vi "main_scan_4.vi"() -> ()   [LabVIEW 2009]
uses:
  <vilib>/userDefined/High Color/IMAQdx.ctl
  <vilib>/vision/Image Controls.llb/IMAQ Image.ctl
  global_stage_initialised.vi
  <vilib>/vision/driver/IMAQdx.llb/IMAQdx Buffer Number Mode.ctl
  <vilib>/Utility/file.llb/Write To Spreadsheet File (DBL).vi
  <vilib>/vision/driver/NI_Vision_Acquisition_Software.lvlib
  C:/Program Files (x86)/National Instruments/LabVIEW 2009/resource/objmgr/imaqdx.rc
panel:
  in  "Video Mode":u32(ring)=2 items=["Mono 8 1.88 fsp", "Mono 8 3.75 fsp", "Mono 8 7.50 fsp", "Mono 8 15.00 fsp", "Mono 8 30.00 fsp", "Mono 8 60.00 fsp", "Mono 8 120.00 fsp", "Mono 16 1.88 fsp", "Mono 16 3.75 fsp", "Mono 16 7.50 fsp", "Mono 16 15.00 fsp", "Mono 16 30.00 fsp", "Mono 16 60.00 fsp", "Format 7 Mode 0 640x480"]
  out "Vektor Summierte Helligkeit [a.u.]":dbl[](array[numeric])
  out "Vektor L/2-Position [°]":dbl[](array[numeric])
  out "Daten speichern":bool
  out "Leist/Pol # Schleifen":i64
  out "Leistungs-/Polarisationscan läuft":bool
  in  "Max. Spannungsdifferenz":dbl=150.0
  out "Geschätzte Messzeit":string="00:00"
  out "Start time [ms]":timestamp
  out "2D-Intensitätsverteilung (MCP)":dbl[][](graph)
  in  "# Photosignale":i32
  in  "Achs-ID":i32
  in  "Spannungskanal":refnum<k21>
  out "x-U-Scan läuft":bool
  out "Spannungsscan läuft":bool
  out "LAPD Spannung (V)":dbl format="%#.3g"
  out "Summierte Helligkeit (a.u.)":i64
  out "# Messschritte":i32
  out "Aktueller Messschritt":i32
  in  "LAPD-Daten speichern":bool
  in  "Summierte Helligkeit speichern":bool
  in  "Einzelbilder speichern":bool
  in  "Gemittelte Bilder speichern":bool
  in  "# Bilder/Messschritt":i32=1
  in  "SN von Rotationsbühne":i32=83831982
  in  "Wellenplatte [°]":refnum<k7>(container)
  out "Wellenplatte":bool
  in  "Waveplate ON/OFF":bool
  in  "Registerkarte":T1(tab)=enum."Leistungs-/Polarisationsscan"
  out "Aktuelle xyz-Position [mm]":dbl[](array[numeric]) format="%.5g"
  in  "Rasterweite [µm]":dbl[](array[numeric])
  in  "# Rasterschritte":i32[](array[numeric])=[1, 1, 1] min=1 step=1
  in  "Rasterung ON/OFF":bool
  out "Start xyz-Position [mm]":dbl[](array[numeric]) format="%.5g"
  in  "Rasterart":T2(ring)=enum."2D-Scan(xy)"
  out "Rasterschritt [µm]":dbl[](array[numeric])
  out "2D-Intensitätsverteilung (LAPD)":dbl[][](graph)
  out "Spannungsstart [V]":dbl[](array[numeric])
  out "TIP/SUP":string[](array[string])=["Tip", "Suppressor"]
  out "Spannungsschritt [V]":dbl[](array[numeric]) format="%.1g"
  out "Aktuelle Spannung [V]":dbl[](array[numeric]) format="%.1f"
  in  "# Spannungsschritte":i32[](array[numeric])
  in  "Spannungsweite [V]":dbl[](array[numeric])
  in  "Spannungsscan ON/OFF":bool
  out "Schräglage berücksichtigen":string="Schräglage berücksichtigen"
  in  "Ausgleichslage Start festlegen":bool
  out "x-U-Scan (Ausgleichslage) xy-Start [mm]":dbl[](array[numeric]) format="%_5g"
  in  "Raum-Koordinate 2 (Lagenausgleich)":enum16{"x-Achse", "y-Achse", "z-Achse"}(ring)=enum."y-Achse"
  out "x-U-Scan y-Startposition [mm]":dbl format="%.4g"
  out "x-U-Scan aktuelle y-Position [mm]":dbl format="%.4g"
  in  "x-U-Scan (Ausgleichslage) Steigung":dbl format="%_3g"
  out "x-U-Scan Spannungsstart [V]":dbl
  out "x-U-Scan Spannungsschritt [V]":dbl
  out "x-U-Scan aktuelle Spannung [V]":dbl
  in  "# x-U-Scan Spannungsschritte":i32
  in  "x-U-Scan Spannungsweite [V]":dbl
  in  "Raum-Koordinate 1":enum16{"x-Achse", "y-Achse", "z-Achse"}(ring)
  in  "Spannungs-Koordinate":enum16{"Tip-Spannung", "Suppressor-Spannung"}(ring)=2
  in  "x-U-Scan ON/OFF":bool
  in  "x-U-Scan x-Rasterweite [µm]":dbl
  in  "# x-U-Scan x-Rasterschritte":i32
  out "x-U-Scan x-Startposition [mm]":dbl format="%.4g"
  out "x-U-Scan aktuelle x-Position [mm]":dbl format="%.4g"
  out "x-U-Scan x-Rasterschritt [µm]":dbl
  out "x-U-Scan (Ausgleichslage) xy-End [mm]":dbl[](array[numeric]) format="%_5g"
  in  "Ausgleichslage Ende festlegen":bool
  in  "Sättigungszeit [s]":dbl
  in  "Wartezeit [s]":dbl
  in  "Max. Leistung (vK) [mW]":dbl
  out "Aktuelle Leistung (iK) [mW]":dbl
  out "Aktuelle L/2-Position [°]":dbl format="%_3g"
  out "L/2-Schritt [°]":dbl
  in  "Hin und Zurück":bool=TRUE
  in  "# L/2-Schritte":i32
  in  "L/2-Weite [°]":dbl
  in  "L/2-Start [°]":dbl
  in  "Leistuns- oder Polarisationsscan":u16(ring) items=["Polarisationsscan", "Leistungsscan"]
  in  "Leistungs-/Polarisationsscan ON/OFF":bool
  out "1D-Intensitätsverteilung (MCP)":T3(graph)
  out "Vorherige L/2 Position [°]":dbl format="%_3g"
  in  "Hintergrund-Helligkeit":i64
  in  "Helligkeit nullen":bool
  out "Helligkeitsverlauf":dbl(graph)
  in  "Sequenz Ordner":string="Referenzbilder"
  in  "Sequenzaufnahme ON":bool
  in  "MCP-Spannung [V]":dbl=1300.0
  in  "P-Schirm-Spannung [V]":dbl=4300.0
  in  "Proben-ID":string="140528_06"
  out "Messlogbuch":path
  out "Gemitteltes Bild":u64[][](array[numeric])
  in  "Polarisation [°]":dbl=90.0
  out "Current y step":i32
  out "Current z step":i32
  out "Current x step":i32
  out "Scanschleifenzähler":i32
  out "Kameraschleifenzähler":i32
  out "Steuerschleifenzähler":i32
  out "Bühne":bool
  in  "HV ON/OFF":bool
  out "HV-Steuerung":bool
  in  "Suppressor-Spannung [V]":dbl min=0.0 max=1000.0 step=1.0 format="%.1p"
  in  "Tip-Spannung [V]":dbl min=0.0 max=800.0 step=1.0 format="%.1p"
  in  "Leistung (iK) [mW]":dbl format="%.1f"
  in  "LAPD-Kanal (Meilhaus)":u32 max=31
  out "Save folder":string
  out "Buffer Number":u64
  out "ROI table":string[](array[string])=["Breite [px]", "Höhe [px]", "X-Offset [px]", "Y-Offset [px]"]
  in  "Vollbild":bool
  out "Frame Rate (FPS)":dbl format="%#_3g"
  in  "Buffer Interval":u32=1
  out "Ereignis: FrameDone?":refnum<event-registration>
  out "Image Display":T4(plugin-control)
  in  "ROI":i32[](array[numeric])=[640, 480, 0, 0]
  in  "Shutter time (ms)":u16(ring)=3 items=["1000", "500", "200", "100", "50", "20", "10", "1"]
  out "Buffer Overrun":bool
  out "Image Memory":T4
  out "Kamera":bool
  in  "Kamera ON/OFF":bool
  in  "Detektionskamera":T5="cam0"
  out "Day folder":string
  in  "Root folder":string="E:\\GIPES\\Messungen\\"
  out "z-Achse":i32=3
  out "y-Achse":i32=2
  out "x-Achse":i32=1
  out "Event: Rasterung gestartet?":refnum<user-event>
  out "Fehler (Ausgang)":errorcluster
  in  "Programm beenden":bool
  out "Rasterung läuft":bool
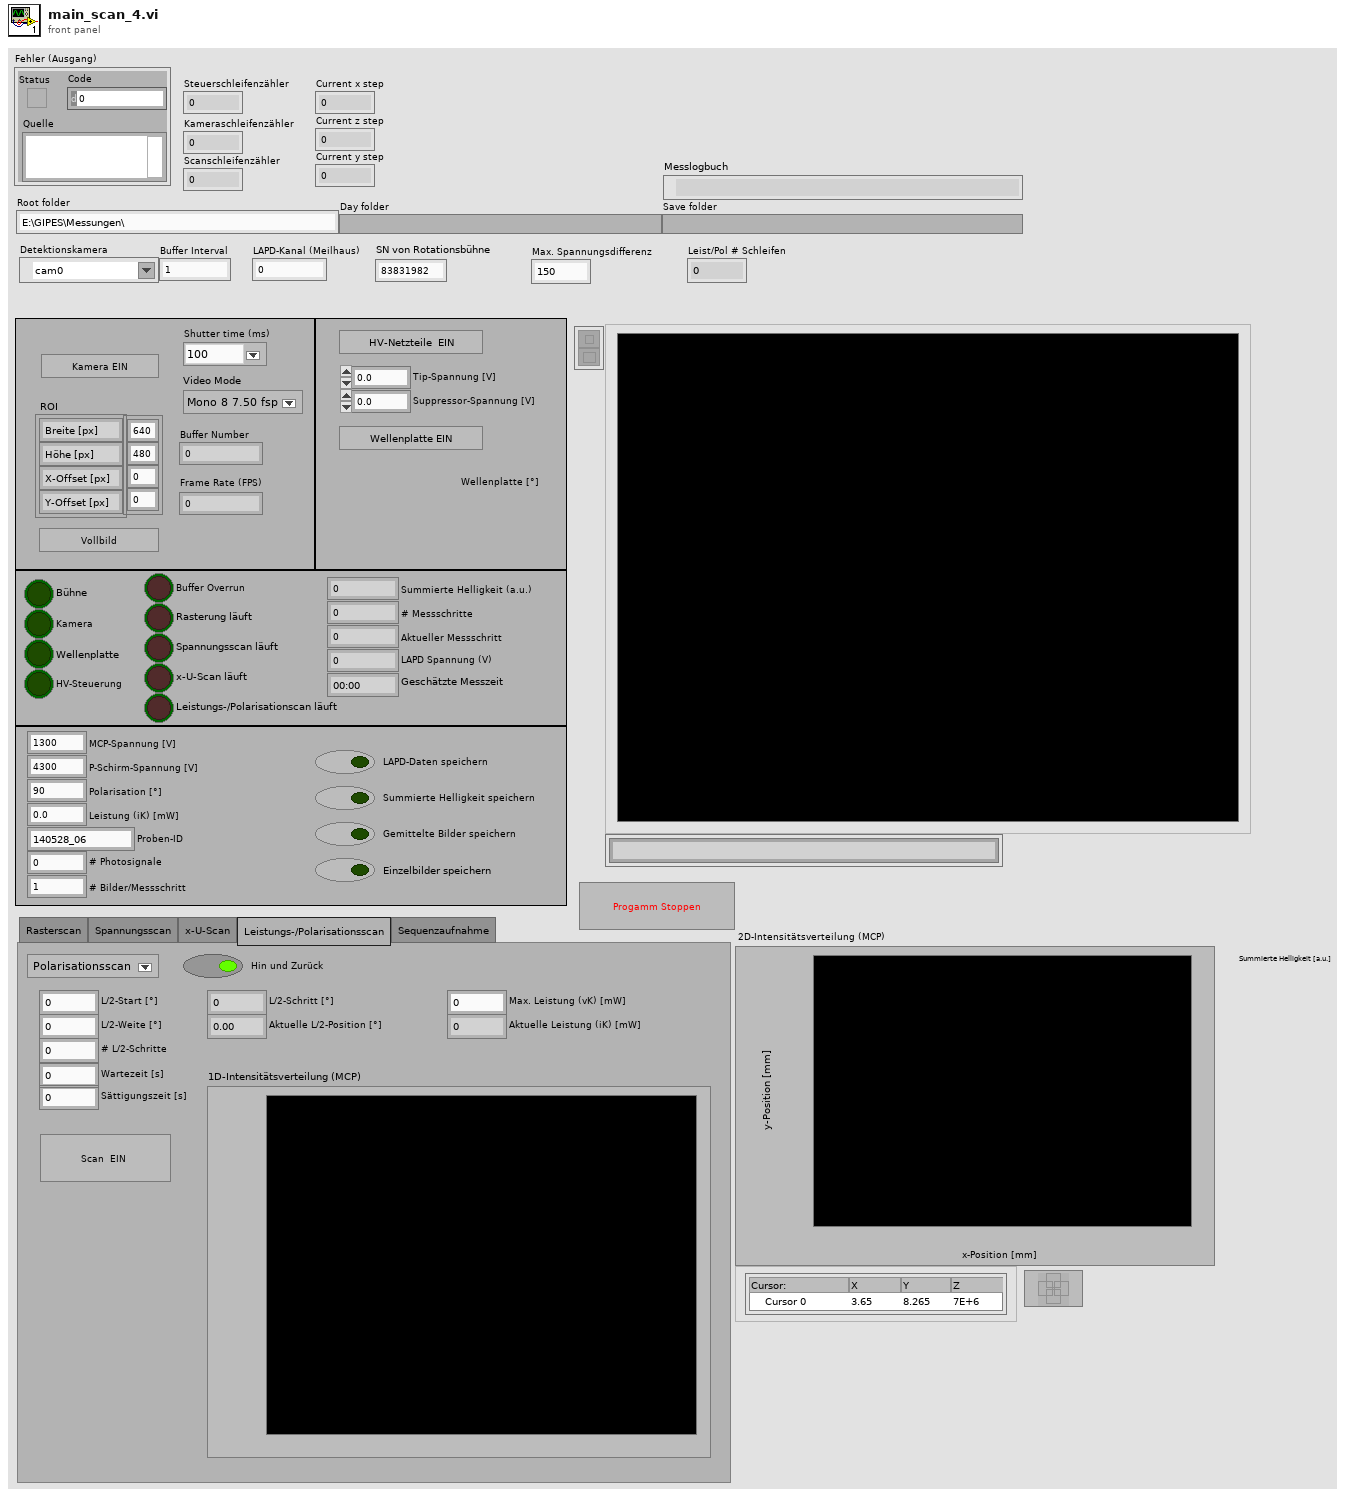
[diagram p1: front panel]
types:
  T1 = enum32{"Rasterscan", "Spannungsscan", "x-U-Scan", "Leistungs-/Polarisationsscan", "Sequenzaufnahme"}
  T2 = enum16{"Linescan(x)", "Linescan(z)", "2D-Scan(xy)", "2D-Scan(yz)", "2D-Scan(xz)"}
  T3 = cluster{"Vektor L/2-Position [°]":dbl[], "Vektor Summierte Helligkeit [a.u.]":dbl[]}
  T4 = typedef "IMAQ Image.ctl" = refnum<image>
  T5 = typedef "IMAQdx.ctl" = refnum<k21>
  T6 = enum32{"Bad", "Idle", "Run top level", "Running"}
  T7 = cluster{"Summierte Helligkeit (a.u.)":u64, "Aktuelle L/2-Position [°]":dbl}
  T8 = typedef "NI_Vision_Acquisition_Software.lvlib/IMAQdx Buffer Number Mode.ctl" = enum32{"Next", "Last", "Buffer Number"}
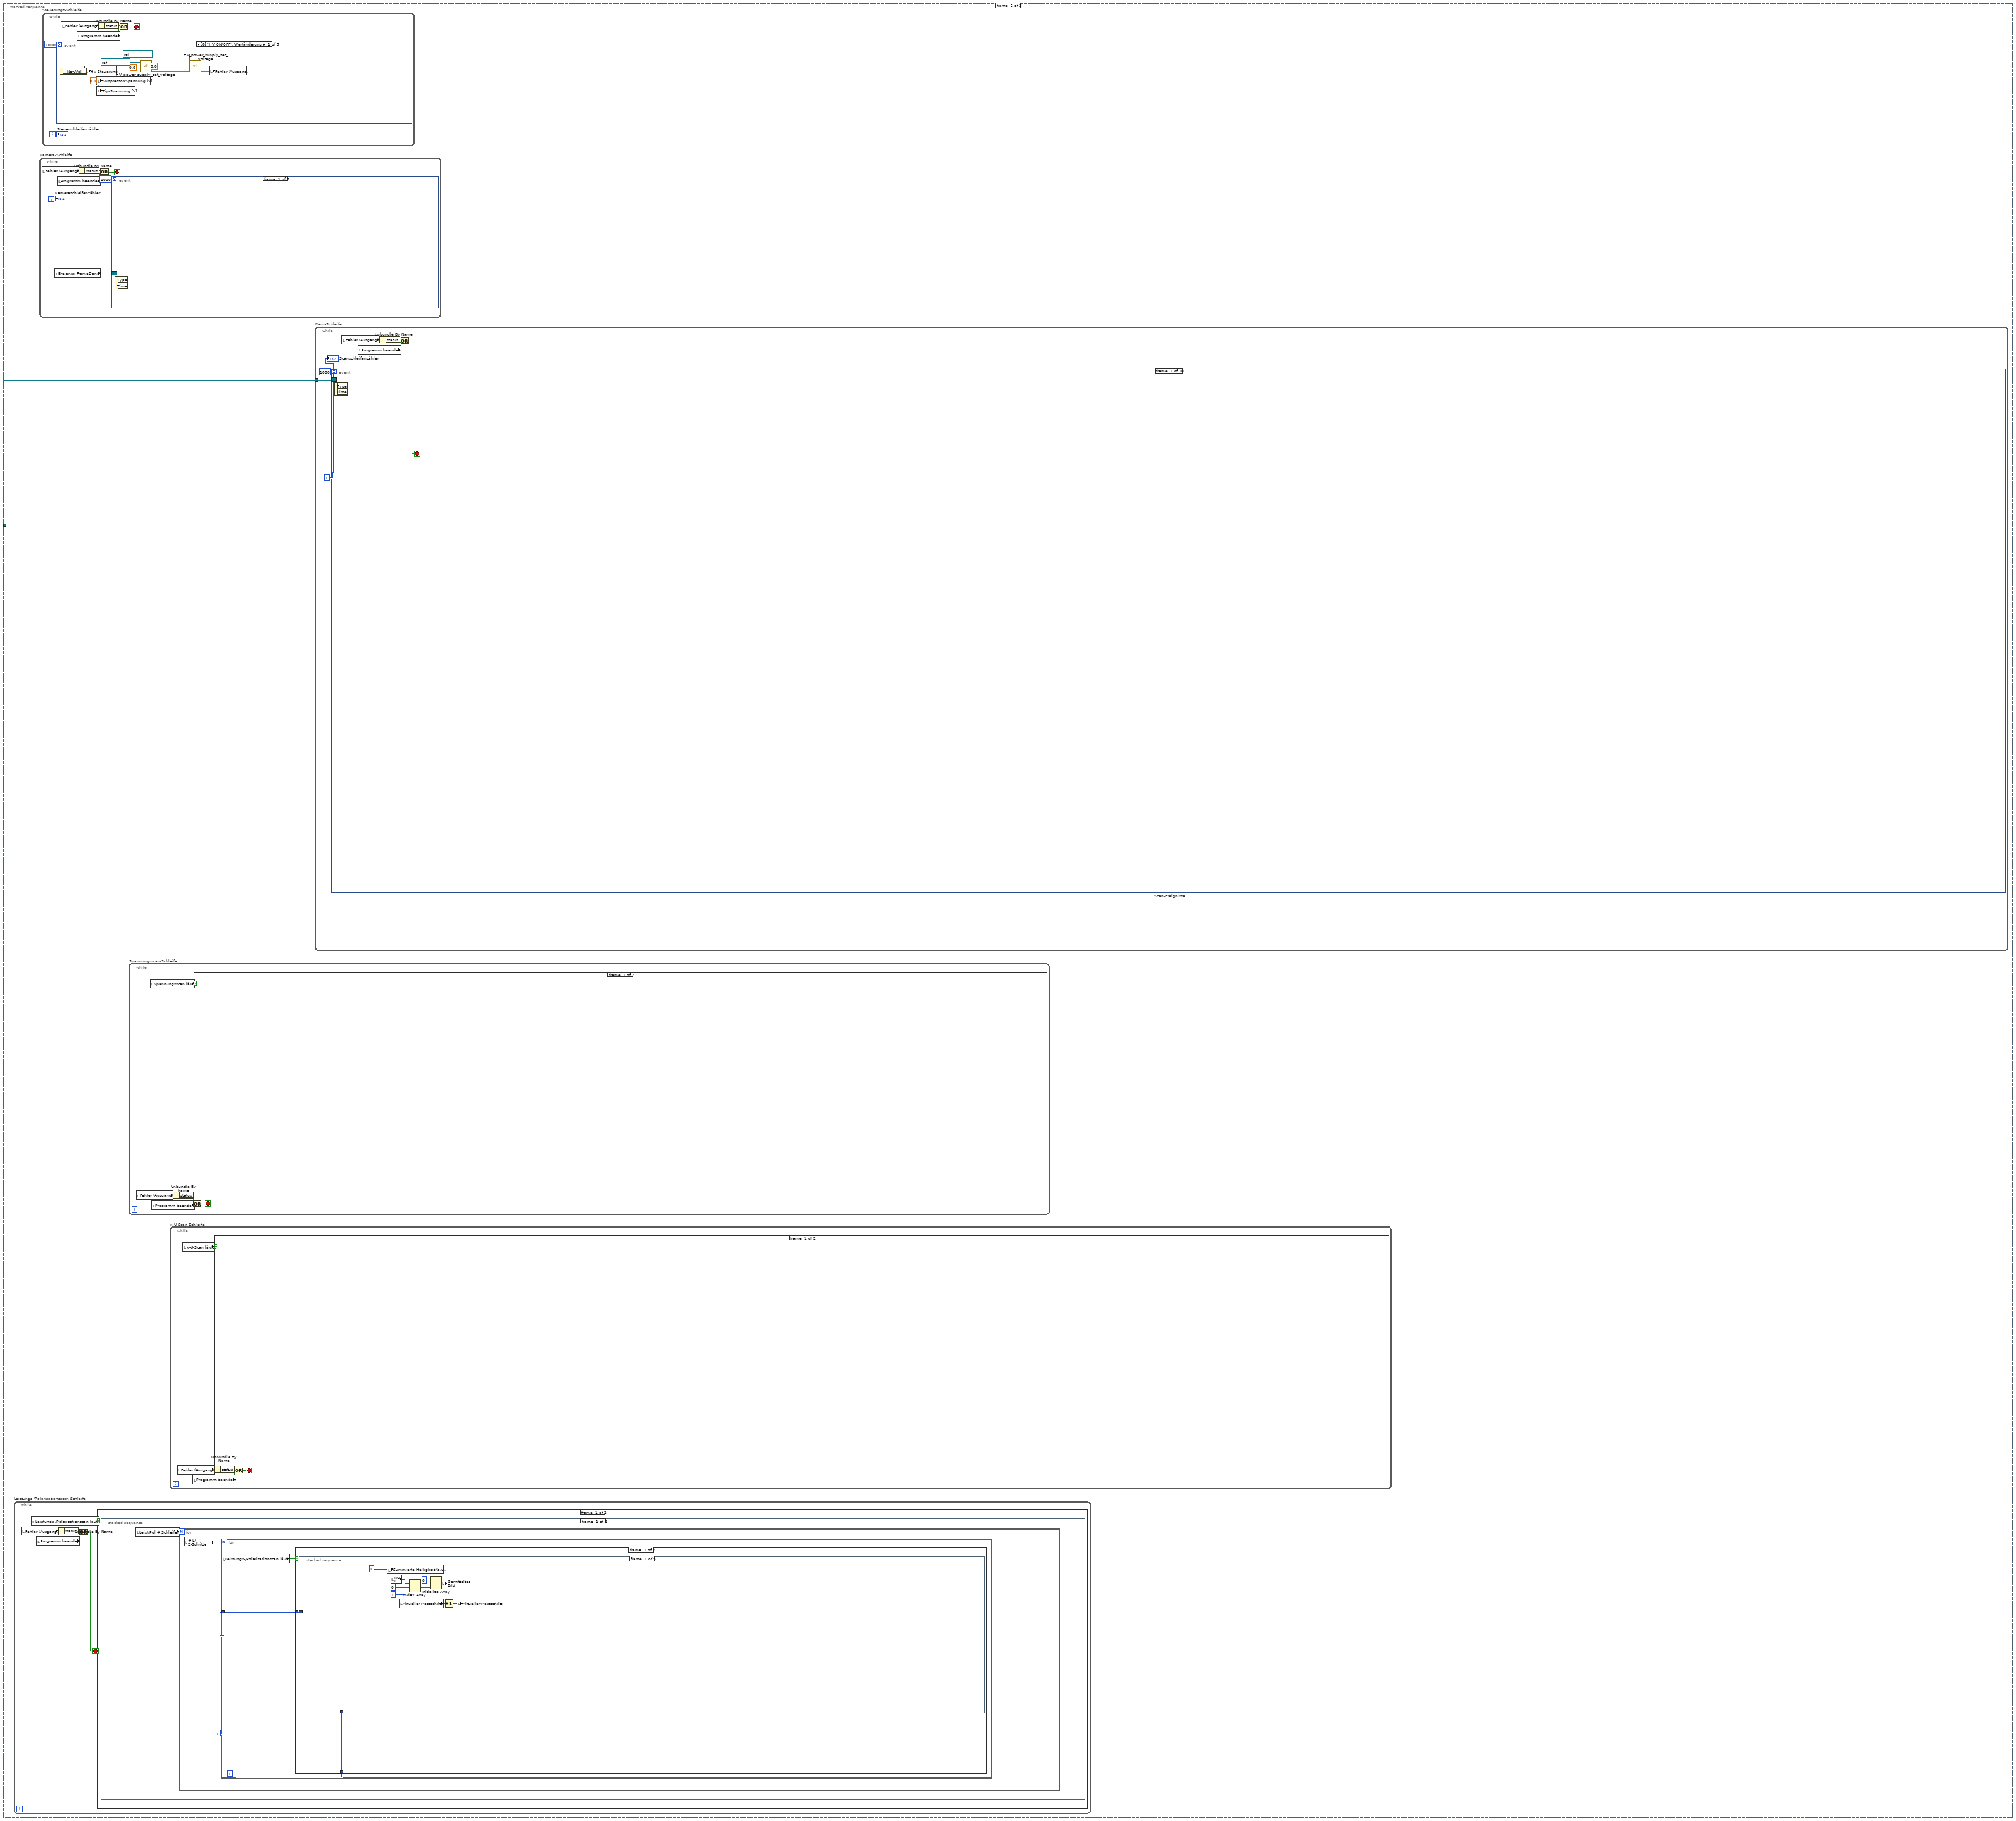
[diagram p3: hidden frame]
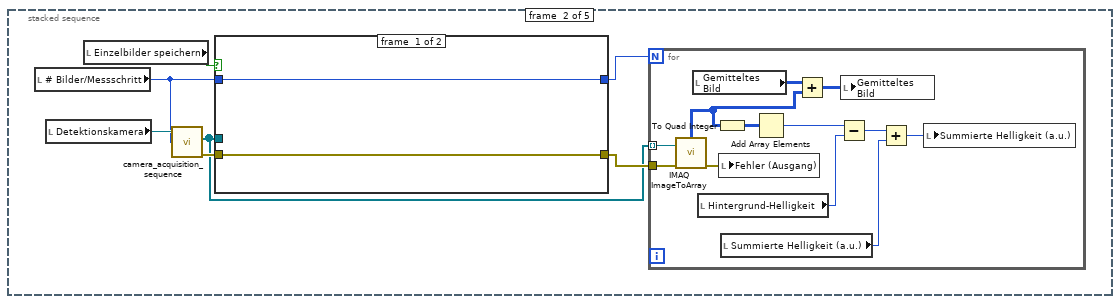
[diagram p4: hidden frame]
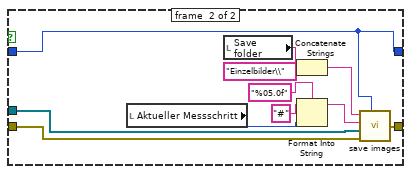
[diagram p5: hidden frame]
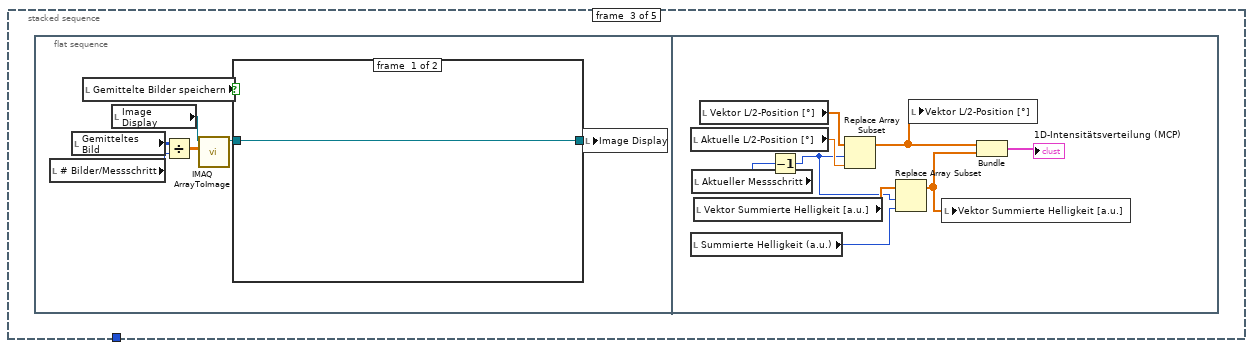
[diagram p6: hidden frame]
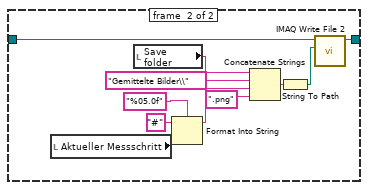
[diagram p7: hidden frame]
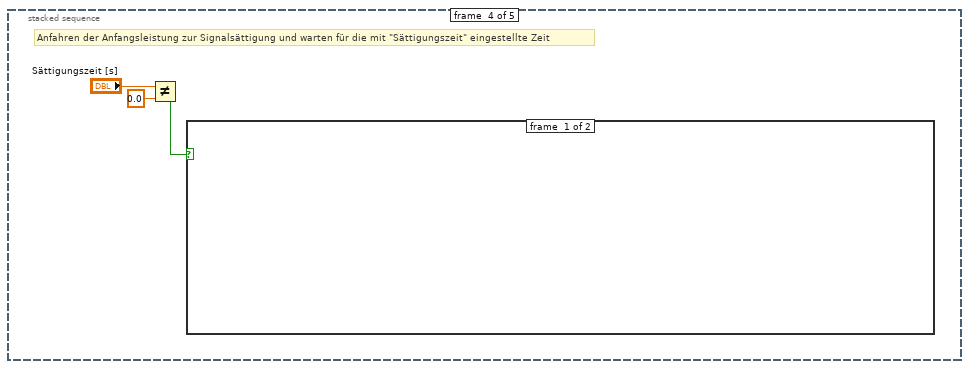
[diagram p8: hidden frame]
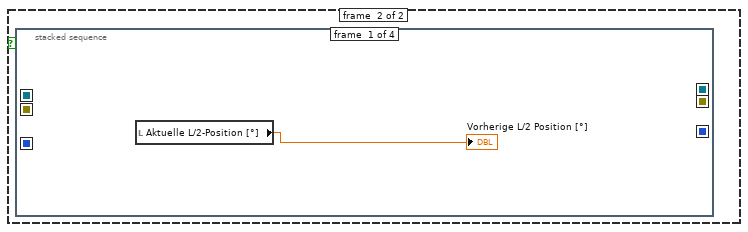
[diagram p9: hidden frame]
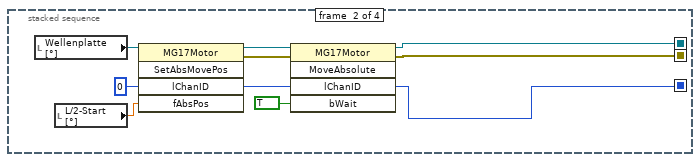
[diagram p10: hidden frame]
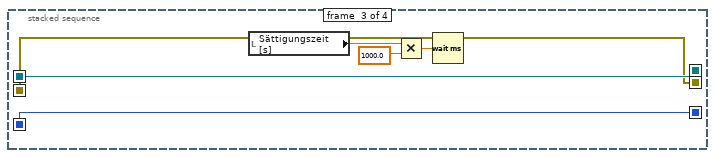
[diagram p11: hidden frame]
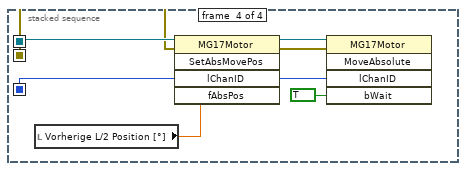
[diagram p12: hidden frame]
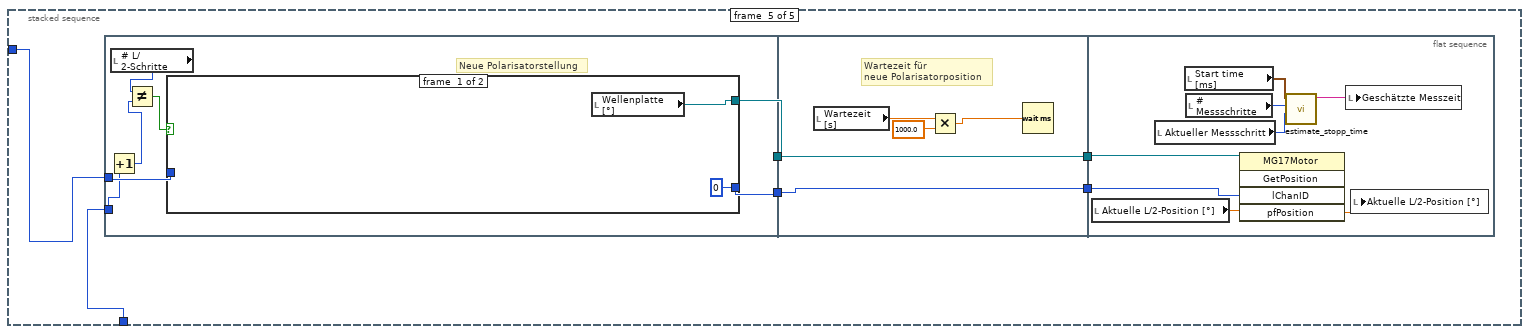
[diagram p13: hidden frame]
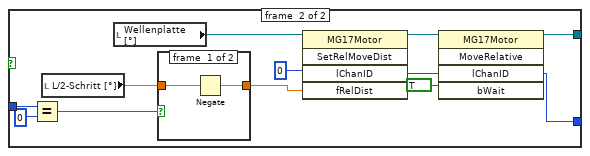
[diagram p14: hidden frame]
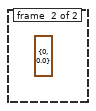
[diagram p16: hidden frame]
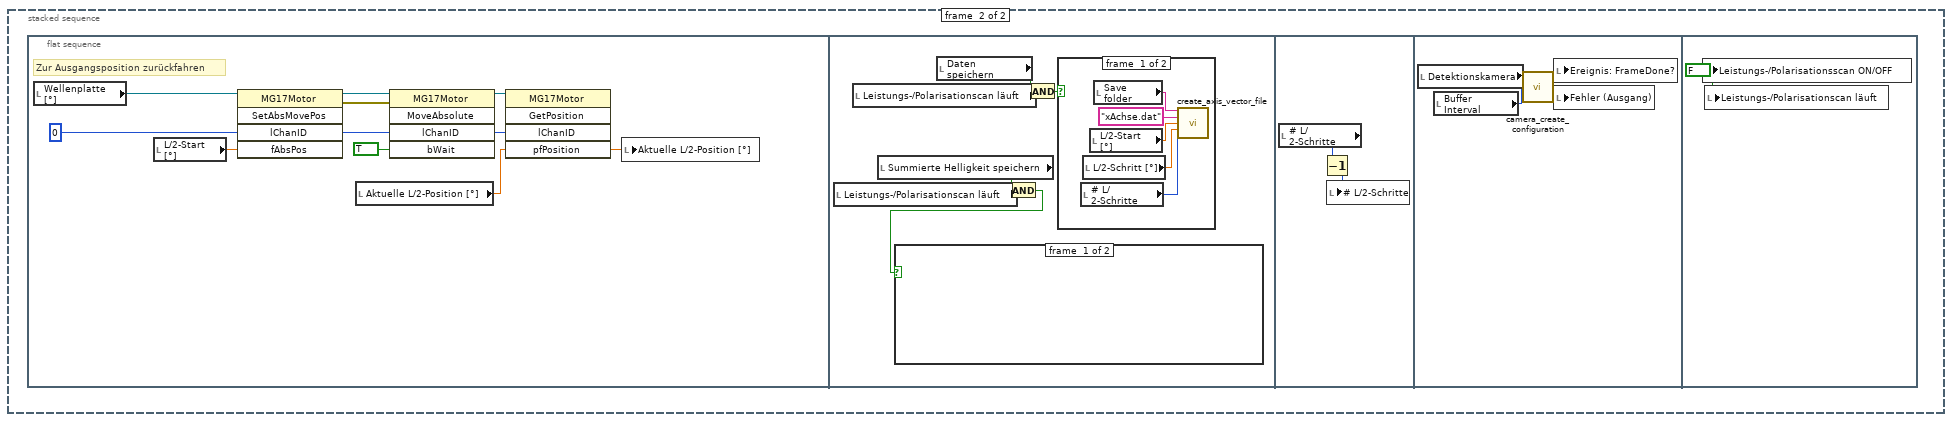
[diagram p17: hidden frame]
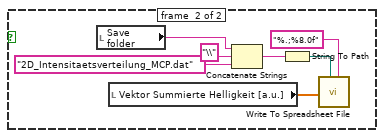
[diagram p18: hidden frame]
diagram:
  n1 = local read "Event: Rasterung gestartet?"() -> (w2:refnum<user-event>)
  n2 = register-events(w2) -> (reference out=w1:refnum<event-registration>)  [unwired: 2 in, 1 out]
  n3 = flat-sequence {
    frame #0 {
      (unwired) 0.0 ("Helligkeitsverlauf")
      w6 = 0.0 ("Aktuelle x-Position [mm]")
      w12 = 1 ("# x-U-Scan Spannungsschritte")
      w13 = 0.0 ("Aktuelle x-Position [mm]")
      w11 = 0.0 ("Suppressor-Spannung [V]")
      w3 = i64 0 ("Numerisches Element")
      w25 = u16 3 items=["1000", "500", "200", "100", "50", "20", "10"] ("Shutter time (ms)")
      w4 = FALSE ("Scanstart")
      n4 = Initialize Array(1 ("Element"), 2 ("Dimension")) -> (w14:i32[])
      n5 = Initialize Array(1 ("Dimension"), 3 ("Dimension")) -> (w37:i32[])
      n6 = Initialize Array(0.0 ("Element"), 2 ("Dimension")) -> (w10:dbl[])
      "Aktuelle Spannung [V]" <- w10
      "Spannungsstart [V]" <- w10
      "x-U-Scan (Ausgleichslage) xy-Start [mm]" <- w10
      "x-U-Scan (Ausgleichslage) xy-End [mm]" <- w10
      n7 = Initialize Array(0.0 ("Element"), 3 ("Dimension")) -> (w20:dbl[])
      "Aktuelle xyz-Position [mm]" <- w20
      "Start xyz-Position [mm]" <- w20
      "Rasterschritt [µm]" <- w20
      n8 = local write "Tip-Spannung [V]"(0.0 ("Tip-Spannung [V]")) -> ()
      n9 = local write "# Photosignale"(10.0 ("Anzahl Mittelungen")) -> ()
      n10 = local write "x-U-Scan x-Rasterweite [µm]"(w11) -> ()
      n11 = local write "# x-U-Scan x-Rasterschritte"(w12) -> ()
      n12 = local write "x-U-Scan Spannungsweite [V]"(w11) -> ()
      n13 = local write "# x-U-Scan Spannungsschritte"(w12) -> ()
      n14 = local write "Suppressor-Spannung [V]"(w11) -> ()
      n15 = local read "Aktueller Messschritt"() -> (w30:i32)
      n16 = local write "Shutter time (ms)"(w25) -> ()
      n17 = local write "# Spannungsschritte"(w14) -> ()
      n18 = local write "Spannungsweite [V]"(w10) -> ()
      n19 = local write "Rasterweite [µm]"(w20) -> ()
      n20 = local write "# Rasterschritte"(w37) -> ()
      n21 = local write "ROI"(i32[] [640, 480, 0, 0] ("Region of Interest (px)")) -> ()
      n22 = local write "x-U-Scan (Ausgleichslage) Steigung"(0.0 ("x-U-Scan (Ausgleichslage) Steigung")) -> ()
      n23 = local write "Spannungsscan ON/OFF"(w4) -> ()
      n24 = local write "Programm beenden"(w4) -> ()
      n25 = local write "Spannungsscan ON/OFF"(w4) -> ()
      n26 = local write "Sequenzaufnahme ON"(w4) -> ()
      n27 = local write "HV ON/OFF"(w4) -> ()
      n28 = local write "x-U-Scan ON/OFF"(w4) -> ()
      n29 = local write "Kamera ON/OFF"(w4) -> ()
      n30 = local write "Rasterung ON/OFF"(w4) -> ()
      n31 = local write "Waveplate ON/OFF"(w4) -> ()
      n32 = local write "Buffer Overrun"(w4) -> ()
      n33 = local write "x-U-Scan läuft"(w4) -> ()
      n34 = local write "Rasterung läuft"(w4) -> ()
      n35 = Create User Event(user event datatype=w30) -> (user event=→"Event: Rasterung gestartet?":refnum<user-event>)  [unwired: 1 in, 1 out]
      n36 = local write "Leistungs-/Polarisationsscan ON/OFF"(w4) -> ()
      n37 = local write "Hintergrund-Helligkeit"(w3) -> ()
      "Rasterung läuft" <- FALSE ("Scan aktiv")
      "# Messschritte" <- 0 ("# Messschritte")
      "Aktueller Messschritt" <- 0 ("Aktueller Messschritt")
      "x-Achse" <- 1 ("x-Achse")
      "y-Achse" <- 2 ("y-Achse")
      "z-Achse" <- 3 ("z-Achse")
      "Summierte Helligkeit (a.u.)" <- w3
      "LAPD Spannung (V)" <- 0.0 ("Transmittierte Intensität (a.u.)")
      "Bühne" <- w4
      "Wellenplatte" <- w4
      "Kamera" <- FALSE ("Camera eingeschaltet")
      "HV-Steuerung" <- w4
      "Spannungsscan läuft" <- w4
      "x-U-Scan aktuelle x-Position [mm]" <- w13
      "x-U-Scan x-Rasterschritt [µm]" <- w13
      "x-U-Scan aktuelle Spannung [V]" <- w13
      "x-U-Scan Spannungsschritt [V]" <- w13
      "x-U-Scan x-Startposition [mm]" <- w13
      "x-U-Scan Spannungsstart [V]" <- w11
      "x-U-Scan aktuelle y-Position [mm]" <- 0.0 ("x-U-Scan aktuelle y-Position [mm]")
      "x-U-Scan y-Startposition [mm]" <- 0.0 ("x-U-Scan y-Startposition [mm]")
      "L/2-Schritt [°]" <- w6
      "Aktuelle L/2-Position [°]" <- w6
      "Aktuelle Leistung (iK) [mW]" <- w6
      "Leistungs-/Polarisationscan läuft" <- w4
      "Leist/Pol # Schleifen" <- i64 1 ("Leist/Pol # Schleifen")
      "Daten speichern" <- w4
    }
  }
  n38 = stacked-sequence {
    tunnel: w1 -> [_ w63 _]
    frame #0 {
      n39 = flat-sequence {
        frame #0 {
          # "Überprüfung ob die VI stage_control.vi ausgeführt wid, wenn nicht wird sie gestartet und gewartet bis die Bühne initialisiert ist"
          n40 = Open VI Reference(vi path=path "stage_control.vi" ("VI-Pfad")) -> (vi reference=w41:refnum<vi>)  [unwired: 5 in, 1 out]
          n41 = property class="VI"(reference=w41) -> (reference out=w40:refnum<vi>, error out=w39:errorcluster, "Exec.State"=w44:T6)  [unwired: 1 in]
          n42 = Equal?(x=w44, y=T6."Run top level") -> (x = y?=w42:bool)
          n43 = case shown="False" w42 {
            tunnel: w40 -> [w51 _]
            tunnel: w39 -> [w50 _]
            frame #0 {
              n44 = invoke class="VI" method="VI ausführen"(reference=w51, error in=w50, "Wait until done"=FALSE ("Warten bis beendet"), "Auto Dispose Ref"=FALSE ("Referenz automatisch schließen")) -> (reference out=w47:refnum<vi>)  [unwired: 1 in, 4 out]
              n45 = invoke class="VI" method="FP.Öffnen"(reference=w47) -> (reference out=w46:refnum<vi>)  [unwired: 4 in, 4 out]
              n46 = while {
                tunnel: w46 -> [w58]
                stop <- w53 stop-if-true
                n47 = property class="VI"(reference=w58) -> (error out=w57:errorcluster, "Exec.State"=w56:T6)  [unwired: 1 in, 1 out]
                n48 = global read "global_stage_initialised.vi" "Bühne initialisiert"() -> (w52:bool)
                n49 = local write "Fehler (Ausgang)"(w57) -> ()
                n50 = Equal?(x=w56, y=T6."Run top level") -> (x = y?=w54:bool)
                n51 = And(x=w52, y=w54) -> (x .and. y?=w53:bool)
              }
            }
            frame #1 {
            }
          }
        }
        frame #1 {
          n52 = local read "Root folder"() -> (w62:string)
          n53 = local write "Bühne"(TRUE ("Bühne bereit")) -> ()
          n54 = call "create_day_folder.vi"("Root folder"=w62) -> ("Day Folder"=w60:string)  [unwired: 9 in, 1 out]
          n55 = local write "Day folder"(w60) -> ()
          n56 = call "create_measure_log_file.vi"("Tagesordner"=w60) -> ("Messlogbuch"=w59:path)  [unwired: 9 in]
          n57 = local write "Messlogbuch"(w59) -> ()
        }
      }
    }
    frame #1 {
      n58 = while "Leistungs-/Polarisationsscan-Schleife" {
        stop <- w65 stop-if-true
        n59 = local read "Fehler (Ausgang)"() -> (w68:errorcluster)
        n60 = local read "Leistungs-/Polarisationscan läuft"() -> (w64:bool)
        n61 = local read "Programm beenden"() -> (w66:bool)
        n62 = Unbundle By Name(w68) -> ("status"=w67:bool)
        n63 = Or(x=w67, y=w66) -> (x .or. y?=w65:bool)
        n64 = case shown="True" w64 {
          frame #0 {
            n65 = stacked-sequence {
              frame #0 {
                n66 = local read "Leist/Pol # Schleifen"() -> (w69:i64)
                n67 = for {
                  N: w69 -> [_]
                  i -> [w70]
                  n68 = local read "# L/2-Schritte"() -> (w71:i32)
                  n69 = for "Schleife für L/2-Position" {
                    N: w71 -> [_]
                    tunnel: w70 -> [w73]
                    i -> [w72]
                    n70 = local read "Leistungs-/Polarisationscan läuft"() -> (w74:bool)
                    n71 = case shown="True" w74 {
                      tunnel: w73 -> [w76 _]
                      tunnel: w72 -> [w75 _]
                      frame #0 {
                        n72 = stacked-sequence {
                          tunnel: w76 -> [_ _ _ _ w180]
                          tunnel: w75 -> [_ _ _ _ w175]
                          frame #0 {
                            n73 = local write "Summierte Helligkeit (a.u.)"(u64 0 ("Summierte Helligkeit (a.u.)")) -> ()
                            n74 = local read "ROI"() -> (w82:i32[])
                            n75 = local read "Aktueller Messschritt"() -> (w79:i32)
                            n76 = Index Array(array=w82, index #1=0 ("Index"), index #2=1 ("Index")) -> (element #1=w86:i32, element #2=w85:i32)
                            n77 = Initialize Array(u64 0 ("Element"), w85, w86) -> (w80:u64[][])
                            n78 = local write "Gemitteltes Bild"(w80) -> ()
                            n79 = Increment(x=w79) -> (x+1=w78:i32)
                            n80 = local write "Aktueller Messschritt"(w78) -> ()
                          }
                          frame #1 {
                            n81 = local read "# Bilder/Messschritt"() -> (w90:i32)
                            n82 = local read "Detektionskamera"() -> (w93:T5)
                            n83 = local read "Einzelbilder speichern"() -> (w88:bool)
                            n84 = call "camera_acquisition_sequence.vi"("Session In"=w93, "Desired image number"=w90) -> ("Image Array"=w87:T4[], "error out"=w92:errorcluster)  [unwired: 2 in, 1 out]
                            n85 = case shown="True" w88 {
                              tunnel: w92 -> [w95 w103]
                              tunnel: [w95 w102] -> w91
                              tunnel: w90 -> [w94 w101]
                              tunnel: [w94 w101] -> w89
                              tunnel: w87 -> [_ w100]
                              frame #0 {
                              }
                              frame #1 {
                                n86 = local read "Aktueller Messschritt"() -> (w106:i32)
                                n87 = local read "Save folder"() -> (w98:string)
                                n88 = Concatenate Strings(w98, "Einzelbilder\\" ("String")) -> (w96:string)
                                n89 = Format Into String(format string="%05.0f" ("Format-String"), initial string="#" ("Eingangs-String"), w106) -> (resulting string=w99:string)  [unwired: 1 in, 1 out]
                                n90 = call "save images.vi"("Save Folder"=w96, "File name prefix"=w99, "Array"=w100, "error out 2"=w103, "Bilder/Messschritt"=w101) -> ("error out"=w102:errorcluster)
                              }
                            }
                            n91 = for {
                              N: w89 -> [_]
                              tunnel: w91 -> [w116]
                              tunnel: w87 -> [w114] mode=indexing
                              n92 = call "IMAQ ImageToArray"("error in (no error)"=w116, "Image"=w114) -> ("error out"=w115:errorcluster, "Image Pixels (U8)"=w113:u8[][])  [unwired: 2 in, 3 out]
                              n93 = local read "Gemitteltes Bild"() -> (w111:u64[][])
                              n94 = local read "Hintergrund-Helligkeit"() -> (w107:i64)
                              n95 = To Quad Integer(1:w113) -> (0:w117:i64[][])
                              n96 = local write "Fehler (Ausgang)"(w115) -> ()
                              n97 = local read "Summierte Helligkeit (a.u.)"() -> (w110:i64)
                              n98 = Add Array Elements(numeric array=w117) -> (sum=w109:i64)
                              n99 = Add(x=w111, y=w113) -> (x+y=w112:u64[][])
                              n100 = Subtract(x=w109, y=w107) -> (x-y=w108:i64)
                              n101 = local write "Gemitteltes Bild"(w112) -> ()
                              n102 = Add(x=w108, y=w110) -> (x+y=w118:i64)
                              n103 = local write "Summierte Helligkeit (a.u.)"(w118) -> ()
                            }
                          }
                          frame #2 {
                            n104 = flat-sequence {
                              frame #0 {
                                n105 = local read "# Bilder/Messschritt"() -> (w121:i32)
                                n106 = local read "Gemitteltes Bild"() -> (w119:u64[][])
                                n107 = local read "Gemittelte Bilder speichern"() -> (w125:bool)
                                n108 = local read "Image Display"() -> (w123:T4)
                                n109 = Divide(x=w119, y=w121) -> (x/y=w120:dbl[][])
                                n110 = call "IMAQ ArrayToImage"("Image Pixels (U8)"=w120, "Image"=w123) -> ("Image Out"=w122:T4)  [unwired: 8 in, 1 out]
                                n111 = case shown="True" w125 {
                                tunnel: w122 -> [w126 w137]
                                tunnel: [w126 w128] -> w124
                                frame #0 {
                                }
                                frame #1 {
                                n112 = local read "Aktueller Messschritt"() -> (w132:i32)
                                n113 = local read "Save folder"() -> (w134:string)
                                n114 = Format Into String(format string="%05.0f" ("Format-String"), initial string="#" ("Eingangs-String"), w132) -> (resulting string=w131:string)  [unwired: 1 in, 1 out]
                                n115 = Concatenate Strings(w134, "Gemittelte Bilder\\" ("String"), w131, ".png" ("String")) -> (w130:string)
                                n116 = String To Path(string=w130) -> (path=w129:path)
                                n117 = call-poly "IMAQ Write File 2"("File Path"=w129, "Image"=w137) -> ("Image Out (duplicate)"=w128:T4)  [unwired: 8 in, 1 out]
                                }
                                }
                                n118 = local write "Image Display"(w124) -> ()
                              }
                              frame #1 {
                                n119 = local read "Aktuelle L/2-Position [°]"() -> (w143:dbl)
                                n120 = local read "Summierte Helligkeit (a.u.)"() -> (w142:i64)
                                n121 = local read "Aktueller Messschritt"() -> (w141:i32)
                                n122 = local read "Vektor Summierte Helligkeit [a.u.]"() -> (w145:dbl[])
                                n123 = local read "Vektor L/2-Position [°]"() -> (w144:dbl[])
                                n124 = Decrement(x=w141) -> (x-1=w140:i32)
                                n125 = Replace Array Subset(array=w144, new element=w143, index=w140) -> (w139:dbl[])
                                n126 = Replace Array Subset(array=w145, new element=w142, index=w140) -> (w138:dbl[])
                                n127 = local write "Vektor L/2-Position [°]"(w139) -> ()
                                n128 = local write "Vektor Summierte Helligkeit [a.u.]"(w138) -> ()
                                n129 = Bundle("Vektor L/2-Position [°]"=w139, "Vektor Summierte Helligkeit [a.u.]"=w138) -> (→"1D-Intensitätsverteilung (MCP)":T3)  [unwired: 1 in]
                              }
                            }
                          }
                          frame #3 {
                            # "Anfahren der Anfangsleistung zur Signalsättigung und warten für die mit \"Sättigungszeit\" eingestellte Zeit"
                            n130 = Not Equal?(x="Sättigungszeit [s]", y=0.0) -> (x != y?=w149:bool)
                            n131 = case shown="True" w149 {
                              frame #0 {
                              }
                              frame #1 {
                                n132 = stacked-sequence {
                                seq-local: [_ w153 _ _] -> [_ _ w163 _]
                                seq-local: [_ w152 _ _] -> [_ _ w162 _]
                                seq-local: [_ w151 _ _] -> [_ _ w161 _]
                                seq-local: [_ _ w163 _] -> [_ _ _ w170]
                                seq-local: [_ _ w162 _] -> [_ _ _ w169]
                                seq-local: [_ _ w161 _] -> [_ _ _ w168]
                                frame #0 {
                                n133 = local read "Aktuelle L/2-Position [°]"() -> (→"Vorherige L/2 Position [°]":dbl)
                                }
                                frame #1 {
                                n134 = local read "Wellenplatte [°]"() -> (w154:refnum<k7>)
                                n135 = local read "L/2-Start [°]"() -> (w160:dbl)
                                n136 = invoke class="MG17Motor" method="SetAbsMovePos"(reference=w154, "lChanID"=0, "fAbsPos"=w160) -> (reference out=w156:refnum<k7>, error out=w159:errorcluster, "lChanID"=w158:i32)  [unwired: 2 in, 2 out]
                                n137 = invoke class="MG17Motor" method="MoveAbsolute"(reference=w156, error in=w159, "lChanID"=w158, "bWait"=TRUE) -> (reference out=w152:refnum<k7>, error out=w151:errorcluster, "lChanID"=w153:i32)  [unwired: 1 in, 2 out]
                                }
                                frame #2 {
                                n138 = local read "Sättigungszeit [s]"() -> (w166:dbl)
                                n139 = Multiply(x=w166, y=1000.0) -> (x*y=w164:dbl)
                                n140 = Wait (ms)(milliseconds to wait=w164) -> ()  [unwired: 1 out]
                                }
                                frame #3 {
                                n141 = local read "Vorherige L/2 Position [°]"() -> (w167:dbl)
                                n142 = invoke class="MG17Motor" method="SetAbsMovePos"(reference=w169, error in=w168, "lChanID"=w170, "fAbsPos"=w167) -> (reference out=w172:refnum<k7>, error out=w174:errorcluster, "lChanID"=w173:i32)  [unwired: 1 in, 2 out]
                                n143 = invoke class="MG17Motor" method="MoveAbsolute"(reference=w172, error in=w174, "lChanID"=w173, "bWait"=TRUE) -> ()  [unwired: 1 in, 5 out]
                                }
                                }
                              }
                            }
                          }
                          frame #4 {
                            n144 = flat-sequence {
                              tunnel: w180 -> [w187]
                              tunnel: [w186] -> w179
                              tunnel: [w185] -> w178
                              tunnel: w175 -> [w184]
                              tunnel: w179 -> [w208]
                              tunnel: w178 -> [w209]
                              tunnel: [w209] -> w177
                              tunnel: [w208] -> w176
                              tunnel: w177 -> [w213]
                              tunnel: w176 -> [w212]
                              frame #0 {
                                # "Neue Polarisatorstellung"
                                n145 = Increment(x=w184) -> (x+1=w183:i32)
                                n146 = local read "# L/2-Schritte"() -> (w182:i32)
                                n147 = Not Equal?(x=w182, y=w183) -> (x != y?=w181:bool)
                                n148 = case shown="True" w181 {
                                tunnel: w187 -> [_ w194]
                                tunnel: [0 ("lChanID") w191] -> w186
                                tunnel: [w189 w190] -> w185
                                frame #0 {
                                n149 = local read "Wellenplatte [°]"() -> (w189:refnum<k7>)
                                }
                                frame #1 {
                                n150 = Equal?(x=w194, y=0) -> (x = y?=w192:bool)
                                n151 = local read "L/2-Schritt [°]"() -> (w196:dbl)
                                n152 = local read "Wellenplatte [°]"() -> (w197:refnum<k7>)
                                n153 = case shown="False" w192 {
                                tunnel: w196 -> [w203 w204]
                                tunnel: [w202 w204] -> w195
                                frame #0 {
                                n154 = Negate(x=w203) -> (-x=w202:dbl)
                                }
                                frame #1 {
                                }
                                }
                                n155 = invoke class="MG17Motor" method="SetRelMoveDist"(reference=w197, "lChanID"=0, "fRelDist"=w195) -> (reference out=w199:refnum<k7>, "lChanID"=w200:i32)  [unwired: 2 in, 3 out]
                                n156 = invoke class="MG17Motor" method="MoveRelative"(reference=w199, "lChanID"=w200, "bWait"=TRUE) -> (reference out=w190:refnum<k7>, "lChanID"=w191:i32)  [unwired: 2 in, 3 out]
                                }
                                }
                              }
                              frame #1 {
                                # "Wartezeit für\nneue Polarisatorposition"
                                n157 = local read "Wartezeit [s]"() -> (w206:dbl)
                                n158 = Multiply(x=w206, y=1000.0) -> (x*y=w205:dbl)
                                n159 = Wait (ms)(milliseconds to wait=w205) -> ()  [unwired: 1 out]
                              }
                              frame #2 {
                                n160 = local read "Aktuelle L/2-Position [°]"() -> (w210:dbl)
                                n161 = local read "Aktueller Messschritt"() -> (w215:i32)
                                n162 = local read "Start time [ms]"() -> (w217:timestamp)
                                n163 = local read "# Messschritte"() -> (w216:i32)
                                n164 = invoke class="MG17Motor" method="GetPosition"(reference=w213, "lChanID"=w212, "pfPosition"=w210) -> ("pfPosition"=w211:sgl)  [unwired: 2 in, 4 out]
                                n165 = call "estimate_stopp_time.vi"("Aktueller Messschritt"=w215, "# Messschritte"=w216, "Startzeit"=w217) -> ("Stopp Zeit"=w214:string)  [unwired: 8 in]
                                n166 = local write "Geschätzte Messzeit"(w214) -> ()
                                n167 = local write "Aktuelle L/2-Position [°]"(w211) -> ()
                              }
                            }
                          }
                        }
                      }
                      frame #1 {
                        (unwired) T7 {"Summierte Helligkeit (a.u.)"=0, "Aktuelle L/2-Position [°]"=0.0}
                      }
                    }
                  }
                }
              }
              frame #1 {
                n168 = flat-sequence {
                  frame #0 {
                    # "Zur Ausgangsposition zurückfahren"
                    n169 = local read "Wellenplatte [°]"() -> (w228:refnum<k7>)
                    n170 = local read "L/2-Start [°]"() -> (w222:dbl)
                    n171 = invoke class="MG17Motor" method="SetAbsMovePos"(reference=w228, "lChanID"=0, "fAbsPos"=w222) -> (reference out=w226:refnum<k7>, error out=w223:errorcluster, "lChanID"=w224:i32)  [unwired: 2 in, 2 out]
                    n172 = local read "Aktuelle L/2-Position [°]"() -> (w220:dbl)
                    n173 = invoke class="MG17Motor" method="MoveAbsolute"(reference=w226, error in=w223, "lChanID"=w224, "bWait"=TRUE) -> (reference out=w219:refnum<k7>, "lChanID"=w218:i32)  [unwired: 1 in, 3 out]
                    n174 = invoke class="MG17Motor" method="GetPosition"(reference=w219, "lChanID"=w218, "pfPosition"=w220) -> ("pfPosition"=w221:sgl)  [unwired: 2 in, 4 out]
                    n175 = local write "Aktuelle L/2-Position [°]"(w221) -> ()
                  }
                  frame #1 {
                    n176 = local read "Leistungs-/Polarisationscan läuft"() -> (w231:bool)
                    n177 = local read "Leistungs-/Polarisationscan läuft"() -> (w233:bool)
                    n178 = local read "Summierte Helligkeit speichern"() -> (w230:bool)
                    n179 = local read "Daten speichern"() -> (w234:bool)
                    n180 = And(x=w230, y=w231) -> (x .and. y?=w229:bool)
                    n181 = case shown="True" w229 {
                      frame #0 {
                      }
                      frame #1 {
                        n182 = local read "Save folder"() -> (w235:string)
                        n183 = local read "Vektor Summierte Helligkeit [a.u.]"() -> (w236:dbl[])
                        n184 = Concatenate Strings(w235, "\\" ("String"), "2D_Intensitaetsverteilung_MCP.dat" ("String")) -> (w240:string)
                        n185 = String To Path(string=w240) -> (path=w239:path)
                        n186 = call-poly <vilib>:"Write To Spreadsheet File.vi"("format (%.3f)"="%.;%8.0f", "1D data"=w236, "file path (dialog if empty)"=w239) -> ()  [unwired: 5 in, 1 out]
                      }
                    }
                    n187 = And(x=w234, y=w233) -> (x .and. y?=w232:bool)
                    n188 = case shown="True" w232 {
                      frame #0 {
                        n189 = local read "# L/2-Schritte"() -> (w244:i32)
                        n190 = local read "L/2-Schritt [°]"() -> (w243:dbl)
                        n191 = local read "L/2-Start [°]"() -> (w242:dbl)
                        n192 = local read "Save folder"() -> (w245:string)
                        n193 = call "create_axis_vector_file.vi"("Save folder"=w245, "Dateiname"="xAchse.dat", "Start"=w242, "Schrittlänge"=w243, "# Schritte"=w244) -> ()  [unwired: 11 in]
                      }
                      frame #1 {
                      }
                    }
                  }
                  frame #2 {
                    n194 = local read "# L/2-Schritte"() -> (w248:i32)
                    n195 = Decrement(x=w248) -> (x-1=w247:i32)
                    n196 = local write "# L/2-Schritte"(w247) -> ()
                  }
                  frame #3 {
                    n197 = local read "Detektionskamera"() -> (w250:T5)
                    n198 = local read "Buffer Interval"() -> (w251:u32)
                    n199 = call "camera_create_configuration.vi"("BufferInterval"=w251, "Session Out 2"=w250) -> ("Fehler (Ausgang)"=w252:errorcluster, "Ereignisregistrierung (Referenz)"=w249:refnum<event-registration>)  [unwired: 1 in, 1 out]
                    n200 = local write "Ereignis: FrameDone?"(w249) -> ()
                    n201 = local write "Fehler (Ausgang)"(w252) -> ()
                  }
                  frame #4 {
                    w253 = FALSE ("Spannungsscan läuft")
                    n202 = local write "Leistungs-/Polarisationsscan ON/OFF"(w253) -> ()
                    n203 = local write "Leistungs-/Polarisationscan läuft"(w253) -> ()
                  }
                }
              }
            }
          }
          frame #1 {
          }
        }
      }
      n204 = while "Kamera-Schleife" {
        i -> [w1624]
        stop <- w1625 stop-if-true
        n205 = local read "Fehler (Ausgang)"() -> (w1626:errorcluster)
        n206 = local read "Ereignis: FrameDone?"() -> (w1629:refnum<event-registration>)
        n207 = local read "Programm beenden"() -> (w1628:bool)
        n208 = Unbundle By Name(w1626) -> ("status"=w1627:bool)
        n209 = Or(x=w1627, y=w1628) -> (x .or. y?=w1625:bool)
        n210 = event "Kamera-Ereignisse" shown="[3] \"Helligkeit nullen\": Wertänderung" {
          selector: w1629 -> [_ _ _ _ _ _ _ _]
          dyn-events: _ -> [_ _ _ _ _ _ _ _]
          timeout: 1000 -> [_ _ _ _ _ _ _ _]
          event #0 {
            n211 = event-data() -> ()  [unwired: 1 in, 2 out]
          }
          event #1 {
            n212 = event-data() -> ()  [unwired: 1 in, 4 out]
            n213 = local read "Detektionskamera"() -> (w1632:T5)
            n214 = local read "Kamera ON/OFF"() -> (w1633:bool)
            n215 = case shown="True" w1633 {
              tunnel: w1632 -> [w1634 w1640]
              tunnel: [w1637 w1641] -> w1631
              frame #0 {
                n216 = local read "Image Memory"() -> (w1635:T4)
                n217 = call "camera_release configuration_stop.vi"("Image Memory"=w1635, "Detektionskamera"=w1634) -> ("error out"=w1637:errorcluster, "status"=w1636:bool)
                n218 = local write "Kamera"(w1636) -> ()
              }
              frame #1 {
                n219 = local read "Buffer Interval"() -> (w1639:u32)
                n220 = local read "Video Mode"() -> (w1638:u32)
                n221 = call "camera_acquisition_continously.vi"("Detektionskamera"=w1640, "BufferInterval"=w1639, "Video Mode"=w1638) -> ("Kamera eingeschaltet?"=w1645:bool, "Detektionskamera"=w1644:T5, "Image Memory"=w1643:T4, "Ereignis: FrameDone?"=w1642:refnum<event-registration>, "error out"=w1641:errorcluster)  [unwired: 1 in]
                n222 = local write "Image Memory"(w1643) -> ()
                n223 = local write "Detektionskamera"(w1644) -> ()
                n224 = local write "Ereignis: FrameDone?"(w1642) -> ()
                n225 = local write "Kamera"(w1645) -> ()
              }
            }
            n226 = local write "Fehler (Ausgang)"(w1631) -> ()
          }
          event #2 {
            w1660 = IMAQdx_Buffer_Number_Mode."Buffer Number"  # Buffer Number Mode
            n227 = event-data() -> ("ActualBufferNumber"=w1654:u32)  [unwired: 1 in]
            n228 = local read "Detektionskamera"() -> (w1659:T5)
            n229 = local read "Image Memory"() -> (w1658:T4)
            n230 = call <vilib>:"IMAQdx Get Image.vi"("Buffer Number Mode (Next)"=w1660, "Buffer Number In"=w1654, "Image In"=w1658, "Session In"=w1659) -> ("error out"=w1652:errorcluster, "Buffer Number Out"=w1655:u32, "Image Out"=w1651:T4, "Session Out"=w1656:T5)  [unwired: 1 in, 3 out]
            n231 = local write "Image Memory"(w1651) -> ()
            n232 = local write "Detektionskamera"(w1656) -> ()
            n233 = local write "Image Display"(w1651) -> ()
            n234 = local write "Buffer Number"(w1655) -> ()
            n235 = local write "Fehler (Ausgang)"(w1652) -> ()
            n236 = Not Equal?(x=w1655, y=w1654) -> (x != y?=w1653:bool)
            n237 = call "IMAQ ImageToArray"("Image"=w1651) -> ("Image Pixels (U8)"=w1648:u8[][])  [unwired: 3 in, 4 out]
            n238 = call "CalculateFPS.vi"("buffer number"=w1655) -> ("processed FPS"=w1657:dbl)  [unwired: 2 out]
            n239 = To Quad Integer(1:w1648) -> (0:w1647:i64[][])
            n240 = local write "Buffer Overrun"(w1653) -> ()
            n241 = local write "Frame Rate (FPS)"(w1657) -> ()
            n242 = Add Array Elements(numeric array=w1647) -> (sum=w1650:i64)
            n243 = local read "Hintergrund-Helligkeit"() -> (w1646:i64)
            n244 = Subtract(x=w1650, y=w1646) -> (x-y=w1649:i64)
            n245 = local write "Summierte Helligkeit (a.u.)"(w1649) -> ()
            n246 = local write "Helligkeitsverlauf"(w1649) -> ()
          }
          event #3 {
            n247 = event-data() -> ()  [unwired: 1 in, 2 out]
            n248 = case shown="True" "Helligkeit nullen" {
              frame #0 {
              }
              frame #1 {
                n249 = local read "Summierte Helligkeit (a.u.)"() -> (w1662:i64)
                n250 = local write "Hintergrund-Helligkeit"(w1662) -> ()
              }
            }
          }
          event #4 {
            n251 = event-data() -> ()  [unwired: 1 in, 2 out]
            n252 = local read "Kamera"() -> (w1663:bool)
            n253 = case shown="True" w1663 {
              frame #0 {
              }
              frame #1 {
                n254 = control-ref of="Shutter time (ms)"() -> (w1670:refnum<vi>)
                n255 = property class="Ring (strikt)"(reference=w1670) -> ("RingText.Text"=w1669:string)  [unwired: 1 in, 2 out]
                n256 = local read "Detektionskamera"() -> (w1668:T5)
                n257 = Decimal String To Number(string=w1669) -> (number=w1665:i32)  [unwired: 2 in, 1 out]
                n258 = property class="IMAQdx"(reference=w1668, "ActiveAttribute"="CameraAttributes::Shutter::Value", "ValueDBL"=w1665) -> (reference out=w1667:T5, error out=w1664:errorcluster)  [unwired: 1 in]
                n259 = local write "Detektionskamera"(w1667) -> ()
                n260 = local write "Fehler (Ausgang)"(w1664) -> ()
              }
            }
          }
          event #5 {
            n261 = event-data() -> ()  [unwired: 1 in, 1 out]
            n262 = local read "Kamera ON/OFF"() -> (w1671:bool)
            n263 = case shown="True" w1671 {
              frame #0 {
              }
              frame #1 {
                n264 = flat-sequence {
                  frame #0 {
                    n265 = local read "Detektionskamera"() -> (w1672:T5)
                    n266 = local read "Image Memory"() -> (w1673:T4)
                    n267 = call "camera_release configuration_stop.vi"("Image Memory"=w1673, "Detektionskamera"=w1672) -> ("status"=w1674:bool)  [unwired: 1 out]
                    n268 = local write "Kamera"(w1674) -> ()
                  }
                  frame #1 {
                    n269 = local read "Detektionskamera"() -> (w1675:T5)
                    n270 = control-ref of="Shutter time (ms)"() -> (w1678:refnum<vi>)
                    n271 = property class="Ring (strikt)"(reference=w1678) -> ("RingText.Text"=w1677:string)  [unwired: 1 in, 2 out]
                    n272 = local read "Buffer Interval"() -> (w1681:u32)
                    n273 = local read "Video Mode"() -> (w1680:u32)
                    n274 = Decimal String To Number(string=w1677) -> (number=w1676:i32)  [unwired: 2 in, 1 out]
                    n275 = call "camera_acquisition_continously.vi"("Detektionskamera"=w1675, "BufferInterval"=w1681, "Video Mode"=w1680, "Shutter time (ms)"=w1676) -> ("Kamera eingeschaltet?"=w1685:bool, "Detektionskamera"=w1684:T5, "Image Memory"=w1683:T4, "Ereignis: FrameDone?"=w1682:refnum<event-registration>, "error out"=w1679:errorcluster)
                    n276 = local write "Image Memory"(w1683) -> ()
                    n277 = local write "Detektionskamera"(w1684) -> ()
                    n278 = local write "Ereignis: FrameDone?"(w1682) -> ()
                    n279 = local write "Fehler (Ausgang)"(w1679) -> ()
                    n280 = local write "Kamera"(w1685) -> ()
                  }
                }
              }
            }
          }
          event #6 {
            n281 = event-data() -> ()  [unwired: 1 in, 1 out]
            n282 = local read "Kamera"() -> (w1686:bool)
            n283 = case shown="True" w1686 {
              frame #0 {
              }
              frame #1 {
                n284 = local read "Ereignis: FrameDone?"() -> (w1688:refnum<event-registration>)
                n285 = local read "Detektionskamera"() -> (w1692:T5)
                n286 = local read "Buffer Interval"() -> (w1691:u32)
                n287 = local read "ROI"() -> (w1693:i32[])
                n288 = call "camera_change_ROI.vi"("BufferInterval"=w1691, "Region of Interest"=w1693, "Ereignisregistrierung (Referenz) 2"=w1688, "Session In"=w1692) -> ("Fehler (Ausgang)"=w1687:errorcluster, "Ereignisregistrierung (Referenz)"=w1690:refnum<event-registration>, "Session Out"=w1689:T5)  [unwired: 5 in]
                n289 = local write "Detektionskamera"(w1689) -> ()
                n290 = local write "Ereignis: FrameDone?"(w1690) -> ()
                n291 = local write "Fehler (Ausgang)"(w1687) -> ()
              }
            }
          }
          event #7 {
            n292 = event-data() -> ("NewVal"=w1695:bool)  [unwired: 1 in, 1 out]
            n293 = local read "Kamera"() -> (w1696:bool)
            n294 = And(x=w1696, y=w1695) -> (x .and. y?=w1694:bool)
            n295 = case shown="True" w1694 {
              frame #0 {
              }
              frame #1 {
                w1697 = i32[] [640, 480, 0, 0] ("Region of Interest (px)")
                n296 = local read "Ereignis: FrameDone?"() -> (w1699:refnum<event-registration>)
                n297 = local read "Detektionskamera"() -> (w1703:T5)
                n298 = local read "Buffer Interval"() -> (w1702:u32)
                n299 = call "camera_change_ROI.vi"("BufferInterval"=w1702, "Region of Interest"=w1697, "Ereignisregistrierung (Referenz) 2"=w1699, "Session In"=w1703) -> ("Fehler (Ausgang)"=w1698:errorcluster, "Ereignisregistrierung (Referenz)"=w1701:refnum<event-registration>, "Session Out"=w1700:T5)  [unwired: 5 in]
                n300 = local write "ROI"(w1697) -> ()
                n301 = local write "Detektionskamera"(w1700) -> ()
                n302 = local write "Ereignis: FrameDone?"(w1701) -> ()
                n303 = local write "Fehler (Ausgang)"(w1698) -> ()
              }
            }
          }
        }
        "Kameraschleifenzähler" <- w1624
      }
      n304 = while "Steuerungs-Schleife" {
        i -> [w614]
        stop <- w613 stop-if-true
        n305 = event shown="[0] \"HV ON/OFF\": Wertänderung" {
          selector: _ -> [_ _ _ _ _]
          dyn-events: _ -> [_ _ _ _ _]
          timeout: 1000 -> [_ _ _ _ _]
          event #0 {
            w619 = 0.0 ("Suppressor-Spannung [V]")
            n306 = event-data() -> ("NewVal"=w620:bool)  [unwired: 1 in]
            n307 = local write "HV-Steuerung"(w620) -> ()
            n308 = local write "Suppressor-Spannung [V]"(w619) -> ()
            n309 = local write "Tip-Spannung [V]"(w619) -> ()
            n310 = call "HV_power_supply_set_voltage.vi"("Desired output voltage in V (HV power supply)"=0.0, "Channel of HV power supply"=refnum<k21> "Dev0/Ao0") -> ("error out"=w622:errorcluster)  [unwired: 8 in]
            n311 = call "HV_power_supply_set_voltage.vi"("error in"=w622, "Desired output voltage in V (HV power supply)"=0.0, "Channel of HV power supply"=refnum<k21> "Dev0/Ao1") -> ("error out"=w621:errorcluster)  [unwired: 7 in]
            n312 = local write "Fehler (Ausgang)"(w621) -> ()
          }
          event #1 {
            n313 = event-data() -> ("NewVal"=w627:bool)  [unwired: 1 in]
            n314 = case shown="True" w627 {
              frame #0 {
                n315 = local read "Wellenplatte [°]"() -> (w630:refnum<k7>)
                n316 = invoke class="MG17Motor" method="StopCtrl"(reference=w630) -> (error out=w629:errorcluster)  [unwired: 2 in, 2 out]
                n317 = Unbundle By Name(w629) -> ("status"=w628:bool)
                n318 = local write "Wellenplatte"(w628) -> ()
              }
              frame #1 {
                n319 = property class="MG17Motor"(reference="Wellenplatte [°]", "HWSerialNum"="SN von Rotationsbühne") -> (reference out=w637:refnum<k7>, error out=w636:errorcluster)  [unwired: 1 in]
                n320 = invoke class="MG17Motor" method="StartCtrl"(reference=w637, error in=w636) -> (error out=w635:errorcluster)  [unwired: 1 in, 2 out]
                n321 = local write "Fehler (Ausgang)"(w635) -> ()
                n322 = Unbundle By Name(w635) -> ("status"=w634:bool)
                n323 = Not(x=w634) -> (.not. x?=w633:bool)
                n324 = local write "Wellenplatte"(w633) -> ()
              }
            }
          }
          event #2 {
            n325 = event-data() -> ("OldVal"=w638:dbl, "NewVal"=w644:dbl)  [unwired: 1 in]
            n326 = local read "Suppressor-Spannung [V]"() -> (w643:dbl)
            n327 = local read "Max. Spannungsdifferenz"() -> (w641:dbl)
            n328 = local read "HV-Steuerung"() -> (w639:bool)
            n329 = Subtract(x=w644, y=w643) -> (x-y=w642:dbl)
            n330 = Less Or Equal?(x=w642, y=w641) -> (x <= y?=w640:bool)
            n331 = case shown="True" w639 {
              tunnel: w640 -> [_ w646]
              tunnel: w638 -> [_ w645]
              frame #0 {
              }
              frame #1 {
                n332 = case shown="True" w646 {
                  tunnel: w645 -> [w647 _]
                  frame #0 {
                    n333 = local write "Tip-Spannung [V]"(w647) -> ()
                  }
                  frame #1 {
                    n334 = local read "Tip-Spannung [V]"() -> (w648:dbl)
                    n335 = call "HV_power_supply_set_voltage.vi"("Desired output voltage in V (HV power supply)"=w648, "Channel of HV power supply"=refnum<k21> "Dev0/Ao1") -> ("error out"=w649:errorcluster)  [unwired: 8 in]
                    n336 = local write "Fehler (Ausgang)"(w649) -> ()
                  }
                }
              }
            }
          }
          event #3 {
            n337 = event-data() -> ("OldVal"=w651:dbl, "NewVal"=w653:dbl)  [unwired: 1 in]
            n338 = local read "Tip-Spannung [V]"() -> (w652:dbl)
            n339 = local read "Max. Spannungsdifferenz"() -> (w654:dbl)
            n340 = Subtract(x=w652, y=w653) -> (x-y=w656:dbl)
            n341 = local read "HV-Steuerung"() -> (w657:bool)
            n342 = Less Or Equal?(x=w656, y=w654) -> (x <= y?=w655:bool)
            n343 = case shown="True" w657 {
              tunnel: w655 -> [_ w659]
              tunnel: w651 -> [_ w658]
              frame #0 {
              }
              frame #1 {
                n344 = case shown="True" w659 {
                  tunnel: w658 -> [w660 _]
                  frame #0 {
                    n345 = local write "Suppressor-Spannung [V]"(w660) -> ()
                  }
                  frame #1 {
                    n346 = local read "Suppressor-Spannung [V]"() -> (w661:dbl)
                    n347 = call "HV_power_supply_set_voltage.vi"("Desired output voltage in V (HV power supply)"=w661, "Channel of HV power supply"=refnum<k21> "Dev0/Ao0") -> ("error out"=w662:errorcluster)  [unwired: 8 in]
                    n348 = local write "Fehler (Ausgang)"(w662) -> ()
                  }
                }
              }
            }
          }
          event #4 {
            n349 = event-data() -> ()  [unwired: 1 in, 2 out]
          }
        }
        n350 = local read "Fehler (Ausgang)"() -> (w618:errorcluster)
        n351 = local read "Programm beenden"() -> (w617:bool)
        n352 = Unbundle By Name(w618) -> ("status"=w616:bool)
        n353 = Or(x=w616, y=w617) -> (x .or. y?=w613:bool)
        "Steuerschleifenzähler" <- w614
      }
      n354 = while "Spannungsscan-Schleife" {
        stop <- w435 stop-if-true
        n355 = local read "Fehler (Ausgang)"() -> (w436:errorcluster)
        n356 = local read "Spannungsscan läuft"() -> (w434:bool)
        n357 = local read "Programm beenden"() -> (w438:bool)
        n358 = Unbundle By Name(w436) -> ("status"=w437:bool)
        n359 = Or(x=w437, y=w438) -> (x .or. y?=w435:bool)
        n360 = case shown="True" w434 {
          frame #0 {
          }
          frame #1 {
            n361 = stacked-sequence {
              frame #0 {
                n362 = local read "# Spannungsschritte"() -> (w443:i32[])
                n363 = Index Array(array=w443, index #1=0 ("Index"), index #2=1 ("Index")) -> (element #1=w440:i32, element #2=w439:i32)
                n364 = for "Schleife für Tip-Spannung" {
                  N: w440 -> [_]
                  tunnel: w439 -> [w444]
                  i -> [w445]
                  n365 = local read "Spannungsscan läuft"() -> (w446:bool)
                  n366 = case shown="True" w446 {
                    tunnel: w445 -> [_ w448]
                    tunnel: w444 -> [_ w447]
                    frame #0 {
                    }
                    frame #1 {
                      n367 = stacked-sequence {
                        tunnel: w448 -> [w450 _]
                        tunnel: w447 -> [w449 _]
                        frame #0 {
                          n368 = for "Schleife für Suppressor-Spannung" {
                            N: w449 -> [_]
                            tunnel: w450 -> [w452]
                            i -> [w451]
                            n369 = local read "Spannungsscan läuft"() -> (w453:bool)
                            n370 = case shown="True" w453 {
                              tunnel: w452 -> [_ w455]
                              tunnel: w451 -> [_ w454]
                              frame #0 {
                              }
                              frame #1 {
                                n371 = stacked-sequence {
                                tunnel: w455 -> [_ _ w499 _]
                                tunnel: w454 -> [_ _ w498 _]
                                frame #0 {
                                n372 = local write "Summierte Helligkeit (a.u.)"(u64 0 ("Summierte Helligkeit (a.u.)")) -> ()
                                n373 = local read "ROI"() -> (w461:i32[])
                                n374 = local read "Aktueller Messschritt"() -> (w458:i32)
                                n375 = Index Array(array=w461, index #1=0 ("Index"), index #2=1 ("Index")) -> (element #1=w465:i32, element #2=w464:i32)
                                n376 = Initialize Array(u64 0 ("Element"), w464, w465) -> (w459:u64[][])
                                n377 = local write "Gemitteltes Bild"(w459) -> ()
                                n378 = Increment(x=w458) -> (x+1=w457:i32)
                                n379 = local write "Aktueller Messschritt"(w457) -> ()
                                }
                                frame #1 {
                                n380 = local read "# Bilder/Messschritt"() -> (w469:i32)
                                n381 = local read "Detektionskamera"() -> (w472:T5)
                                n382 = local read "Einzelbilder speichern"() -> (w467:bool)
                                n383 = call "camera_acquisition_sequence.vi"("Session In"=w472, "Desired image number"=w469) -> ("Image Array"=w466:T4[], "error out"=w471:errorcluster)  [unwired: 2 in, 1 out]
                                n384 = case shown="True" w467 {
                                tunnel: w471 -> [w474 w482]
                                tunnel: [w474 w481] -> w470
                                tunnel: w469 -> [w473 w480]
                                tunnel: [w473 w480] -> w468
                                tunnel: w466 -> [_ w479]
                                frame #0 {
                                }
                                frame #1 {
                                n385 = local read "Aktueller Messschritt"() -> (w485:i32)
                                n386 = local read "Save folder"() -> (w477:string)
                                n387 = Concatenate Strings(w477, "Einzelbilder\\" ("String")) -> (w475:string)
                                n388 = Format Into String(format string="%05.0f" ("Format-String"), initial string="#" ("Eingangs-String"), w485) -> (resulting string=w478:string)  [unwired: 1 in, 1 out]
                                n389 = call "save images.vi"("Save Folder"=w475, "File name prefix"=w478, "Array"=w479, "error out 2"=w482, "Bilder/Messschritt"=w480) -> ("error out"=w481:errorcluster)
                                }
                                }
                                n390 = for {
                                N: w468 -> [_]
                                tunnel: w470 -> [w494]
                                tunnel: w466 -> [w492] mode=indexing
                                n391 = call "IMAQ ImageToArray"("error in (no error)"=w494, "Image"=w492) -> ("error out"=w493:errorcluster, "Image Pixels (U8)"=w491:u8[][])  [unwired: 2 in, 3 out]
                                n392 = local read "Gemitteltes Bild"() -> (w489:u64[][])
                                n393 = local write "Fehler (Ausgang)"(w493) -> ()
                                n394 = To Quad Integer(1:w491) -> (0:w495:i64[][])
                                n395 = Add Array Elements(numeric array=w495) -> (sum=w488:i64)
                                n396 = local read "Summierte Helligkeit (a.u.)"() -> (w496:i64)
                                n397 = Add(x=w489, y=w491) -> (x+y=w490:u64[][])
                                n398 = local write "Gemitteltes Bild"(w490) -> ()
                                n399 = local read "Hintergrund-Helligkeit"() -> (w486:i64)
                                n400 = Subtract(x=w488, y=w486) -> (x-y=w487:i64)
                                n401 = Add(x=w487, y=w496) -> (x+y=w497:i64)
                                n402 = local write "Summierte Helligkeit (a.u.)"(w497) -> ()
                                }
                                }
                                frame #2 {
                                n403 = local read "# Bilder/Messschritt"() -> (w505:i32)
                                n404 = local read "2D-Intensitätsverteilung (MCP)"() -> (w502:dbl[][])
                                n405 = local read "Gemitteltes Bild"() -> (w503:u64[][])
                                n406 = local read "Summierte Helligkeit (a.u.)"() -> (w500:i64)
                                n407 = local read "Gemittelte Bilder speichern"() -> (w509:bool)
                                n408 = local read "Image Display"() -> (w507:T4)
                                n409 = Divide(x=w503, y=w505) -> (x/y=w504:dbl[][])
                                n410 = Replace Array Subset(array=w502, new element=w500, index (row)=w499, index (col)=w498) -> (w501:dbl[][])
                                n411 = call "IMAQ ArrayToImage"("Image Pixels (U8)"=w504, "Image"=w507) -> ("Image Out"=w506:T4)  [unwired: 8 in, 1 out]
                                n412 = local write "2D-Intensitätsverteilung (MCP)"(w501) -> ()
                                n413 = case shown="True" w509 {
                                tunnel: w506 -> [w510 w521]
                                tunnel: [w510 w512] -> w508
                                frame #0 {
                                }
                                frame #1 {
                                n414 = local read "Aktueller Messschritt"() -> (w516:i32)
                                n415 = local read "Save folder"() -> (w518:string)
                                n416 = Format Into String(format string="%05.0f" ("Format-String"), initial string="#" ("Eingangs-String"), w516) -> (resulting string=w515:string)  [unwired: 1 in, 1 out]
                                n417 = Concatenate Strings(w518, "Gemittelte Bilder\\" ("String"), w515, ".png" ("String")) -> (w514:string)
                                n418 = String To Path(string=w514) -> (path=w513:path)
                                n419 = call-poly "IMAQ Write File 2"("File Path"=w513, "Image"=w521) -> ("Image Out (duplicate)"=w512:T4)  [unwired: 8 in, 1 out]
                                }
                                }
                                n420 = local write "Image Display"(w508) -> ()
                                }
                                frame #3 {
                                n421 = flat-sequence {
                                frame #0 {
                                n422 = local read "Aktuelle Spannung [V]"() -> (w524:dbl[])
                                n423 = local read "Spannungsschritt [V]"() -> (w528:dbl[])
                                n424 = Index Array(array=w524, index=1 ("Index")) -> (element=w526:dbl)
                                n425 = Index Array(array=w528, index=1 ("Index")) -> (element=w527:dbl)
                                n426 = Add(x=w526, y=w527) -> (x+y=w522:dbl)
                                n427 = local write "Suppressor-Spannung [V]"(w522) -> ()
                                n428 = call "HV_power_supply_set_voltage.vi"("Desired output voltage in V (HV power supply)"=w522, "Channel of HV power supply"=refnum<k21> "Dev0/Ao0") -> ("error out"=w531:errorcluster)  [unwired: 8 in]
                                n429 = local write "Fehler (Ausgang)"(w531) -> ()
                                n430 = Replace Array Subset(array=w524, new element=w522, index=1 ("Index")) -> (w523:dbl[])
                                n431 = local write "Aktuelle Spannung [V]"(w523) -> ()
                                }
                                frame #1 {
                                # "Wartezeit für\nneue Spannung"
                                n432 = Wait (ms)(milliseconds to wait=u32 200 ("Zu wartende ms")) -> ()  [unwired: 1 out]
                                }
                                frame #2 {
                                n433 = local read "Aktueller Messschritt"() -> (w535:i32)
                                n434 = local read "Start time [ms]"() -> (w537:timestamp)
                                n435 = local read "# Messschritte"() -> (w536:i32)
                                n436 = call "estimate_stopp_time.vi"("Aktueller Messschritt"=w535, "# Messschritte"=w536, "Startzeit"=w537) -> ("Stopp Zeit"=w534:string)  [unwired: 8 in]
                                n437 = local write "Geschätzte Messzeit"(w534) -> ()
                                }
                                }
                                }
                                }
                              }
                            }
                          }
                        }
                        frame #1 {
                          n438 = flat-sequence {
                            frame #0 {
                              n439 = local read "Spannungsstart [V]"() -> (w543:dbl[])
                              n440 = local read "Aktuelle Spannung [V]"() -> (w545:dbl[])
                              n441 = Index Array(array=w543, index=1 ("Index")) -> (element=w538:dbl)
                              n442 = local write "Suppressor-Spannung [V]"(w538) -> ()
                              n443 = call "HV_power_supply_set_voltage.vi"("Desired output voltage in V (HV power supply)"=w538, "Channel of HV power supply"=refnum<k21> "Dev0/Ao0") -> ("error out"=w539:errorcluster)  [unwired: 8 in]
                              n444 = local write "Fehler (Ausgang)"(w539) -> ()
                              n445 = Replace Array Subset(array=w545, new element=w538, index=1 ("Index")) -> (w541:dbl[])
                              n446 = local write "Aktuelle Spannung [V]"(w541) -> ()
                            }
                            frame #1 {
                              n447 = local read "Aktuelle Spannung [V]"() -> (w548:dbl[])
                              n448 = local read "Spannungsschritt [V]"() -> (w552:dbl[])
                              n449 = Index Array(array=w548, index=0 ("Index")) -> (element=w550:dbl)
                              n450 = Index Array(array=w552, index=0 ("Index")) -> (element=w551:dbl)
                              n451 = Add(x=w550, y=w551) -> (x+y=w546:dbl)
                              n452 = local write "Tip-Spannung [V]"(w546) -> ()
                              n453 = call "HV_power_supply_set_voltage.vi"("Desired output voltage in V (HV power supply)"=w546, "Channel of HV power supply"=refnum<k21> "Dev0/Ao1") -> ("error out"=w555:errorcluster)  [unwired: 8 in]
                              n454 = local write "Fehler (Ausgang)"(w555) -> ()
                              n455 = Replace Array Subset(array=w548, new element=w546, index=0 ("Index")) -> (w547:dbl[])
                              n456 = local write "Aktuelle Spannung [V]"(w547) -> ()
                            }
                            frame #2 {
                              # "Wartezeit für\nStartspannung"
                              n457 = Wait (ms)(milliseconds to wait=u32 6000 ("Zu wartende ms")) -> ()  [unwired: 1 out]
                            }
                          }
                        }
                      }
                    }
                  }
                }
              }
              frame #1 {
                n458 = local read "Spannungsscan läuft"() -> (w558:bool)
                n459 = case shown="False" w558 {
                  frame #0 {
                    n460 = flat-sequence {
                      frame #0 {
                        # "Zur Ausgangsposition zurückfahren"
                        n461 = local read "Spannungsstart [V]"() -> (w564:dbl[])
                        n462 = local read "Spannungsstart [V]"() -> (w559:dbl[])
                        n463 = local read "Detektionskamera"() -> (w571:T5)
                        n464 = local read "Buffer Interval"() -> (w570:u32)
                        n465 = local write "Aktuelle Spannung [V]"(w559) -> ()
                        n466 = call "camera_create_configuration.vi"("BufferInterval"=w570, "Session Out 2"=w571) -> ("Fehler (Ausgang)"=w565:errorcluster, "Ereignisregistrierung (Referenz)"=w572:refnum<event-registration>)  [unwired: 1 in, 1 out]
                        n467 = Index Array(array=w564, index #1=0 ("Index"), index #2=1 ("Index")) -> (element #1=w560:dbl, element #2=w561:dbl)
                        n468 = local write "Tip-Spannung [V]"(w560) -> ()
                        n469 = local write "Suppressor-Spannung [V]"(w561) -> ()
                        n470 = local write "Ereignis: FrameDone?"(w572) -> ()
                        n471 = call "HV_power_supply_set_voltage.vi"("error in"=w565, "Desired output voltage in V (HV power supply)"=w561, "Channel of HV power supply"=refnum<k21> "Dev0/Ao0") -> ("error out"=w567:errorcluster)  [unwired: 7 in]
                        n472 = call "HV_power_supply_set_voltage.vi"("error in"=w567, "Desired output voltage in V (HV power supply)"=w560, "Channel of HV power supply"=refnum<k21> "Dev0/Ao1") -> ("error out"=w566:errorcluster)  [unwired: 7 in]
                        n473 = local write "Fehler (Ausgang)"(w566) -> ()
                      }
                    }
                  }
                  frame #1 {
                    n474 = flat-sequence {
                      frame #0 {
                        n475 = local read "2D-Intensitätsverteilung (MCP)"() -> (w573:dbl[][])
                        n476 = control-ref of="2D-Intensitätsverteilung (MCP)"() -> (w576:refnum<vi>)
                        n477 = Array Max & Min(array=w573) -> (max value=w574:dbl, min value=w575:dbl)  [unwired: 2 out]
                        n478 = property class="IntGraph (strikt)"(reference=w576, "ZScale.Maximum"=w574, "ZScale.Minimum"=w575) -> ()  [unwired: 1 in, 2 out]
                      }
                      frame #1 {
                        # "Zur Ausgangsposition zurückfahren"
                        n479 = local read "Spannungsstart [V]"() -> (w577:dbl[])
                        n480 = local read "Spannungsstart [V]"() -> (w582:dbl[])
                        n481 = local read "Detektionskamera"() -> (w589:T5)
                        n482 = local read "Buffer Interval"() -> (w588:u32)
                        n483 = local write "Aktuelle Spannung [V]"(w577) -> ()
                        n484 = call "camera_create_configuration.vi"("BufferInterval"=w588, "Session Out 2"=w589) -> ("Fehler (Ausgang)"=w583:errorcluster, "Ereignisregistrierung (Referenz)"=w590:refnum<event-registration>)  [unwired: 1 in, 1 out]
                        n485 = Index Array(array=w582, index #1=0 ("Index"), index #2=1 ("Index")) -> (element #1=w578:dbl, element #2=w579:dbl)
                        n486 = local write "Tip-Spannung [V]"(w578) -> ()
                        n487 = local write "Suppressor-Spannung [V]"(w579) -> ()
                        n488 = local write "Ereignis: FrameDone?"(w590) -> ()
                        n489 = call "HV_power_supply_set_voltage.vi"("error in"=w583, "Desired output voltage in V (HV power supply)"=w579, "Channel of HV power supply"=refnum<k21> "Dev0/Ao0") -> ("error out"=w585:errorcluster)  [unwired: 7 in]
                        n490 = call "HV_power_supply_set_voltage.vi"("error in"=w585, "Desired output voltage in V (HV power supply)"=w578, "Channel of HV power supply"=refnum<k21> "Dev0/Ao1") -> ("error out"=w584:errorcluster)  [unwired: 7 in]
                        n491 = local write "Fehler (Ausgang)"(w584) -> ()
                      }
                      frame #2 {
                        n492 = local read "Daten speichern"() -> (w591:bool)
                        n493 = case shown="True" w591 {
                          frame #0 {
                          }
                          frame #1 {
                            w592 = 1 ("Index")
                            w604 = 0 ("Index")
                            n494 = local read "Spannungsschritt [V]"() -> (w602:dbl[])
                            n495 = local read "# Spannungsschritte"() -> (w603:i32[])
                            n496 = local read "Spannungsstart [V]"() -> (w601:dbl[])
                            n497 = local read "Save folder"() -> (w593:string)
                            n498 = Index Array(array=w601, index #1=w604, index #2=w592) -> (element #1=w600:dbl, element #2=w596:dbl)
                            n499 = Index Array(array=w602, index #1=w604, index #2=w592) -> (element #1=w599:dbl, element #2=w595:dbl)
                            n500 = Index Array(array=w603, index #1=w604, index #2=w592) -> (element #1=w598:i32, element #2=w594:i32)
                            n501 = local read "2D-Intensitätsverteilung (MCP)"() -> (w610:dbl[][])
                            n502 = call "create_axis_vector_file.vi"("Save folder"=w593, "Dateiname"="xAchse.dat" ("Save folder"), "Start"=w600, "Schrittlänge"=w599, "# Schritte"=w598) -> ()  [unwired: 11 in]
                            n503 = call "create_axis_vector_file.vi"("Save folder"=w593, "Dateiname"="yAchse.dat", "Start"=w596, "Schrittlänge"=w595, "# Schritte"=w594) -> ()  [unwired: 11 in]
                            n504 = Concatenate Strings(w593, "\\" ("String"), "2D_Intensitaetsverteilung_MCP.dat" ("String")) -> (w607:string)
                            n505 = String To Path(string=w607) -> (path=w608:path)
                            n506 = call-poly <vilib>:"Write To Spreadsheet File.vi"("format (%.3f)"="%.;%8.0f", "2D data"=w610, "file path (dialog if empty)"=w608) -> ()  [unwired: 5 in, 1 out]
                          }
                        }
                      }
                      frame #3 {
                        w612 = FALSE ("Spannungsscan läuft")
                        n507 = local write "Spannungsscan ON/OFF"(w612) -> ()
                        n508 = local write "Spannungsscan läuft"(w612) -> ()
                      }
                    }
                  }
                }
              }
            }
          }
        }
      }
      n509 = while "x-U-Scan Schleife" {
        stop <- w255 stop-if-true
        n510 = local read "Fehler (Ausgang)"() -> (w256:errorcluster)
        n511 = local read "x-U-Scan läuft"() -> (w254:bool)
        n512 = local read "Programm beenden"() -> (w258:bool)
        n513 = case shown="True" w254 {
          frame #0 {
          }
          frame #1 {
            n514 = stacked-sequence {
              frame #0 {
                n515 = local read "# x-U-Scan x-Rasterschritte"() -> (w259:i32)
                n516 = for "Schleife für Raumkoordinate" {
                  N: w259 -> [_]
                  i -> [w260]
                  n517 = local read "x-U-Scan läuft"() -> (w261:bool)
                  n518 = case shown="True" w261 {
                    tunnel: w260 -> [_ w262]
                    frame #0 {
                    }
                    frame #1 {
                      n519 = stacked-sequence {
                        tunnel: w262 -> [w264 _]
                        frame #0 {
                          n520 = local read "# x-U-Scan Spannungsschritte"() -> (w263:i32)
                          n521 = for "Schleife für Spannungskoordinate" {
                            N: w263 -> [_]
                            tunnel: w264 -> [w266]
                            i -> [w265]
                            n522 = local read "x-U-Scan läuft"() -> (w267:bool)
                            n523 = case shown="True" w267 {
                              tunnel: w266 -> [_ w269]
                              tunnel: w265 -> [_ w268]
                              frame #0 {
                              }
                              frame #1 {
                                n524 = stacked-sequence {
                                tunnel: w269 -> [_ _ w313 _]
                                tunnel: w268 -> [_ _ w312 _]
                                frame #0 {
                                n525 = local write "Summierte Helligkeit (a.u.)"(u64 0 ("Summierte Helligkeit (a.u.)")) -> ()
                                n526 = local read "ROI"() -> (w275:i32[])
                                n527 = local read "Aktueller Messschritt"() -> (w272:i32)
                                n528 = Index Array(array=w275, index #1=0 ("Index"), index #2=1 ("Index")) -> (element #1=w279:i32, element #2=w278:i32)
                                n529 = Initialize Array(u64 0 ("Element"), w278, w279) -> (w273:u64[][])
                                n530 = local write "Gemitteltes Bild"(w273) -> ()
                                n531 = Increment(x=w272) -> (x+1=w271:i32)
                                n532 = local write "Aktueller Messschritt"(w271) -> ()
                                }
                                frame #1 {
                                n533 = local read "# Bilder/Messschritt"() -> (w283:i32)
                                n534 = local read "Detektionskamera"() -> (w286:T5)
                                n535 = local read "Einzelbilder speichern"() -> (w281:bool)
                                n536 = call "camera_acquisition_sequence.vi"("Session In"=w286, "Desired image number"=w283) -> ("Image Array"=w280:T4[], "error out"=w285:errorcluster)  [unwired: 2 in, 1 out]
                                n537 = case shown="True" w281 {
                                tunnel: w285 -> [w288 w296]
                                tunnel: [w288 w295] -> w284
                                tunnel: w283 -> [w287 w294]
                                tunnel: [w287 w294] -> w282
                                tunnel: w280 -> [_ w293]
                                frame #0 {
                                }
                                frame #1 {
                                n538 = local read "Aktueller Messschritt"() -> (w299:i32)
                                n539 = local read "Save folder"() -> (w291:string)
                                n540 = Concatenate Strings(w291, "Einzelbilder\\" ("String")) -> (w289:string)
                                n541 = Format Into String(format string="%05.0f" ("Format-String"), initial string="#" ("Eingangs-String"), w299) -> (resulting string=w292:string)  [unwired: 1 in, 1 out]
                                n542 = call "save images.vi"("Save Folder"=w289, "File name prefix"=w292, "Array"=w293, "error out 2"=w296, "Bilder/Messschritt"=w294) -> ("error out"=w295:errorcluster)
                                }
                                }
                                n543 = for {
                                N: w282 -> [_]
                                tunnel: w284 -> [w308]
                                tunnel: w280 -> [w306] mode=indexing
                                n544 = call "IMAQ ImageToArray"("error in (no error)"=w308, "Image"=w306) -> ("error out"=w307:errorcluster, "Image Pixels (U8)"=w305:u8[][])  [unwired: 2 in, 3 out]
                                n545 = local read "Gemitteltes Bild"() -> (w303:u64[][])
                                n546 = local read "Summierte Helligkeit (a.u.)"() -> (w310:i64)
                                n547 = local write "Fehler (Ausgang)"(w307) -> ()
                                n548 = To Quad Integer(1:w305) -> (0:w309:i64[][])
                                n549 = Add Array Elements(numeric array=w309) -> (sum=w302:i64)
                                n550 = Add(x=w303, y=w305) -> (x+y=w304:u64[][])
                                n551 = local write "Gemitteltes Bild"(w304) -> ()
                                n552 = local read "Hintergrund-Helligkeit"() -> (w300:i64)
                                n553 = Subtract(x=w302, y=w300) -> (x-y=w301:i64)
                                n554 = Add(x=w301, y=w310) -> (x+y=w311:i64)
                                n555 = local write "Summierte Helligkeit (a.u.)"(w311) -> ()
                                }
                                }
                                frame #2 {
                                n556 = local read "# Bilder/Messschritt"() -> (w319:i32)
                                n557 = local read "2D-Intensitätsverteilung (MCP)"() -> (w316:dbl[][])
                                n558 = local read "Gemitteltes Bild"() -> (w317:u64[][])
                                n559 = local read "Summierte Helligkeit (a.u.)"() -> (w314:i64)
                                n560 = local read "Gemittelte Bilder speichern"() -> (w323:bool)
                                n561 = local read "Image Display"() -> (w321:T4)
                                n562 = Divide(x=w317, y=w319) -> (x/y=w318:dbl[][])
                                n563 = call "IMAQ ArrayToImage"("Image Pixels (U8)"=w318, "Image"=w321) -> ("Image Out"=w320:T4)  [unwired: 8 in, 1 out]
                                n564 = Replace Array Subset(array=w316, new element=w314, index (row)=w313, index (col)=w312) -> (w315:dbl[][])
                                n565 = local write "2D-Intensitätsverteilung (MCP)"(w315) -> ()
                                n566 = case shown="True" w323 {
                                tunnel: w320 -> [w324 w335]
                                tunnel: [w324 w326] -> w322
                                frame #0 {
                                }
                                frame #1 {
                                n567 = local read "Aktueller Messschritt"() -> (w330:i32)
                                n568 = local read "Save folder"() -> (w332:string)
                                n569 = Format Into String(format string="%05.0f" ("Format-String"), initial string="#" ("Eingangs-String"), w330) -> (resulting string=w329:string)  [unwired: 1 in, 1 out]
                                n570 = Concatenate Strings(w332, "Gemittelte Bilder\\" ("String"), w329, ".png" ("String")) -> (w328:string)
                                n571 = String To Path(string=w328) -> (path=w327:path)
                                n572 = call-poly "IMAQ Write File 2"("File Path"=w327, "Image"=w335) -> ("Image Out (duplicate)"=w326:T4)  [unwired: 8 in, 1 out]
                                }
                                }
                                n573 = local write "Image Display"(w322) -> ()
                                }
                                frame #3 {
                                n574 = flat-sequence {
                                frame #0 {
                                n575 = local read "x-U-Scan aktuelle Spannung [V]"() -> (w338:dbl)
                                n576 = local read "x-U-Scan Spannungsschritt [V]"() -> (w339:dbl)
                                n577 = local read "Spannungskanal"() -> (w337:refnum<k21>)
                                n578 = Add(x=w338, y=w339) -> (x+y=w336:dbl)
                                n579 = local write "x-U-Scan aktuelle Spannung [V]"(w336) -> ()
                                n580 = call "HV_power_supply_set_voltage.vi"("Desired output voltage in V (HV power supply)"=w336, "Channel of HV power supply"=w337) -> ("error out"=w340:errorcluster)  [unwired: 8 in]
                                n581 = local write "Fehler (Ausgang)"(w340) -> ()
                                }
                                frame #1 {
                                # "Wartezeit für\nneue Spannung"
                                n582 = Wait (ms)(milliseconds to wait=u32 200 ("Zu wartende ms")) -> ()  [unwired: 1 out]
                                }
                                frame #2 {
                                n583 = local read "Aktueller Messschritt"() -> (w343:i32)
                                n584 = local read "Start time [ms]"() -> (w345:timestamp)
                                n585 = local read "# Messschritte"() -> (w344:i32)
                                n586 = call "estimate_stopp_time.vi"("Aktueller Messschritt"=w343, "# Messschritte"=w344, "Startzeit"=w345) -> ("Stopp Zeit"=w342:string)  [unwired: 8 in]
                                n587 = local write "Geschätzte Messzeit"(w342) -> ()
                                }
                                }
                                }
                                }
                              }
                            }
                          }
                        }
                        frame #1 {
                          n588 = flat-sequence {
                            frame #0 {
                              n589 = local read "x-U-Scan Spannungsstart [V]"() -> (w346:dbl)
                              n590 = local read "Spannungskanal"() -> (w347:refnum<k21>)
                              n591 = local write "x-U-Scan aktuelle Spannung [V]"(w346) -> ()
                              n592 = call "HV_power_supply_set_voltage.vi"("Desired output voltage in V (HV power supply)"=w346, "Channel of HV power supply"=w347) -> ("error out"=w348:errorcluster)  [unwired: 8 in]
                              n593 = local write "Fehler (Ausgang)"(w348) -> ()
                            }
                            frame #1 {
                              # "Fahre nächste x-Position an"
                              n594 = local read "x-U-Scan x-Rasterschritt [µm]"() -> (w353:dbl)
                              n595 = local read "Achs-ID"() -> (w352:i32)
                              n596 = Decrement(x=w352) -> (x-1=w351:i32)
                              n597 = call "stage_move_axis_relative.vi"("Achse"=w352, "Schrittweite [µm]"=w353) -> ("xyz-Position OUT [mm]"=w350:dbl[])  [unwired: 1 in, 2 out]
                              n598 = Index Array(array=w350, index=w351) -> (element=w349:dbl)
                              n599 = local write "x-U-Scan aktuelle x-Position [mm]"(w349) -> ()
                            }
                            frame #2 {
                              n600 = local read "x-U-Scan (Ausgleichslage) Steigung"() -> (w355:dbl)
                              n601 = Not Equal?(x=w355, y=0.0) -> (x != y?=w356:bool)
                              n602 = case shown="True" w356 {
                                frame #0 {
                                }
                                frame #1 {
                                # "Fahre nächste y-Position an"
                                n603 = local read "Raum-Koordinate 2 (Lagenausgleich)"() -> (w357:enum16{"x-Achse", "y-Achse", "z-Achse"})
                                n604 = local read "x-U-Scan (Ausgleichslage) Steigung"() -> (w359:dbl)
                                n605 = local read "x-U-Scan x-Rasterschritt [µm]"() -> (w361:dbl)
                                n606 = Multiply(x=w361, y=w359) -> (x*y=w360:dbl)
                                n607 = Increment(x=w357) -> (x+1=w358:enum16{"x-Achse", "y-Achse", "z-Achse"})
                                n608 = call "stage_move_axis_relative.vi"("Achse"=w358, "Schrittweite [µm]"=w360) -> ("xyz-Position OUT [mm]"=w362:dbl[])  [unwired: 1 in, 2 out]
                                n609 = Index Array(array=w362, index=w357) -> (element=w363:dbl)
                                n610 = local write "x-U-Scan aktuelle y-Position [mm]"(w363) -> ()
                                }
                              }
                            }
                            frame #3 {
                              # "Wartezeit für\nStartspannung"
                              n611 = Wait (ms)(milliseconds to wait=u32 6000 ("Zu wartende ms")) -> ()  [unwired: 1 out]
                            }
                          }
                        }
                      }
                    }
                  }
                }
              }
              frame #1 {
                n612 = local read "x-U-Scan läuft"() -> (w365:bool)
                n613 = case shown="True" w365 {
                  frame #0 {
                    n614 = flat-sequence {
                      frame #0 {
                        # "Zur Ausgangsposition zurückfahren"
                        n615 = local read "x-U-Scan x-Startposition [mm]"() -> (w366:dbl)
                        n616 = local read "Aktuelle xyz-Position [mm]"() -> (w369:dbl[])
                        n617 = local read "Achs-ID"() -> (w367:i32)
                        n618 = local read "x-U-Scan Spannungsstart [V]"() -> (w373:dbl)
                        n619 = Decrement(x=w367) -> (x-1=w368:i32)
                        n620 = Replace Array Subset(array=w369, new element=w366, index=w368) -> (w370:dbl[])
                        n621 = local read "Detektionskamera"() -> (w377:T5)
                        n622 = local read "Buffer Interval"() -> (w376:u32)
                        n623 = call "stage_move_axis_absolute.vi"("Ziel xyz IN [mm]"=w370, "Achse"=w367) -> ("error out"=w371:errorcluster)  [unwired: 1 in, 2 out]
                        n624 = local write "x-U-Scan aktuelle Spannung [V]"(w373) -> ()
                        n625 = local read "Spannungskanal"() -> (w374:refnum<k21>)
                        n626 = call "camera_create_configuration.vi"("error in"=w371, "BufferInterval"=w376, "Session Out 2"=w377) -> ("Fehler (Ausgang)"=w375:errorcluster, "Ereignisregistrierung (Referenz)"=w378:refnum<event-registration>)  [unwired: 1 out]
                        n627 = local write "Ereignis: FrameDone?"(w378) -> ()
                        n628 = call "HV_power_supply_set_voltage.vi"("error in"=w375, "Desired output voltage in V (HV power supply)"=w373, "Channel of HV power supply"=w374) -> ("error out"=w372:errorcluster)  [unwired: 7 in]
                        n629 = local write "Fehler (Ausgang)"(w372) -> ()
                      }
                    }
                  }
                  frame #1 {
                    n630 = flat-sequence {
                      frame #0 {
                        n631 = local read "2D-Intensitätsverteilung (MCP)"() -> (w379:dbl[][])
                        n632 = control-ref of="2D-Intensitätsverteilung (MCP)"() -> (w382:refnum<vi>)
                        n633 = Array Max & Min(array=w379) -> (max value=w380:dbl, min value=w381:dbl)  [unwired: 2 out]
                        n634 = property class="IntGraph (strikt)"(reference=w382, "ZScale.Maximum"=w380, "ZScale.Minimum"=w381) -> ()  [unwired: 1 in, 2 out]
                      }
                      frame #1 {
                        # "Zur Ausgangsposition zurückfahren"
                        n635 = local read "Start xyz-Position [mm]"() -> (w387:dbl[])
                        n636 = local read "x-U-Scan Spannungsstart [V]"() -> (w392:dbl)
                        n637 = local read "x-U-Scan Spannungsstart [V]"() -> (w390:dbl)
                        n638 = local read "Detektionskamera"() -> (w395:T5)
                        n639 = local read "Achs-ID"() -> (w384:i32)
                        n640 = local read "Buffer Interval"() -> (w394:u32)
                        n641 = local read "Spannungskanal"() -> (w391:refnum<k21>)
                        n642 = Decrement(x=w384) -> (x-1=w385:i32)
                        n643 = call "stage_move_axis_absolute.vi"("Ziel xyz IN [mm]"=w387, "Achse"=w384) -> ("error out"=w388:errorcluster, "Ziel xyz OUT [mm]"=w386:dbl[])  [unwired: 1 in, 1 out]
                        n644 = local write "x-U-Scan aktuelle Spannung [V]"(w392) -> ()
                        n645 = call "camera_create_configuration.vi"("error in"=w388, "BufferInterval"=w394, "Session Out 2"=w395) -> ("Fehler (Ausgang)"=w389:errorcluster, "Ereignisregistrierung (Referenz)"=w396:refnum<event-registration>)  [unwired: 1 out]
                        n646 = Index Array(array=w386, index=w385) -> (element=w383:dbl)
                        n647 = local write "x-U-Scan aktuelle x-Position [mm]"(w383) -> ()
                        n648 = local write "x-U-Scan aktuelle Spannung [V]"(w390) -> ()
                        n649 = local write "Ereignis: FrameDone?"(w396) -> ()
                        n650 = call "HV_power_supply_set_voltage.vi"("error in"=w389, "Desired output voltage in V (HV power supply)"=w390, "Channel of HV power supply"=w391) -> ("error out"=w393:errorcluster)  [unwired: 7 in]
                        n651 = local write "Fehler (Ausgang)"(w393) -> ()
                      }
                      frame #2 {
                        n652 = local read "x-U-Scan (Ausgleichslage) Steigung"() -> (w398:dbl)
                        n653 = Not Equal?(x=w398, y=0.0) -> (x != y?=w397:bool)
                        n654 = case shown="True" w397 {
                          frame #0 {
                          }
                          frame #1 {
                            n655 = local read "Raum-Koordinate 2 (Lagenausgleich)"() -> (w400:enum16{"x-Achse", "y-Achse", "z-Achse"})
                            n656 = local read "Start xyz-Position [mm]"() -> (w402:dbl[])
                            n657 = Increment(x=w400) -> (x+1=w401:enum16{"x-Achse", "y-Achse", "z-Achse"})
                            n658 = call "stage_move_axis_absolute.vi"("Ziel xyz IN [mm]"=w402, "Achse"=w401) -> ("Ziel xyz OUT [mm]"=w403:dbl[])  [unwired: 1 in, 2 out]
                            n659 = Index Array(array=w403, index=w400) -> (element=w404:dbl)
                            n660 = local write "x-U-Scan aktuelle y-Position [mm]"(w404) -> ()
                          }
                        }
                      }
                      frame #3 {
                        n661 = local read "Daten speichern"() -> (w405:bool)
                        n662 = case shown="True" w405 {
                          frame #0 {
                          }
                          frame #1 {
                            n663 = local read "x-U-Scan x-Rasterschritt [µm]"() -> (w413:dbl)
                            n664 = local read "x-U-Scan (Ausgleichslage) Steigung"() -> (w407:dbl)
                            n665 = local read "x-U-Scan Spannungsschritt [V]"() -> (w416:dbl)
                            n666 = local read "# x-U-Scan Spannungsschritte"() -> (w415:i32)
                            n667 = local read "x-U-Scan x-Startposition [mm]"() -> (w414:dbl)
                            n668 = local read "x-U-Scan Spannungsstart [V]"() -> (w417:dbl)
                            n669 = local read "# x-U-Scan x-Rasterschritte"() -> (w409:i32)
                            n670 = Divide(x=w413, y=1000.0) -> (x/y=w410:dbl)
                            n671 = local read "Save folder"() -> (w411:string)
                            n672 = Not Equal?(x=w407, y=0.0) -> (x != y?=w408:bool)
                            n673 = local read "2D-Intensitätsverteilung (MCP)"() -> (w424:dbl[][])
                            n674 = call "create_axis_vector_file.vi"("Save folder"=w411, "Dateiname"="yAchse.dat", "Start"=w417, "Schrittlänge"=w416, "# Schritte"=w415) -> ()  [unwired: 11 in]
                            n675 = case shown="True" w408 {
                              tunnel: w411 -> [_ w432]
                              tunnel: w410 -> [_ w429]
                              tunnel: w409 -> [_ w426]
                              frame #0 {
                              }
                              frame #1 {
                                n676 = local read "x-U-Scan (Ausgleichslage) Steigung"() -> (w430:dbl)
                                n677 = local read "x-U-Scan y-Startposition [mm]"() -> (w427:dbl)
                                n678 = Multiply(x=w429, y=w430) -> (x*y=w428:dbl)
                                n679 = call "create_axis_vector_file.vi"("Save folder"=w432, "Dateiname"="zAchse.dat", "Start"=w427, "Schrittlänge"=w428, "# Schritte"=w426) -> ()  [unwired: 11 in]
                              }
                            }
                            n680 = call "create_axis_vector_file.vi"("Save folder"=w411, "Dateiname"="xAchse.dat", "Start"=w414, "Schrittlänge"=w410, "# Schritte"=w409) -> ()  [unwired: 11 in]
                            n681 = Concatenate Strings(w411, "\\" ("String"), "2D_Intensitaetsverteilung_MCP.dat" ("String")) -> (w421:string)
                            n682 = String To Path(string=w421) -> (path=w422:path)
                            n683 = call-poly <vilib>:"Write To Spreadsheet File.vi"("format (%.3f)"="%.;%8.0f", "2D data"=w424, "file path (dialog if empty)"=w422) -> ()  [unwired: 5 in, 1 out]
                          }
                        }
                      }
                      frame #4 {
                        w433 = FALSE ("Spannungsscan läuft")
                        n684 = local write "x-U-Scan ON/OFF"(w433) -> ()
                        n685 = local write "x-U-Scan läuft"(w433) -> ()
                      }
                    }
                  }
                }
              }
            }
          }
        }
        n686 = Unbundle By Name(w256) -> ("status"=w257:bool)
        n687 = Or(x=w257, y=w258) -> (x .or. y?=w255:bool)
      }
      n688 = while "Mess-Schleife" {
        tunnel: w63 -> [w666]
        i -> [w665]
        stop <- w664 stop-if-true
        n689 = event "Scan-Ereignisse" shown="[3] <Event: Rasterung gestartet?>: Benutzerereignis" {
          selector: w666 -> [_ _ _ _ _ _ _ _ _ _]
          dyn-events: _ -> [_ _ _ _ _ _ _ _ _ _]
          timeout: 1000 -> [_ _ _ _ _ _ _ _ _ _]
          event #0 {
            n690 = event-data() -> ()  [unwired: 1 in, 2 out]
          }
          event #1 {
            n691 = event-data() -> ("NewVal"=w673:bool)  [unwired: 1 in]
            n692 = local read "Kamera"() -> (w672:bool)
            n693 = And(x=w672, y=w673) -> (x .and. y?=w671:bool)
            n694 = case shown="True" w671 {
              frame #0 {
                n695 = local write "Rasterung läuft"(FALSE ("Rasterung läuft")) -> ()
              }
              frame #1 {
                n696 = stacked-sequence {
                  frame #0 {
                    n697 = flat-sequence {
                      tunnel: [w685] -> w675
                      tunnel: w675 -> [w753]
                      frame #0 {
                        n698 = Get Date/Time In Seconds() -> (seconds since 1Jan1904=w676:timestamp)
                        n699 = local write "Start time [ms]"(w676) -> ()
                        n700 = local read "Rasterweite [µm]"() -> (w696:dbl[])
                        n701 = local read "# Rasterschritte"() -> (w698:i32[])
                        n702 = control-ref of="Shutter time (ms)"() -> (w693:refnum<vi>)
                        n703 = local read "Rasterart"() -> (w699:T2)
                        n704 = property class="Ring (strikt)"(reference=w693) -> ("RingText.Text"=w692:string)  [unwired: 1 in, 2 out]
                        n705 = case shown="\"2D-Scan(xz)\"" w699 {
                          tunnel: w698 -> [w707 w723 w728 w737 w743]
                          tunnel: [w706 w722 w729 w736 w740] -> w697
                          tunnel: w696 -> [w705 w713 w725 w733 w742]
                          tunnel: [w704 w712 w724 w732 w741] -> w695
                          frame #0 {
                            n706 = Replace Array Subset(array=w707, new element #1=1 ("Neues Element/Teil-Array"), index #1=1 ("Index"), new element #2=1 ("Neues Element/Teil-Array"), index #2=2 ("Index")) -> (w706:i32[])
                            n707 = Replace Array Subset(array=w705, new element #1=0.0 ("Neues Element/Teil-Array"), index #1=1 ("Index"), new element #2=0.0 ("Neues Element/Teil-Array"), index #2=2 ("Index")) -> (w704:dbl[])
                          }
                          frame #1 {
                            n708 = Replace Array Subset(array=w723, new element #1=1 ("Neues Element/Teil-Array"), index #1=0 ("Index"), new element #2=1 ("Neues Element/Teil-Array"), index #2=1 ("Index")) -> (w722:i32[])
                            n709 = Replace Array Subset(array=w713, new element #1=0.0 ("Neues Element/Teil-Array"), index #1=0 ("Index"), new element #2=0.0 ("Neues Element/Teil-Array"), index #2=1 ("Index")) -> (w712:dbl[])
                          }
                          frame #2 {
                            n710 = Replace Array Subset(array=w728, new element=1 ("Neues Element/Teil-Array"), index=2 ("Index")) -> (w729:i32[])
                            n711 = Replace Array Subset(array=w725, new element=0.0 ("Neues Element/Teil-Array"), index=2 ("Index")) -> (w724:dbl[])
                          }
                          frame #3 {
                            n712 = Replace Array Subset(array=w737, new element=1 ("Neues Element/Teil-Array"), index=0 ("Index")) -> (w736:i32[])
                            n713 = Replace Array Subset(array=w733, new element=0.0 ("Neues Element/Teil-Array"), index=0 ("Index")) -> (w732:dbl[])
                          }
                          frame #4 {
                            n714 = Replace Array Subset(array=w743, new element=1 ("Neues Element/Teil-Array"), index=1 ("Index")) -> (w740:i32[])
                            n715 = Replace Array Subset(array=w742, new element=0.0 ("Neues Element/Teil-Array"), index=1 ("Index")) -> (w741:dbl[])
                          }
                        }
                        n716 = local read "# Bilder/Messschritt"() -> (w691:i32)
                        n717 = control-ref of="Rasterart"() -> (w694:refnum<vi>)
                        n718 = Decimal String To Number(string=w692) -> (number=w689:i32)  [unwired: 2 in, 1 out]
                        n719 = local read "Suppressor-Spannung [V]"() -> (w678:dbl)
                        n720 = local read "P-Schirm-Spannung [V]"() -> (w683:dbl)
                        n721 = local read "MCP-Spannung [V]"() -> (w682:dbl)
                        n722 = property class="Enum (strikt)"(reference=w694) -> ("RingText.Text"=w680:string)  [unwired: 1 in, 2 out]
                        n723 = local read "Leistung (iK) [mW]"() -> (w681:dbl)
                        n724 = local read "Tip-Spannung [V]"() -> (w677:dbl)
                        n725 = local read "Polarisation [°]"() -> (w686:dbl)
                        n726 = Multiply(x=w691, y=w689) -> (x*y=w690:i32)
                        n727 = local read "Messlogbuch"() -> (w688:path)
                        n728 = local read "Proben-ID"() -> (w687:string)
                        n729 = local read "ROI"() -> (w679:i32[])
                        n730 = local write "Rasterweite [µm]"(w695) -> ()
                        n731 = local write "# Rasterschritte"(w697) -> ()
                        n732 = call "stage_get_current_xyz.vi"() -> ("Aktuelle xyz-Position OUT [mm]"=w684:dbl[])  [unwired: 3 in, 1 out]
                        n733 = call "create_measure_log_entry.vi"("Messlogbuch-Pfad"=w688, "Probe"=w687, "Polarisation [°]"=w686, "Messart"=w680, "ROI"=w679, "Messungen/Messschritt"=w691, "Maximalleistung (iK) [mW]"=w681, "Tip-Spannung [V]"=w677, "Suppressor-Spannung [V]"=w678, "Zeit/Messschritt [ms]"=w689, "MCP-Spannung [V]"=w682, "Zeit/Messung [ms]"=w690, "Phosphorschirm-Spannung [V]"=w683, "xyz [mm]"=w684) -> ("Messung Nr."=w685:i32)  [unwired: 4 in, 1 out]
                      }
                      frame #1 {
                        n734 = local write "Aktueller Messschritt"(0 ("Aktueller Messschritt")) -> ()
                        n735 = local read "Fehler (Ausgang)"() -> (w754:errorcluster)
                        n736 = local read "Rasterweite [µm]"() -> (w779:dbl[])
                        n737 = local read "# Rasterschritte"() -> (w778:i32[])
                        n738 = local read "# Rasterschritte"() -> (w776:i32[])
                        n739 = local read "Day folder"() -> (w759:string)
                        n740 = Divide(x=w779, y=w778) -> (x/y=w777:dbl[])
                        n741 = local read "Summierte Helligkeit speichern"() -> (w751:bool)
                        n742 = Index Array(array=w776, index #1=0 ("Index"), index #2=1 ("Index"), index #3=2 ("Index")) -> (element #1=w773:i32, element #2=w772:i32, element #3=w771:i32)
                        n743 = local read "Gemittelte Bilder speichern"() -> (w749:bool)
                        n744 = local read "LAPD-Daten speichern"() -> (w748:bool)
                        n745 = local read "Einzelbilder speichern"() -> (w750:bool)
                        n746 = local read "Einzelbilder speichern"() -> (w762:bool)
                        n747 = local write "Rasterschritt [µm]"(w777) -> ()
                        n748 = call "create_save_folder.vi"("Day folder"=w759, "Measuring number"=w753, "Measuring folder"="Rasterung" ("Subfolder"), "error in"=w754) -> ("Save Folder"=w758:string, "Error Out"=w757:errorcluster)  [unwired: 5 in]
                        n749 = Multiply(x=w773, y=w772) -> (x*y=w770:i32)
                        n750 = local write "Save folder"(w758) -> ()
                        n751 = case shown="True" w762 {
                          tunnel: w757 -> [w780 w782]
                          tunnel: [w780 w781] -> w756
                          frame #0 {
                          }
                          frame #1 {
                            n752 = local read "Save folder"() -> (w785:string)
                            n753 = Concatenate Strings(w785, "\\Einzelbilder" ("Subfolder")) -> (w783:string)
                            n754 = String To Path(string=w783) -> (path=w786:path)
                            n755 = call <vilib>:"Check if File or Folder Exists.vi"("error in (no error)"=w782, "path"=w786) -> ("error out"=w781:errorcluster, "file or folder exists?"=w787:bool, "dup path"=w788:path)  [unwired: 7 in]
                            n756 = case shown="False" w787 {
                              tunnel: w788 -> [w789 _]
                              frame #0 {
                                n757 = Create Folder(path (use dialog)=w789) -> ()  [unwired: 2 in, 3 out]
                              }
                              frame #1 {
                              }
                            }
                          }
                        }
                        n758 = Compound Arithmetic op=OR(w749, w750, w751, w748) -> (w752:bool)
                        n759 = local write "Daten speichern"(w752) -> ()
                        n760 = Multiply(x=w770, y=w771) -> (x*y=w769:i32)
                        n761 = local write "# Messschritte"(w769) -> ()
                        n762 = local read "Gemittelte Bilder speichern"() -> (w763:bool)
                        n763 = case shown="True" w763 {
                          tunnel: w756 -> [w790 w792]
                          tunnel: [w790 w791] -> w755
                          frame #0 {
                          }
                          frame #1 {
                            n764 = local read "Save folder"() -> (w796:string)
                            n765 = Concatenate Strings(w796, "\\Gemittelte Bilder" ("Subfolder")) -> (w798:string)
                            n766 = String To Path(string=w798) -> (path=w795:path)
                            n767 = call <vilib>:"Check if File or Folder Exists.vi"("error in (no error)"=w792, "path"=w795) -> ("error out"=w791:errorcluster, "file or folder exists?"=w794:bool, "dup path"=w793:path)  [unwired: 7 in]
                            n768 = case shown="False" w794 {
                              tunnel: w793 -> [w799 _]
                              frame #0 {
                                n769 = Create Folder(path (use dialog)=w799) -> ()  [unwired: 2 in, 3 out]
                              }
                              frame #1 {
                              }
                            }
                          }
                        }
                        n770 = local read "Kamera"() -> (w765:bool)
                        n771 = case shown="True" w765 {
                          tunnel: [w800 w802] -> w764
                          tunnel: w755 -> [w800 w801]
                          frame #0 {
                          }
                          frame #1 {
                            n772 = local read "Ereignis: FrameDone?"() -> (w803:refnum<event-registration>)
                            n773 = local read "Detektionskamera"() -> (w804:T5)
                            n774 = call "camera_release_configuration.vi"("error in"=w801, "Session In"=w804, "Ereignisregistrierung (Referenz) 2"=w803) -> ("error out"=w802:errorcluster)  [unwired: 1 out]
                          }
                        }
                        n775 = call "stage_get_current_xyz.vi"("error in"=w764) -> ("error out"=w761:errorcluster, "Aktuelle xyz-Position OUT [mm]"=w766:dbl[])  [unwired: 2 in]
                        n776 = local write "Start xyz-Position [mm]"(w766) -> ()
                        n777 = local write "Fehler (Ausgang)"(w761) -> ()
                      }
                    }
                  }
                  frame #1 {
                    n778 = flat-sequence {
                      tunnel: [w819] -> w815
                      tunnel: [w818] -> w814
                      tunnel: [w817] -> w813
                      tunnel: [w817] -> w812
                      tunnel: [w817] -> w811
                      tunnel: [w817] -> w810
                      tunnel: [w817] -> w809
                      tunnel: [w816] -> w808
                      tunnel: [w817] -> w807
                      tunnel: [w817] -> w806
                      tunnel: [w816] -> w805
                      tunnel: w815 -> [w833]
                      tunnel: w814 -> [w843]
                      tunnel: w813 -> [w842]
                      tunnel: w812 -> [w841]
                      tunnel: w811 -> [w840]
                      tunnel: w810 -> [w839]
                      tunnel: w809 -> [w838]
                      tunnel: w808 -> [w837]
                      tunnel: w807 -> [w836]
                      tunnel: w806 -> [w835]
                      tunnel: w805 -> [w834]
                      frame #0 {
                        n779 = local read "Rasterart"() -> (w820:T2)
                        n780 = case shown="\"2D-Scan(yz)\"" w820 {
                          tunnel: [0 ("Index") 2 ("Index") 0 ("Index")] -> w816
                          tunnel: [1 ("Index") 1 ("Index") 2 ("Index")] -> w817
                          tunnel: ["x-Position [mm]" ("X-Achse.Namensbeschriftung.Text") "z-Position [mm]" ("Y-Achse.Namensbeschriftung.Text") "x-Position [mm]" ("Y-Achse.Namensbeschriftung.Text")] -> w819
                          tunnel: ["y-Position [mm]" ("Y-Achse.Namensbeschriftung.Text") "y-Position [mm]" ("X-Achse.Namensbeschriftung.Text") "z-Position [mm]" ("X-Achse.Namensbeschriftung.Text")] -> w818
                          frame #0 {
                          }
                          frame #1 {
                          }
                          frame #2 {
                          }
                        }
                      }
                      frame #1 {
                        w851 = 1000.0 ("y")
                        w870 = 1000.0 ("y")
                        n781 = local read "Rasterweite [µm]"() -> (w875:dbl[])
                        n782 = local read "Rasterweite [µm]"() -> (w846:dbl[])
                        n783 = local read "# Rasterschritte"() -> (w879:i32[])
                        n784 = local read "# Rasterschritte"() -> (w868:i32[])
                        n785 = local read "# Rasterschritte"() -> (w853:i32[])
                        n786 = local read "Start xyz-Position [mm]"() -> (w874:dbl[])
                        n787 = local read "Start xyz-Position [mm]"() -> (w847:dbl[])
                        n788 = Index Array(array=w879, index #1=w837, index #2=w842) -> (element #1=w877:i32, element #2=w878:i32)
                        n789 = Index Array(array=w875, index #1=w837, index #2=w836) -> (element #1=w871:dbl, element #2=w872:dbl)
                        n790 = Index Array(array=w868, index #1=w837, index #2=w841) -> (element #1=w864:i32, element #2=w866:i32)
                        n791 = Index Array(array=w846, index #1=w837, index #2=w838) -> (element #1=w850:dbl, element #2=w849:dbl)
                        n792 = Index Array(array=w853, index #1=w837, index #2=w840) -> (element #1=w857:i32, element #2=w855:i32)
                        n793 = Divide(x=w871, y=w870) -> (x/y=w865:dbl)
                        n794 = Divide(x=w872, y=w870) -> (x/y=w867:dbl)
                        n795 = Divide(x=w850, y=w851) -> (x/y=w856:dbl)
                        n796 = Divide(x=w849, y=w851) -> (x/y=w854:dbl)
                        n797 = control-ref of="2D-Intensitätsverteilung (MCP)"() -> (w876:refnum<vi>)
                        n798 = Index Array(array=w874, index #1=w834, index #2=w835) -> (element #1=w873:dbl, element #2=w869:dbl)
                        n799 = Index Array(array=w847, index #1=w837, index #2=w839) -> (element #1=w848:dbl, element #2=w852:dbl)
                        n800 = Initialize Array(0.0 ("y"), w877, w878) -> (w860:dbl[][])
                        n801 = local write "2D-Intensitätsverteilung (LAPD)"(w860) -> ()
                        n802 = local write "2D-Intensitätsverteilung (MCP)"(w860) -> ()
                        n803 = Divide(x=w856, y=w857) -> (x/y=w858:dbl)
                        n804 = Divide(x=w854, y=w855) -> (x/y=w859:dbl)
                        n805 = Divide(x=w865, y=w864) -> (x/y=w863:dbl)
                        n806 = Divide(x=w867, y=w866) -> (x/y=w862:dbl)
                        n807 = property class="IntGraph (strikt)"(reference=w876, "XScale.Offset"=w873, "XScale.Multiplier"=w863, "YScale.Offset"=w869, "YScale.Multiplier"=w862, "XScale.MinorInc"=w863, "YScale.MinorInc"=w862, "XScale.NameLbl.Text"=w833, "YScale.NameLbl.Text"=w843) -> (error out=w880:errorcluster)  [unwired: 1 in, 1 out]
                        n808 = control-ref of="2D-Intensitätsverteilung (LAPD)"() -> (w844:refnum<vi>)
                        n809 = property class="IntGraph (strikt)"(reference=w844, error in=w880, "XScale.Offset"=w848, "XScale.Multiplier"=w858, "YScale.Offset"=w852, "YScale.Multiplier"=w859, "XScale.MinorInc"=w858, "YScale.MinorInc"=w859, "XScale.NameLbl.Text"=w833, "YScale.NameLbl.Text"=w843) -> (error out=w845:errorcluster)  [unwired: 1 out]
                        n810 = local write "Fehler (Ausgang)"(w845) -> ()
                      }
                    }
                  }
                  frame #2 {
                    n811 = local write "Rasterung läuft"(TRUE ("x-Linsescan")) -> ()
                    n812 = local read "Event: Rasterung gestartet?"() -> (w884:refnum<user-event>)
                    n813 = local read "Aktueller Messschritt"() -> (w883:i32)
                    n814 = Generate User Event(user event=w884, event data cluster=w883) -> (user event out=w882:refnum<user-event>)  [unwired: 1 in, 1 out]
                    n815 = local write "Event: Rasterung gestartet?"(w882) -> ()
                  }
                }
              }
            }
          }
          event #2 {
            n816 = event-data() -> ()  [unwired: 1 in, 1 out]
            n817 = local read "Rasterweite [µm]"() -> (w886:dbl[])
            n818 = local read "# Rasterschritte"() -> (w897:i32[])
            n819 = Replace Array Subset(array=w897, new element #1=1 ("Neues Element/Teil-Array"), index #1=0 ("Index"), new element #2=1 ("Neues Element/Teil-Array"), index #2=1 ("Index"), new element #3=1 ("Neues Element/Teil-Array"), index #3=2 ("Index")) -> (w893:i32[])
            n820 = Replace Array Subset(array=w886, new element #1=0 ("Neues Element/Teil-Array"), index #1=0 ("Index"), new element #2=0 ("Neues Element/Teil-Array"), index #2=1 ("Index"), new element #3=0 ("Neues Element/Teil-Array"), index #3=2 ("Index")) -> (w885:dbl[])
            n821 = local write "Rasterweite [µm]"(w885) -> ()
            n822 = local write "# Rasterschritte"(w893) -> ()
          }
          event #3 {
            n823 = event-data() -> ()  [unwired: 1 in, 1 out]
            n824 = stacked-sequence {
              frame #0 {
                n825 = while "x-Schleife" {
                  i -> [w903]
                  stop <- w904 stop-if-true
                  n826 = stacked-sequence {
                    frame #0 {
                      n827 = while "z-Schleife" {
                        i -> [w911]
                        stop <- w913 stop-if-true
                        n828 = stacked-sequence {
                          frame #0 {
                            n829 = while "y-Schleife" {
                              i -> [w922]
                              stop <- w928 stop-if-true
                              # "Schleife für y-Achse"
                              n830 = stacked-sequence {
                                frame #0 {
                                # "Hier findet die Messung statt"
                                n831 = stacked-sequence {
                                frame #0 {
                                n832 = local write "Summierte Helligkeit (a.u.)"(u64 0 ("Summierte Helligkeit (a.u.)")) -> ()
                                n833 = local write "LAPD Spannung (V)"(0.0 ("Transmittierte Intensität (a.u.)")) -> ()
                                n834 = local read "ROI"() -> (w935:i32[])
                                n835 = Index Array(array=w935, index #1=0 ("Index"), index #2=1 ("Index")) -> (element #1=w931:i32, element #2=w932:i32)
                                n836 = local read "Aktueller Messschritt"() -> (w938:i32)
                                n837 = Initialize Array(u64 0 ("Element"), w932, w931) -> (w937:u64[][])
                                n838 = local write "Gemitteltes Bild"(w937) -> ()
                                n839 = Increment(x=w938) -> (x+1=w939:i32)
                                n840 = local write "Aktueller Messschritt"(w939) -> ()
                                }
                                frame #1 {
                                n841 = local read "# Photosignale"() -> (w949:i32)
                                n842 = local read "# Bilder/Messschritt"() -> (w945:i32)
                                n843 = local read "Detektionskamera"() -> (w948:T5)
                                n844 = for {
                                N: w949 -> [_]
                                n845 = Wait (ms)(milliseconds to wait=u32 10 ("Zu wartende ms")) -> ()  [unwired: 1 out]
                                n846 = local read "LAPD-Kanal (Meilhaus)"() -> (w963:u32)
                                n847 = local read "LAPD Spannung (V)"() -> (w968:dbl)
                                n848 = call "IOcard_analog_input_Meilhaus.vi"("Channel"=w963, "Device"=u32 0 ("Board Number")) -> ("Voltage [V]"=w965:dbl)  [unwired: 9 in]
                                n849 = Add(x=w965, y=w968) -> (x+y=w967:dbl)
                                n850 = local write "LAPD Spannung (V)"(w967) -> ()
                                }
                                n851 = local read "Einzelbilder speichern"() -> (w943:bool)
                                n852 = call "camera_acquisition_sequence.vi"("Session In"=w948, "Desired image number"=w945) -> ("Image Array"=w942:T4[], "error out"=w947:errorcluster)  [unwired: 2 in, 1 out]
                                n853 = case shown="True" w943 {
                                tunnel: w947 -> [w951 w959]
                                tunnel: [w951 w958] -> w946
                                tunnel: w945 -> [w950 w957]
                                tunnel: [w950 w957] -> w944
                                tunnel: w942 -> [_ w956]
                                frame #0 {
                                }
                                frame #1 {
                                n854 = local read "Aktueller Messschritt"() -> (w962:i32)
                                n855 = local read "Save folder"() -> (w954:string)
                                n856 = Concatenate Strings(w954, "Einzelbilder\\" ("String")) -> (w952:string)
                                n857 = Format Into String(format string="%05.0f" ("Format-String"), initial string="#" ("Eingangs-String"), w962) -> (resulting string=w955:string)  [unwired: 1 in, 1 out]
                                n858 = call "save images.vi"("Save Folder"=w952, "File name prefix"=w955, "Array"=w956, "error out 2"=w959, "Bilder/Messschritt"=w957) -> ("error out"=w958:errorcluster)
                                }
                                }
                                n859 = for {
                                N: w944 -> [_]
                                tunnel: w946 -> [w977]
                                tunnel: w942 -> [w975] mode=indexing
                                n860 = call "IMAQ ImageToArray"("error in (no error)"=w977, "Image"=w975) -> ("error out"=w976:errorcluster, "Image Pixels (U8)"=w974:u8[][])  [unwired: 2 in, 3 out]
                                n861 = local write "Fehler (Ausgang)"(w976) -> ()
                                n862 = To Quad Integer(1:w974) -> (0:w978:i64[][])
                                n863 = local read "Gemitteltes Bild"() -> (w972:u64[][])
                                n864 = Add Array Elements(numeric array=w978) -> (sum=w971:i64)
                                n865 = local read "Summierte Helligkeit (a.u.)"() -> (w979:i64)
                                n866 = Add(x=w972, y=w974) -> (x+y=w973:u64[][])
                                n867 = local write "Gemitteltes Bild"(w973) -> ()
                                n868 = local read "Hintergrund-Helligkeit"() -> (w969:i64)
                                n869 = Subtract(x=w971, y=w969) -> (x-y=w970:i64)
                                n870 = Add(x=w970, y=w979) -> (x+y=w980:i64)
                                n871 = local write "Summierte Helligkeit (a.u.)"(w980) -> ()
                                }
                                }
                                frame #2 {
                                n872 = local read "Rasterart"() -> (w990:T2)
                                n873 = case shown="\"2D-Scan(xz)\"" w990 {
                                tunnel: [w1012 w1013 w1015 w1016 w1018] -> w989
                                tunnel: [w1011 w1014 w1015 w1016 w1017] -> w988
                                frame #0 {
                                n874 = local read "Current y step"() -> (w1011:i32)
                                n875 = local read "Current x step"() -> (w1012:i32)
                                }
                                frame #1 {
                                n876 = local read "Current z step"() -> (w1013:i32)
                                n877 = local read "Current y step"() -> (w1014:i32)
                                }
                                frame #2 {
                                n878 = local read "Current z step"() -> (w1015:i32)
                                }
                                frame #3 {
                                n879 = local read "Current x step"() -> (w1016:i32)
                                }
                                frame #4 {
                                n880 = local read "Current z step"() -> (w1017:i32)
                                n881 = local read "Current x step"() -> (w1018:i32)
                                }
                                }
                                n882 = local read "# Bilder/Messschritt"() -> (w985:i32)
                                n883 = local read "Gemitteltes Bild"() -> (w987:u64[][])
                                n884 = local read "LAPD Spannung (V)"() -> (w996:dbl)
                                n885 = local read "# Photosignale"() -> (w995:i32)
                                n886 = local read "Image Display"() -> (w983:T4)
                                n887 = Divide(x=w987, y=w985) -> (x/y=w986:dbl[][])
                                n888 = local read "2D-Intensitätsverteilung (LAPD)"() -> (w991:dbl[][])
                                n889 = local read "2D-Intensitätsverteilung (MCP)"() -> (w992:dbl[][])
                                n890 = local read "Gemittelte Bilder speichern"() -> (w981:bool)
                                n891 = local read "Summierte Helligkeit (a.u.)"() -> (w997:i64)
                                n892 = Divide(x=w996, y=w995) -> (x/y=w993:dbl)
                                n893 = call "IMAQ ArrayToImage"("Image Pixels (U8)"=w986, "Image"=w983) -> ("Image Out"=w984:T4)  [unwired: 8 in, 1 out]
                                n894 = local write "LAPD Spannung (V)"(w993) -> ()
                                n895 = Replace Array Subset(array=w992, new element=w997, index (row)=w989, index (col)=w988) -> (w998:dbl[][])
                                n896 = Replace Array Subset(array=w991, new element=w993, index (row)=w989, index (col)=w988) -> (w994:dbl[][])
                                n897 = case shown="True" w981 {
                                tunnel: w984 -> [w999 w1010]
                                tunnel: [w999 w1001] -> w982
                                frame #0 {
                                }
                                frame #1 {
                                n898 = local read "Aktueller Messschritt"() -> (w1005:i32)
                                n899 = local read "Save folder"() -> (w1007:string)
                                n900 = Format Into String(format string="%05.0f" ("Format-String"), initial string="#" ("Eingangs-String"), w1005) -> (resulting string=w1004:string)  [unwired: 1 in, 1 out]
                                n901 = Concatenate Strings(w1007, "Gemittelte Bilder\\" ("String"), w1004, ".png" ("String")) -> (w1003:string)
                                n902 = String To Path(string=w1003) -> (path=w1002:path)
                                n903 = call-poly "IMAQ Write File 2"("File Path"=w1002, "Image"=w1010) -> ("Image Out (duplicate)"=w1001:T4)  [unwired: 8 in, 1 out]
                                }
                                }
                                n904 = local write "2D-Intensitätsverteilung (MCP)"(w998) -> ()
                                n905 = local write "2D-Intensitätsverteilung (LAPD)"(w994) -> ()
                                n906 = local write "Image Display"(w982) -> ()
                                }
                                }
                                }
                                frame #1 {
                                n907 = local read "y-Achse"() -> (w1024:i32)
                                n908 = local read "Aktueller Messschritt"() -> (w1021:i32)
                                n909 = local read "Rasterschritt [µm]"() -> (w1028:dbl[])
                                n910 = local read "Start time [ms]"() -> (w1022:timestamp)
                                n911 = local read "# Messschritte"() -> (w1020:i32)
                                n912 = Decrement(x=w1024) -> (x-1=w1027:i32)
                                n913 = Index Array(array=w1028, index=w1027) -> (element=w1023:dbl)
                                n914 = call "estimate_stopp_time.vi"("Aktueller Messschritt"=w1021, "# Messschritte"=w1020, "Startzeit"=w1022) -> ("Stopp Zeit"=w1019:string)  [unwired: 8 in]
                                n915 = local write "Geschätzte Messzeit"(w1019) -> ()
                                n916 = Not Equal?(x=w1023, y=0.0) -> (x != y?=w1025:bool)
                                n917 = case shown="True" w1025 {
                                tunnel: w1024 -> [_ w1030]
                                tunnel: w1023 -> [_ w1029]
                                frame #0 {
                                }
                                frame #1 {
                                # "Fahre nächste y-Position an"
                                n918 = call "stage_move_axis_relative.vi"("Achse"=w1030, "Schrittweite [µm]"=w1029) -> ("error out"=w1032:errorcluster, "xyz-Position OUT [mm]"=w1031:dbl[])  [unwired: 1 in, 1 out]
                                n919 = local write "Aktuelle xyz-Position [mm]"(w1031) -> ()
                                n920 = local write "Fehler (Ausgang)"(w1032) -> ()
                                }
                                }
                                }
                              }
                              n921 = local read "y-Achse"() -> (w921:i32)
                              n922 = local read "# Rasterschritte"() -> (w927:i32[])
                              n923 = Decrement(x=w921) -> (x-1=w923:i32)
                              n924 = local read "Rasterung ON/OFF"() -> (w929:bool)
                              n925 = Increment(x=w922) -> (x+1=w924:i32)
                              n926 = Index Array(array=w927, index=w923) -> (element=w926:i32)
                              n927 = Equal?(x=w926, y=w924) -> (x = y?=w925:bool)
                              n928 = Not(x=w929) -> (.not. x?=w930:bool)
                              n929 = Or(x=w925, y=w930) -> (x .or. y?=w928:bool)
                              "Current y step" <- w922
                            }
                          }
                          frame #1 {
                            n930 = flat-sequence {
                              frame #0 {
                                n931 = local read "Rasterschritt [µm]"() -> (w1039:dbl[])
                                n932 = local read "y-Achse"() -> (w1034:i32)
                                n933 = Decrement(x=w1034) -> (x-1=w1038:i32)
                                n934 = local read "Start xyz-Position [mm]"() -> (w1033:dbl[])
                                n935 = Index Array(array=w1039, index=w1038) -> (element=w1037:dbl)
                                n936 = Not Equal?(x=w1037, y=0.0) -> (x != y?=w1035:bool)
                                n937 = case shown="True" w1035 {
                                tunnel: w1034 -> [_ w1041]
                                tunnel: w1033 -> [_ w1040]
                                frame #0 {
                                }
                                frame #1 {
                                # "Fahre Startposition für y an"
                                n938 = call "stage_move_axis_absolute.vi"("Ziel xyz IN [mm]"=w1040, "Achse"=w1041) -> ("error out"=w1043:errorcluster, "Ziel xyz OUT [mm]"=w1042:dbl[])  [unwired: 1 in, 1 out]
                                n939 = local write "Aktuelle xyz-Position [mm]"(w1042) -> ()
                                n940 = local write "Fehler (Ausgang)"(w1043) -> ()
                                }
                                }
                              }
                              frame #1 {
                                n941 = local read "Rasterschritt [µm]"() -> (w1049:dbl[])
                                n942 = local read "z-Achse"() -> (w1044:i32)
                                n943 = Decrement(x=w1044) -> (x-1=w1045:i32)
                                n944 = Index Array(array=w1049, index=w1045) -> (element=w1046:dbl)
                                n945 = Not Equal?(x=w1046, y=0.0) -> (x != y?=w1047:bool)
                                n946 = case shown="True" w1047 {
                                tunnel: w1046 -> [_ w1051]
                                tunnel: w1044 -> [_ w1050]
                                frame #0 {
                                }
                                frame #1 {
                                # "Fahre nächste Position für z an"
                                n947 = call "stage_move_axis_relative.vi"("Achse"=w1050, "Schrittweite [µm]"=w1051) -> ("error out"=w1052:errorcluster, "xyz-Position OUT [mm]"=w1053:dbl[])  [unwired: 1 in, 1 out]
                                n948 = local write "Aktuelle xyz-Position [mm]"(w1053) -> ()
                                n949 = local write "Fehler (Ausgang)"(w1052) -> ()
                                }
                                }
                              }
                            }
                          }
                        }
                        n950 = local read "z-Achse"() -> (w912:i32)
                        n951 = local read "# Rasterschritte"() -> (w916:i32[])
                        n952 = Decrement(x=w912) -> (x-1=w920:i32)
                        n953 = local read "Rasterung ON/OFF"() -> (w915:bool)
                        n954 = Increment(x=w911) -> (x+1=w919:i32)
                        n955 = Index Array(array=w916, index=w920) -> (element=w917:i32)
                        n956 = Equal?(x=w917, y=w919) -> (x = y?=w918:bool)
                        n957 = Not(x=w915) -> (.not. x?=w914:bool)
                        n958 = Or(x=w918, y=w914) -> (x .or. y?=w913:bool)
                        "Current z step" <- w911
                      }
                    }
                    frame #1 {
                      n959 = flat-sequence {
                        frame #0 {
                          n960 = local read "z-Achse"() -> (w1054:i32)
                          n961 = local read "Rasterschritt [µm]"() -> (w1057:dbl[])
                          n962 = Decrement(x=w1054) -> (x-1=w1058:i32)
                          n963 = local read "Start xyz-Position [mm]"() -> (w1055:dbl[])
                          n964 = Index Array(array=w1057, index=w1058) -> (element=w1059:dbl)
                          n965 = Not Equal?(x=w1059, y=0.0) -> (x != y?=w1056:bool)
                          n966 = case shown="True" w1056 {
                            tunnel: w1055 -> [_ w1062]
                            tunnel: w1054 -> [_ w1061]
                            frame #0 {
                            }
                            frame #1 {
                              # "Fahre Startposition für z an"
                              n967 = call "stage_move_axis_absolute.vi"("Ziel xyz IN [mm]"=w1062, "Achse"=w1061) -> ("error out"=w1063:errorcluster, "Ziel xyz OUT [mm]"=w1064:dbl[])  [unwired: 1 in, 1 out]
                              n968 = local write "Aktuelle xyz-Position [mm]"(w1064) -> ()
                              n969 = local write "Fehler (Ausgang)"(w1063) -> ()
                            }
                          }
                        }
                        frame #1 {
                          n970 = local read "Rasterschritt [µm]"() -> (w1070:dbl[])
                          n971 = local read "x-Achse"() -> (w1065:i32)
                          n972 = Decrement(x=w1065) -> (x-1=w1069:i32)
                          n973 = Index Array(array=w1070, index=w1069) -> (element=w1068:dbl)
                          n974 = Not Equal?(x=w1068, y=0.0) -> (x != y?=w1066:bool)
                          n975 = case shown="True" w1066 {
                            tunnel: w1068 -> [_ w1073]
                            tunnel: w1065 -> [_ w1071]
                            frame #0 {
                            }
                            frame #1 {
                              # "Fahre nächste Position für x an"
                              n976 = call "stage_move_axis_relative.vi"("Achse"=w1071, "Schrittweite [µm]"=w1073) -> ("error out"=w1074:errorcluster, "xyz-Position OUT [mm]"=w1072:dbl[])  [unwired: 1 in, 1 out]
                              n977 = local write "Aktuelle xyz-Position [mm]"(w1072) -> ()
                              n978 = local write "Fehler (Ausgang)"(w1074) -> ()
                            }
                          }
                        }
                      }
                    }
                  }
                  n979 = local read "# Rasterschritte"() -> (w901:i32[])
                  n980 = local read "x-Achse"() -> (w902:i32)
                  n981 = Decrement(x=w902) -> (x-1=w905:i32)
                  n982 = local read "Rasterung ON/OFF"() -> (w909:bool)
                  n983 = Increment(x=w903) -> (x+1=w906:i32)
                  n984 = Index Array(array=w901, index=w905) -> (element=w908:i32)
                  n985 = Equal?(x=w908, y=w906) -> (x = y?=w907:bool)
                  n986 = Not(x=w909) -> (.not. x?=w910:bool)
                  n987 = Or(x=w907, y=w910) -> (x .or. y?=w904:bool)
                  "Current x step" <- w903
                }
              }
              frame #1 {
                n988 = flat-sequence {
                  frame #0 {
                    # "Zur Ausgangsposition zurückfahren"
                    n989 = local read "Start xyz-Position [mm]"() -> (w1165:dbl[])
                    n990 = local read "Detektionskamera"() -> (w1155:T5)
                    n991 = local read "Buffer Interval"() -> (w1154:u32)
                    n992 = call "camera_create_configuration.vi"("BufferInterval"=w1154, "Session Out 2"=w1155) -> ("Fehler (Ausgang)"=w1153:errorcluster, "Ereignisregistrierung (Referenz)"=w1156:refnum<event-registration>)  [unwired: 1 in, 1 out]
                    n993 = local write "Ereignis: FrameDone?"(w1156) -> ()
                    n994 = local read "x-Achse"() -> (w1162:i32)
                    n995 = call "stage_move_axis_absolute.vi"("error in"=w1153, "Ziel xyz IN [mm]"=w1165, "Achse"=w1162) -> ("error out"=w1158:errorcluster)  [unwired: 2 out]
                    n996 = local read "y-Achse"() -> (w1163:i32)
                    n997 = call "stage_move_axis_absolute.vi"("error in"=w1158, "Ziel xyz IN [mm]"=w1165, "Achse"=w1163) -> ("error out"=w1159:errorcluster)  [unwired: 2 out]
                    n998 = local read "z-Achse"() -> (w1164:i32)
                    n999 = call "stage_move_axis_absolute.vi"("error in"=w1159, "Ziel xyz IN [mm]"=w1165, "Achse"=w1164) -> ("error out"=w1160:errorcluster, "Fertig?"=w1161:bool, "Ziel xyz OUT [mm]"=w1166:dbl[])
                    n1000 = local write "Aktuelle xyz-Position [mm]"(w1166) -> ()
                    n1001 = local write "Fehler (Ausgang)"(w1160) -> ()
                    n1002 = Not(x=w1161) -> (.not. x?=w1157:bool)
                    n1003 = local write "Rasterung ON/OFF"(w1157) -> ()
                    n1004 = local write "Rasterung läuft"(w1157) -> ()
                  }
                }
                n1005 = local read "Daten speichern"() -> (w1075:bool)
                n1006 = local read "LAPD-Daten speichern"() -> (w1084:bool)
                n1007 = local read "2D-Intensitätsverteilung (MCP)"() -> (w1083:dbl[][])
                n1008 = local read "Summierte Helligkeit speichern"() -> (w1085:bool)
                n1009 = case shown="True" w1075 {
                  frame #0 {
                  }
                  frame #1 {
                    n1010 = local read "Rasterschritt [µm]"() -> (w1087:dbl[])
                    n1011 = Divide(x=w1087, y=1000) -> (x/y=w1088:dbl[])
                    n1012 = local read "Start xyz-Position [mm]"() -> (w1090:dbl[])
                    n1013 = local read "# Rasterschritte"() -> (w1091:i32[])
                    n1014 = local read "Save folder"() -> (w1089:string)
                    n1015 = local read "Rasterart"() -> (w1092:T2)
                    n1016 = case shown="\"2D-Scan(xz)\"" w1092 {
                      tunnel: w1091 -> [w1095 w1102 w1114 w1135 w1145]
                      tunnel: w1090 -> [w1093 w1104 w1112 w1136 w1147]
                      tunnel: w1089 -> [w1096 w1105 w1111 w1134 w1148]
                      tunnel: w1088 -> [w1094 w1103 w1113 w1125 w1146]
                      frame #0 {
                        w1101 = 0 ("Index")
                        n1017 = Index Array(array=w1093, index=w1101) -> (element=w1099:dbl)
                        n1018 = Index Array(array=w1094, index=w1101) -> (element=w1097:dbl)
                        n1019 = Index Array(array=w1095, index=w1101) -> (element=w1098:i32)
                        n1020 = call "create_axis_vector_file.vi"("Save folder"=w1096, "Dateiname"="xAchse.dat", "Start"=w1099, "Schrittlänge"=w1097, "# Schritte"=w1098) -> ()  [unwired: 11 in]
                      }
                      frame #1 {
                        w1110 = 2 ("Index")
                        n1021 = Index Array(array=w1104, index=w1110) -> (element=w1108:dbl)
                        n1022 = Index Array(array=w1103, index=w1110) -> (element=w1106:dbl)
                        n1023 = Index Array(array=w1102, index=w1110) -> (element=w1107:i32)
                        n1024 = call "create_axis_vector_file.vi"("Save folder"=w1105, "Dateiname"="xAchse.dat", "Start"=w1108, "Schrittlänge"=w1106, "# Schritte"=w1107) -> ()  [unwired: 11 in]
                      }
                      frame #2 {
                        w1123 = 1 ("Index")
                        w1124 = 0 ("Index")
                        n1025 = Index Array(array=w1112, index #1=w1124, index #2=w1123) -> (element #1=w1120:dbl, element #2=w1117:dbl)
                        n1026 = Index Array(array=w1113, index #1=w1124, index #2=w1123) -> (element #1=w1118:dbl, element #2=w1116:dbl)
                        n1027 = Index Array(array=w1114, index #1=w1124, index #2=w1123) -> (element #1=w1119:i32, element #2=w1115:i32)
                        n1028 = call "create_axis_vector_file.vi"("Save folder"=w1111, "Dateiname"="xAchse.dat", "Start"=w1120, "Schrittlänge"=w1118, "# Schritte"=w1119) -> ()  [unwired: 11 in]
                        n1029 = call "create_axis_vector_file.vi"("Save folder"=w1111, "Dateiname"="yAchse.dat", "Start"=w1117, "Schrittlänge"=w1116, "# Schritte"=w1115) -> ()  [unwired: 11 in]
                      }
                      frame #3 {
                        w1137 = 2 ("Index")
                        w1138 = 1 ("Index")
                        n1030 = Index Array(array=w1136, index #1=w1138, index #2=w1137) -> (element #1=w1131:dbl, element #2=w1128:dbl)
                        n1031 = Index Array(array=w1125, index #1=w1138, index #2=w1137) -> (element #1=w1129:dbl, element #2=w1127:dbl)
                        n1032 = Index Array(array=w1135, index #1=w1138, index #2=w1137) -> (element #1=w1130:i32, element #2=w1126:i32)
                        n1033 = call "create_axis_vector_file.vi"("Save folder"=w1134, "Dateiname"="yAchse.dat", "Start"=w1131, "Schrittlänge"=w1129, "# Schritte"=w1130) -> ()  [unwired: 11 in]
                        n1034 = call "create_axis_vector_file.vi"("Save folder"=w1134, "Dateiname"="xAchse.dat", "Start"=w1128, "Schrittlänge"=w1127, "# Schritte"=w1126) -> ()  [unwired: 11 in]
                      }
                      frame #4 {
                        w1151 = 2 ("Index")
                        w1152 = 0 ("Index")
                        n1035 = Index Array(array=w1147, index #1=w1152, index #2=w1151) -> (element #1=w1144:dbl, element #2=w1139:dbl)
                        n1036 = Index Array(array=w1146, index #1=w1152, index #2=w1151) -> (element #1=w1143:dbl, element #2=w1140:dbl)
                        n1037 = Index Array(array=w1145, index #1=w1152, index #2=w1151) -> (element #1=w1142:i32, element #2=w1141:i32)
                        n1038 = call "create_axis_vector_file.vi"("Save folder"=w1148, "Dateiname"="xAchse.dat", "Start"=w1144, "Schrittlänge"=w1143, "# Schritte"=w1142) -> ()  [unwired: 11 in]
                        n1039 = call "create_axis_vector_file.vi"("Save folder"=w1148, "Dateiname"="yAchse.dat", "Start"=w1139, "Schrittlänge"=w1140, "# Schritte"=w1141) -> ()  [unwired: 11 in]
                      }
                    }
                  }
                }
                n1040 = local read "2D-Intensitätsverteilung (LAPD)"() -> (w1079:dbl[][])
                n1041 = control-ref of="2D-Intensitätsverteilung (MCP)"() -> (w1082:refnum<vi>)
                n1042 = case shown="True" w1084 {
                  frame #0 {
                  }
                  frame #1 {
                    n1043 = local read "Save folder"() -> (w1171:string)
                    n1044 = Concatenate Strings(w1171, "\\" ("String"), "2D_Intensitaetsverteilung_LAPD.dat" ("String")) -> (w1173:string)
                    n1045 = local read "2D-Intensitätsverteilung (LAPD)"() -> (w1169:dbl[][])
                    n1046 = String To Path(string=w1173) -> (path=w1172:path)
                    n1047 = call-poly <vilib>:"Write To Spreadsheet File.vi"("format (%.3f)"="%.;%.5f", "2D data"=w1169, "file path (dialog if empty)"=w1172) -> ()  [unwired: 5 in, 1 out]
                  }
                }
                n1048 = case shown="True" w1085 {
                  frame #0 {
                  }
                  frame #1 {
                    n1049 = local read "Save folder"() -> (w1177:string)
                    n1050 = Concatenate Strings(w1177, "\\" ("String"), "2D_Intensitaetsverteilung_MCP.dat" ("String")) -> (w1175:string)
                    n1051 = local read "2D-Intensitätsverteilung (MCP)"() -> (w1179:dbl[][])
                    n1052 = String To Path(string=w1175) -> (path=w1176:path)
                    n1053 = call-poly <vilib>:"Write To Spreadsheet File.vi"("format (%.3f)"="%.;%8.0f", "2D data"=w1179, "file path (dialog if empty)"=w1176) -> ()  [unwired: 5 in, 1 out]
                  }
                }
                n1054 = Array Max & Min(array=w1083) -> (max value=w1081:dbl, min value=w1080:dbl)  [unwired: 2 out]
                n1055 = control-ref of="2D-Intensitätsverteilung (LAPD)"() -> (w1076:refnum<vi>)
                n1056 = property class="IntGraph (strikt)"(reference=w1082, "ZScale.Maximum"=w1081, "ZScale.Minimum"=w1080) -> ()  [unwired: 1 in, 2 out]
                n1057 = Array Max & Min(array=w1079) -> (max value=w1078:dbl, min value=w1077:dbl)  [unwired: 2 out]
                n1058 = property class="IntGraph (strikt)"(reference=w1076, "ZScale.Maximum"=w1078, "ZScale.Minimum"=w1077) -> ()  [unwired: 1 in, 2 out]
              }
            }
          }
          event #4 {
            n1059 = event-data() -> ("NewVal"=w1182:bool)  [unwired: 1 in, 3 out]
            n1060 = local read "Wellenplatte"() -> (w1183:bool)
            n1061 = local read "Kamera"() -> (w1184:bool)
            n1062 = Compound Arithmetic op=AND(w1184, w1182, w1183) -> (w1181:bool)
            n1063 = case shown="True" w1181 {
              frame #0 {
                n1064 = local write "Leistungs-/Polarisationscan läuft"(FALSE ("Messung läuft")) -> ()
              }
              frame #1 {
                n1065 = stacked-sequence {
                  frame #0 {
                    n1066 = flat-sequence {
                      tunnel: [w1210] -> w1189
                      tunnel: [w1202] -> w1187
                      tunnel: w1189 -> [w1239]
                      tunnel: [w1239] -> w1188
                      tunnel: w1187 -> [w1238]
                      tunnel: [w1238] -> w1186
                      tunnel: w1188 -> [w1246]
                      tunnel: w1186 -> [w1245]
                      frame #0 {
                        n1067 = local read "Hin und Zurück"() -> (w1196:bool)
                        n1068 = local read "# L/2-Schritte"() -> (w1195:i32)
                        n1069 = Get Date/Time In Seconds() -> (seconds since 1Jan1904=w1205:timestamp)
                        n1070 = local read "L/2-Weite [°]"() -> (w1200:dbl)
                        n1071 = local write "Aktueller Messschritt"(0 ("Aktueller Messschritt")) -> ()
                        n1072 = local write "Start time [ms]"(w1205) -> ()
                        n1073 = local read "Leistuns- oder Polarisationsscan"() -> (w1203:u16)
                        n1074 = Divide(x=w1200, y=w1195) -> (x/y=w1199:dbl)
                        n1075 = case shown="False" w1196 {
                          tunnel: w1195 -> [w1222 w1227]
                          tunnel: [w1220 w1225] -> w1190
                          frame #0 {
                            n1076 = local write "Leist/Pol # Schleifen"(i64 1 ("Leist/Pol # Schleifen")) -> ()
                            n1077 = Increment(x=w1222) -> (x+1=w1220:i32)
                          }
                          frame #1 {
                            n1078 = local write "Leist/Pol # Schleifen"(i64 2 ("Leist/Pol # Schleifen")) -> ()
                            n1079 = Increment(x=w1227) -> (x+1=w1223:i32)
                            n1080 = Multiply(x=w1223, y=2) -> (x*y=w1225:i32)
                          }
                        }
                        n1081 = local write "L/2-Schritt [°]"(w1199) -> ()
                        n1082 = local read "L/2-Start [°]"() -> (w1197:dbl)
                        n1083 = case shown="1" w1203 {
                          tunnel: ["Polarisationsscan" ("Subfolder") "Leistungsscan" ("Subfolder")] -> w1202
                          tunnel: [w1228 w1234] -> w1201
                          tunnel: [w1229 w1231] -> w1198
                          tunnel: w1197 -> [w1228 w1233]
                          frame #0 {
                            n1084 = local read "Leistung (iK) [mW]"() -> (w1229:dbl)
                          }
                          frame #1 {
                            n1085 = local read "Max. Leistung (vK) [mW]"() -> (w1232:dbl)
                            n1086 = local read "Polarisation [°]"() -> (w1234:dbl)
                            n1087 = call "calculate_power_in_chamber.vi"("Aktuelle L/2 Position [°]"=w1233, "Eingestellte Polarisation [°]"=w1234, "Max. Leistung (vK) [mW]"=w1232) -> ("Aktuelle Leistung (iK) [mW]"=w1231:dbl)  [unwired: 8 in]
                            n1088 = local write "Leistung (iK) [mW]"(w1231) -> ()
                          }
                        }
                        n1089 = local write "# Messschritte"(w1190) -> ()
                        n1090 = Initialize Array(0.0 ("Element"), w1190) -> (w1194:dbl[])
                        n1091 = Initialize Array(0.0 ("Element"), w1190) -> (w1193:dbl[])
                        n1092 = local write "Vektor Summierte Helligkeit [a.u.]"(w1194) -> ()
                        n1093 = local write "Vektor L/2-Position [°]"(w1193) -> ()
                        n1094 = control-ref of="Shutter time (ms)"() -> (w1219:refnum<vi>)
                        n1095 = property class="Ring (strikt)"(reference=w1219) -> ("RingText.Text"=w1218:string)  [unwired: 1 in, 2 out]
                        n1096 = local read "# Bilder/Messschritt"() -> (w1211:i32)
                        n1097 = local read "Suppressor-Spannung [V]"() -> (w1207:dbl)
                        n1098 = local read "P-Schirm-Spannung [V]"() -> (w1209:dbl)
                        n1099 = local read "MCP-Spannung [V]"() -> (w1208:dbl)
                        n1100 = local read "Tip-Spannung [V]"() -> (w1206:dbl)
                        n1101 = local read "Messlogbuch"() -> (w1216:path)
                        n1102 = call "stage_get_current_xyz.vi"() -> ("Aktuelle xyz-Position OUT [mm]"=w1204:dbl[])  [unwired: 3 in, 1 out]
                        n1103 = Decimal String To Number(string=w1218) -> (number=w1212:i32)  [unwired: 2 in, 1 out]
                        n1104 = local read "Proben-ID"() -> (w1215:string)
                        n1105 = local write "Start xyz-Position [mm]"(w1204) -> ()
                        n1106 = Multiply(x=w1211, y=w1212) -> (x*y=w1213:i32)
                        n1107 = local read "ROI"() -> (w1214:i32[])
                        n1108 = call "create_measure_log_entry.vi"("Messlogbuch-Pfad"=w1216, "Probe"=w1215, "Polarisation [°]"=w1201, "Messart"=w1202, "ROI"=w1214, "Messungen/Messschritt"=w1211, "Maximalleistung (iK) [mW]"=w1198, "Tip-Spannung [V]"=w1206, "Suppressor-Spannung [V]"=w1207, "Zeit/Messschritt [ms]"=w1212, "MCP-Spannung [V]"=w1208, "Zeit/Messung [ms]"=w1213, "Phosphorschirm-Spannung [V]"=w1209, "xyz [mm]"=w1204) -> ("Messung Nr."=w1210:i32)  [unwired: 4 in, 1 out]
                      }
                      frame #1 {
                        n1109 = local read "# L/2-Schritte"() -> (w1237:i32)
                        n1110 = Increment(x=w1237) -> (x+1=w1236:i32)
                        n1111 = local write "# L/2-Schritte"(w1236) -> ()
                      }
                      frame #2 {
                        n1112 = local read "Fehler (Ausgang)"() -> (w1248:errorcluster)
                        n1113 = local read "Summierte Helligkeit speichern"() -> (w1241:bool)
                        n1114 = local read "Einzelbilder speichern"() -> (w1254:bool)
                        n1115 = local read "Gemittelte Bilder speichern"() -> (w1243:bool)
                        n1116 = local read "Day folder"() -> (w1253:string)
                        n1117 = local read "LAPD-Daten speichern"() -> (w1244:bool)
                        n1118 = local read "Einzelbilder speichern"() -> (w1242:bool)
                        n1119 = call "create_save_folder.vi"("Day folder"=w1253, "Measuring number"=w1246, "Measuring folder"=w1245, "error in"=w1248) -> ("Save Folder"=w1252:string, "Error Out"=w1251:errorcluster)  [unwired: 5 in]
                        n1120 = local write "Save folder"(w1252) -> ()
                        n1121 = case shown="True" w1254 {
                          tunnel: w1251 -> [w1257 w1259]
                          tunnel: [w1257 w1258] -> w1250
                          frame #0 {
                          }
                          frame #1 {
                            n1122 = local read "Save folder"() -> (w1262:string)
                            n1123 = Concatenate Strings(w1262, "\\Einzelbilder" ("Subfolder")) -> (w1260:string)
                            n1124 = String To Path(string=w1260) -> (path=w1263:path)
                            n1125 = call <vilib>:"Check if File or Folder Exists.vi"("error in (no error)"=w1259, "path"=w1263) -> ("error out"=w1258:errorcluster, "file or folder exists?"=w1264:bool, "dup path"=w1265:path)  [unwired: 7 in]
                            n1126 = case shown="False" w1264 {
                              tunnel: w1265 -> [w1266 _]
                              frame #0 {
                                n1127 = Create Folder(path (use dialog)=w1266) -> ()  [unwired: 2 in, 3 out]
                              }
                              frame #1 {
                              }
                            }
                          }
                        }
                        n1128 = Compound Arithmetic op=OR(w1243, w1242, w1241, w1244) -> (w1240:bool)
                        n1129 = local write "Daten speichern"(w1240) -> ()
                        n1130 = local read "Gemittelte Bilder speichern"() -> (w1255:bool)
                        n1131 = case shown="True" w1255 {
                          tunnel: w1250 -> [w1267 w1269]
                          tunnel: [w1267 w1268] -> w1249
                          frame #0 {
                          }
                          frame #1 {
                            n1132 = local read "Save folder"() -> (w1273:string)
                            n1133 = Concatenate Strings(w1273, "\\Gemittelte Bilder" ("Subfolder")) -> (w1275:string)
                            n1134 = String To Path(string=w1275) -> (path=w1272:path)
                            n1135 = call <vilib>:"Check if File or Folder Exists.vi"("error in (no error)"=w1269, "path"=w1272) -> ("error out"=w1268:errorcluster, "file or folder exists?"=w1271:bool, "dup path"=w1270:path)  [unwired: 7 in]
                            n1136 = case shown="False" w1271 {
                              tunnel: w1270 -> [w1276 _]
                              frame #0 {
                                n1137 = Create Folder(path (use dialog)=w1276) -> ()  [unwired: 2 in, 3 out]
                              }
                              frame #1 {
                              }
                            }
                          }
                        }
                        n1138 = local read "Kamera"() -> (w1256:bool)
                        n1139 = case shown="True" w1256 {
                          tunnel: [w1277 w1279] -> w1247
                          tunnel: w1249 -> [w1277 w1278]
                          frame #0 {
                          }
                          frame #1 {
                            n1140 = local read "Ereignis: FrameDone?"() -> (w1280:refnum<event-registration>)
                            n1141 = local read "Detektionskamera"() -> (w1281:T5)
                            n1142 = call "camera_release_configuration.vi"("error in"=w1278, "Session In"=w1281, "Ereignisregistrierung (Referenz) 2"=w1280) -> ("error out"=w1279:errorcluster)  [unwired: 1 out]
                          }
                        }
                        n1143 = local write "Fehler (Ausgang)"(w1247) -> ()
                      }
                    }
                  }
                  frame #1 {
                    n1144 = flat-sequence {
                      frame #0 {
                        n1145 = local read "Wellenplatte [°]"() -> (w1292:refnum<k7>)
                        n1146 = local read "L/2-Start [°]"() -> (w1286:dbl)
                        n1147 = invoke class="MG17Motor" method="SetAbsMovePos"(reference=w1292, "lChanID"=0, "fAbsPos"=w1286) -> (reference out=w1290:refnum<k7>, error out=w1287:errorcluster, "lChanID"=w1288:i32)  [unwired: 2 in, 2 out]
                        n1148 = local read "Aktuelle L/2-Position [°]"() -> (w1284:dbl)
                        n1149 = invoke class="MG17Motor" method="MoveAbsolute"(reference=w1290, error in=w1287, "lChanID"=w1288, "bWait"=TRUE) -> (reference out=w1283:refnum<k7>, "lChanID"=w1282:i32)  [unwired: 1 in, 3 out]
                        n1150 = invoke class="MG17Motor" method="GetPosition"(reference=w1283, "lChanID"=w1282, "pfPosition"=w1284) -> ("pfPosition"=w1285:sgl)  [unwired: 2 in, 4 out]
                        n1151 = local write "Aktuelle L/2-Position [°]"(w1285) -> ()
                      }
                      frame #1 {
                        n1152 = local write "Leistungs-/Polarisationscan läuft"(TRUE ("Messung läuft")) -> ()
                      }
                    }
                  }
                }
              }
            }
          }
          event #5 {
            n1153 = event-data() -> ("NewVal"=w1296:bool)  [unwired: 1 in]
            n1154 = local read "HV-Steuerung"() -> (w1294:bool)
            n1155 = local read "Kamera"() -> (w1297:bool)
            n1156 = Compound Arithmetic op=AND(w1297, w1296, w1294) -> (w1295:bool)
            n1157 = case shown="True" w1295 {
              frame #0 {
                n1158 = local write "Spannungsscan läuft"(FALSE ("Messung läuft")) -> ()
              }
              frame #1 {
                n1159 = stacked-sequence {
                  frame #0 {
                    n1160 = flat-sequence {
                      tunnel: [w1312] -> w1299
                      tunnel: w1299 -> [w1333]
                      frame #0 {
                        n1161 = Get Date/Time In Seconds() -> (seconds since 1Jan1904=w1300:timestamp)
                        n1162 = local write "Aktueller Messschritt"(0 ("Aktueller Messschritt")) -> ()
                        n1163 = local write "Start time [ms]"(w1300) -> ()
                        n1164 = local read "# Spannungsschritte"() -> (w1321:i32[])
                        n1165 = local read "Spannungsweite [V]"() -> (w1320:dbl[])
                        n1166 = control-ref of="Shutter time (ms)"() -> (w1325:refnum<vi>)
                        n1167 = property class="Ring (strikt)"(reference=w1325) -> ("RingText.Text"=w1324:string)  [unwired: 1 in, 2 out]
                        n1168 = local read "Suppressor-Spannung [V]"() -> (w1302:dbl)
                        n1169 = local read "# Bilder/Messschritt"() -> (w1318:i32)
                        n1170 = local read "Spannungsstart [V]"() -> (w1306:dbl[])
                        n1171 = local read "Tip-Spannung [V]"() -> (w1303:dbl)
                        n1172 = Divide(x=w1320, y=w1321) -> (x/y=w1322:dbl[])
                        n1173 = Decimal String To Number(string=w1324) -> (number=w1307:i32)  [unwired: 2 in, 1 out]
                        n1174 = local read "P-Schirm-Spannung [V]"() -> (w1310:dbl)
                        n1175 = local read "MCP-Spannung [V]"() -> (w1309:dbl)
                        n1176 = local read "Leistung (iK) [mW]"() -> (w1308:dbl)
                        n1177 = local read "Polarisation [°]"() -> (w1315:dbl)
                        n1178 = local read "Messlogbuch"() -> (w1317:path)
                        n1179 = local read "Proben-ID"() -> (w1316:string)
                        n1180 = local write "Spannungsschritt [V]"(w1322) -> ()
                        n1181 = Multiply(x=w1318, y=w1307) -> (x*y=w1319:i32)
                        n1182 = Replace Array Subset(array=w1306, new element #1=w1303, index #1=0 ("Index"), new element #2=w1302, index #2=1 ("Index")) -> (w1301:dbl[])
                        n1183 = local read "ROI"() -> (w1313:i32[])
                        n1184 = local write "Aktuelle Spannung [V]"(w1301) -> ()
                        n1185 = local write "Spannungsstart [V]"(w1301) -> ()
                        n1186 = call "stage_get_current_xyz.vi"() -> ("Aktuelle xyz-Position OUT [mm]"=w1311:dbl[])  [unwired: 3 in, 1 out]
                        n1187 = call "create_measure_log_entry.vi"("Messlogbuch-Pfad"=w1317, "Probe"=w1316, "Polarisation [°]"=w1315, "Messart"="Spannungsscan", "ROI"=w1313, "Messungen/Messschritt"=w1318, "Maximalleistung (iK) [mW]"=w1308, "Tip-Spannung [V]"=w1303, "Suppressor-Spannung [V]"=w1302, "Zeit/Messschritt [ms]"=w1307, "MCP-Spannung [V]"=w1309, "Zeit/Messung [ms]"=w1319, "Phosphorschirm-Spannung [V]"=w1310, "xyz [mm]"=w1311) -> ("Messung Nr."=w1312:i32)  [unwired: 4 in, 1 out]
                      }
                      frame #1 {
                        n1188 = local read "Fehler (Ausgang)"() -> (w1334:errorcluster)
                        n1189 = local read "Day folder"() -> (w1339:string)
                        n1190 = local read "Einzelbilder speichern"() -> (w1341:bool)
                        n1191 = local read "# Spannungsschritte"() -> (w1348:i32[])
                        n1192 = local read "Summierte Helligkeit speichern"() -> (w1329:bool)
                        n1193 = local read "Gemittelte Bilder speichern"() -> (w1327:bool)
                        n1194 = call "create_save_folder.vi"("Day folder"=w1339, "Measuring number"=w1333, "Measuring folder"="Spannungsscan" ("Subfolder"), "error in"=w1334) -> ("Save Folder"=w1338:string, "Error Out"=w1337:errorcluster)  [unwired: 5 in]
                        n1195 = local read "LAPD-Daten speichern"() -> (w1326:bool)
                        n1196 = local read "Einzelbilder speichern"() -> (w1328:bool)
                        n1197 = local write "Save folder"(w1338) -> ()
                        n1198 = case shown="True" w1341 {
                          tunnel: w1337 -> [w1349 w1351]
                          tunnel: [w1349 w1350] -> w1336
                          frame #0 {
                          }
                          frame #1 {
                            n1199 = local read "Save folder"() -> (w1354:string)
                            n1200 = Concatenate Strings(w1354, "\\Einzelbilder" ("Subfolder")) -> (w1352:string)
                            n1201 = String To Path(string=w1352) -> (path=w1355:path)
                            n1202 = call <vilib>:"Check if File or Folder Exists.vi"("error in (no error)"=w1351, "path"=w1355) -> ("error out"=w1350:errorcluster, "file or folder exists?"=w1356:bool, "dup path"=w1357:path)  [unwired: 7 in]
                            n1203 = case shown="False" w1356 {
                              tunnel: w1357 -> [w1358 _]
                              frame #0 {
                                n1204 = Create Folder(path (use dialog)=w1358) -> ()  [unwired: 2 in, 3 out]
                              }
                              frame #1 {
                              }
                            }
                          }
                        }
                        n1205 = Index Array(array=w1348, index #1=0 ("Index"), index #2=1 ("Index")) -> (element #1=w1345:i32, element #2=w1344:i32)
                        n1206 = Multiply(x=w1345, y=w1344) -> (x*y=w1331:i32)
                        n1207 = Compound Arithmetic op=OR(w1327, w1328, w1329, w1326) -> (w1330:bool)
                        n1208 = local write "Daten speichern"(w1330) -> ()
                        n1209 = local write "# Messschritte"(w1331) -> ()
                        n1210 = local read "Gemittelte Bilder speichern"() -> (w1342:bool)
                        n1211 = case shown="True" w1342 {
                          tunnel: w1336 -> [w1359 w1361]
                          tunnel: [w1359 w1360] -> w1335
                          frame #0 {
                          }
                          frame #1 {
                            n1212 = local read "Save folder"() -> (w1365:string)
                            n1213 = Concatenate Strings(w1365, "\\Gemittelte Bilder" ("Subfolder")) -> (w1367:string)
                            n1214 = String To Path(string=w1367) -> (path=w1364:path)
                            n1215 = call <vilib>:"Check if File or Folder Exists.vi"("error in (no error)"=w1361, "path"=w1364) -> ("error out"=w1360:errorcluster, "file or folder exists?"=w1363:bool, "dup path"=w1362:path)  [unwired: 7 in]
                            n1216 = case shown="False" w1363 {
                              tunnel: w1362 -> [w1368 _]
                              frame #0 {
                                n1217 = Create Folder(path (use dialog)=w1368) -> ()  [unwired: 2 in, 3 out]
                              }
                              frame #1 {
                              }
                            }
                          }
                        }
                        n1218 = local read "Kamera"() -> (w1343:bool)
                        n1219 = case shown="True" w1343 {
                          tunnel: [w1369 w1371] -> w1332
                          tunnel: w1335 -> [w1369 w1370]
                          frame #0 {
                          }
                          frame #1 {
                            n1220 = local read "Ereignis: FrameDone?"() -> (w1372:refnum<event-registration>)
                            n1221 = local read "Detektionskamera"() -> (w1373:T5)
                            n1222 = call "camera_release_configuration.vi"("error in"=w1370, "Session In"=w1373, "Ereignisregistrierung (Referenz) 2"=w1372) -> ("error out"=w1371:errorcluster)  [unwired: 1 out]
                          }
                        }
                        n1223 = local write "Fehler (Ausgang)"(w1332) -> ()
                      }
                    }
                  }
                  frame #1 {
                    n1224 = flat-sequence {
                      frame #0 {
                        w1379 = 1 ("Index")
                        w1380 = 0 ("Index")
                        n1225 = local read "# Spannungsschritte"() -> (w1390:i32[])
                        n1226 = local read "Spannungsstart [V]"() -> (w1375:dbl[])
                        n1227 = local read "Spannungsschritt [V]"() -> (w1378:dbl[])
                        n1228 = Index Array(array=w1390, index #1=w1380, index #2=w1379) -> (element #1=w1388:i32, element #2=w1389:i32)
                        n1229 = Index Array(array=w1375, index #1=w1380, index #2=w1379) -> (element #1=w1377:dbl, element #2=w1376:dbl)
                        n1230 = control-ref of="2D-Intensitätsverteilung (MCP)"() -> (w1374:refnum<vi>)
                        n1231 = Index Array(array=w1378, index #1=w1380, index #2=w1379) -> (element #1=w1382:dbl, element #2=w1381:dbl)
                        n1232 = Initialize Array(0.0 ("y"), w1388, w1389) -> (w1386:dbl[][])
                        n1233 = local write "2D-Intensitätsverteilung (MCP)"(w1386) -> ()
                        n1234 = property class="IntGraph (strikt)"(reference=w1374, "XScale.Offset"=w1377, "XScale.Multiplier"=w1382, "YScale.Offset"=w1376, "YScale.Multiplier"=w1381, "XScale.MinorInc"=w1382, "YScale.MinorInc"=w1381, "XScale.NameLbl.Text"="Tip-Spannung [V]" ("Y-Achse.Namensbeschriftung.Text"), "YScale.NameLbl.Text"="Suppressor-Spannung [V]" ("X-Achse.Namensbeschriftung.Text")) -> (error out=w1385:errorcluster)  [unwired: 1 in, 1 out]
                        n1235 = local write "Fehler (Ausgang)"(w1385) -> ()
                      }
                      frame #1 {
                        n1236 = local write "Spannungsscan läuft"(TRUE ("Messung läuft")) -> ()
                      }
                    }
                  }
                }
              }
            }
          }
          event #6 {
            n1237 = event-data() -> ("NewVal"=w1394:bool)  [unwired: 1 in]
            n1238 = local read "HV-Steuerung"() -> (w1392:bool)
            n1239 = local read "Kamera"() -> (w1395:bool)
            n1240 = Compound Arithmetic op=AND(w1395, w1394, w1392) -> (w1393:bool)
            n1241 = case shown="True" w1393 {
              frame #0 {
                n1242 = local write "x-U-Scan läuft"(FALSE ("Messung läuft")) -> ()
              }
              frame #1 {
                n1243 = stacked-sequence {
                  frame #0 {
                    # "Falls der gewählte Startwert für den Scan und der Startwert zur Berechnung der Ausgleichslage nicht identisch sind muss ein korrigierter Wert für die Raum-Koordinate 2 angefahren werden"
                    n1244 = local read "x-U-Scan (Ausgleichslage) Steigung"() -> (w1398:dbl)
                    n1245 = Not Equal?(x=w1398, y=0.0) -> (x != y?=w1399:bool)
                    n1246 = case shown="True" w1399 {
                      frame #0 {
                      }
                      frame #1 {
                        n1247 = flat-sequence {
                          tunnel: [w1402] -> w1400
                          tunnel: w1400 -> [w1415]
                          frame #0 {
                            n1248 = local read "x-U-Scan (Ausgleichslage) xy-Start [mm]"() -> (w1413:dbl[])
                            n1249 = local read "Raum-Koordinate 2 (Lagenausgleich)"() -> (w1402:enum16{"x-Achse", "y-Achse", "z-Achse"})
                            n1250 = local read "Raum-Koordinate 1"() -> (w1411:enum16{"x-Achse", "y-Achse", "z-Achse"})
                            n1251 = call "stage_get_current_xyz.vi"() -> ("Aktuelle xyz-Position OUT [mm]"=w1404:dbl[])  [unwired: 3 in, 1 out]
                            n1252 = local read "x-U-Scan (Ausgleichslage) Steigung"() -> (w1408:dbl)
                            n1253 = Index Array(array=w1404, index=w1411) -> (element=w1410:dbl)
                            n1254 = Index Array(array=w1413, index #1=w1411, index #2=w1402) -> (element #1=w1412:dbl, element #2=w1405:dbl)
                            n1255 = local write "x-U-Scan x-Startposition [mm]"(w1410) -> ()
                            n1256 = Subtract(x=w1410, y=w1412) -> (x-y=w1409:dbl)
                            n1257 = Multiply(x=w1409, y=w1408) -> (x*y=w1406:dbl)
                            n1258 = Increment(x=w1402) -> (x+1=w1407:enum16{"x-Achse", "y-Achse", "z-Achse"})
                            n1259 = Add(x=w1406, y=w1405) -> (x+y=w1401:dbl)
                            n1260 = Replace Array Subset(array=w1404, new element=w1401, index=w1402) -> (w1403:dbl[])
                            n1261 = call "stage_move_axis_absolute.vi"("Ziel xyz IN [mm]"=w1403, "Achse"=w1407) -> ()  [unwired: 1 in, 3 out]
                          }
                          frame #1 {
                            n1262 = call "stage_get_current_xyz.vi"() -> ("Aktuelle xyz-Position OUT [mm]"=w1416:dbl[])  [unwired: 3 in, 1 out]
                            n1263 = local write "Start xyz-Position [mm]"(w1416) -> ()
                            n1264 = Index Array(array=w1416, index=w1415) -> (element=w1414:dbl)
                            n1265 = local write "x-U-Scan y-Startposition [mm]"(w1414) -> ()
                          }
                        }
                      }
                    }
                  }
                  frame #1 {
                    n1266 = flat-sequence {
                      tunnel: [w1432] -> w1417
                      tunnel: w1417 -> [w1463]
                      frame #0 {
                        n1267 = Get Date/Time In Seconds() -> (seconds since 1Jan1904=w1423:timestamp)
                        n1268 = local write "Aktueller Messschritt"(0 ("Aktueller Messschritt")) -> ()
                        n1269 = local write "Start time [ms]"(w1423) -> ()
                        n1270 = local read "Spannungs-Koordinate"() -> (w1442:enum16{"Tip-Spannung", "Suppressor-Spannung"})
                        n1271 = local read "# x-U-Scan Spannungsschritte"() -> (w1447:i32)
                        n1272 = local read "x-U-Scan x-Rasterweite [µm]"() -> (w1445:dbl)
                        n1273 = local read "x-U-Scan Spannungsweite [V]"() -> (w1446:dbl)
                        n1274 = local read "# x-U-Scan x-Rasterschritte"() -> (w1444:i32)
                        n1275 = control-ref of="Shutter time (ms)"() -> (w1451:refnum<vi>)
                        n1276 = case shown="\"Suppressor-Spannung\", Voreinstellung" w1442 {
                          tunnel: [refnum<k21> "Dev0/Ao1" ("Spannungskanal") refnum<k21> "Dev0/Ao0" ("Spannungskanal")] -> w1441
                          tunnel: [w1452 w1454] -> w1424
                          frame #0 {
                            n1277 = local read "Tip-Spannung [V]"() -> (w1452:dbl)
                          }
                          frame #1 {
                            n1278 = local read "Suppressor-Spannung [V]"() -> (w1454:dbl)
                          }
                        }
                        n1279 = property class="Ring (strikt)"(reference=w1451) -> ("RingText.Text"=w1450:string)  [unwired: 1 in, 2 out]
                        n1280 = Divide(x=w1446, y=w1447) -> (x/y=w1448:dbl)
                        n1281 = Divide(x=w1445, y=w1444) -> (x/y=w1443:dbl)
                        n1282 = local read "# Bilder/Messschritt"() -> (w1433:i32)
                        n1283 = local write "x-U-Scan Spannungsschritt [V]"(w1448) -> ()
                        n1284 = local write "x-U-Scan x-Rasterschritt [µm]"(w1443) -> ()
                        n1285 = Decimal String To Number(string=w1450) -> (number=w1434:i32)  [unwired: 2 in, 1 out]
                        n1286 = local read "Suppressor-Spannung [V]"() -> (w1428:dbl)
                        n1287 = local read "P-Schirm-Spannung [V]"() -> (w1431:dbl)
                        n1288 = local read "MCP-Spannung [V]"() -> (w1430:dbl)
                        n1289 = local read "Leistung (iK) [mW]"() -> (w1429:dbl)
                        n1290 = local read "Tip-Spannung [V]"() -> (w1427:dbl)
                        n1291 = local read "Polarisation [°]"() -> (w1438:dbl)
                        n1292 = local read "Messlogbuch"() -> (w1440:path)
                        n1293 = local read "Proben-ID"() -> (w1439:string)
                        n1294 = Multiply(x=w1433, y=w1434) -> (x*y=w1435:i32)
                        n1295 = local read "Raum-Koordinate 2 (Lagenausgleich)"() -> (w1420:enum16{"x-Achse", "y-Achse", "z-Achse"})
                        n1296 = local read "ROI"() -> (w1436:i32[])
                        n1297 = local read "Raum-Koordinate 1"() -> (w1421:enum16{"x-Achse", "y-Achse", "z-Achse"})
                        n1298 = call "stage_get_current_xyz.vi"() -> ("Aktuelle xyz-Position OUT [mm]"=w1422:dbl[])  [unwired: 3 in, 1 out]
                        n1299 = call "create_measure_log_entry.vi"("Messlogbuch-Pfad"=w1440, "Probe"=w1439, "Polarisation [°]"=w1438, "Messart"="x-U-Scan", "ROI"=w1436, "Messungen/Messschritt"=w1433, "Maximalleistung (iK) [mW]"=w1429, "Tip-Spannung [V]"=w1427, "Suppressor-Spannung [V]"=w1428, "Zeit/Messschritt [ms]"=w1434, "MCP-Spannung [V]"=w1430, "Zeit/Messung [ms]"=w1435, "Phosphorschirm-Spannung [V]"=w1431, "xyz [mm]"=w1422) -> ("Messung Nr."=w1432:i32)  [unwired: 4 in, 1 out]
                        n1300 = local write "Start xyz-Position [mm]"(w1422) -> ()
                        n1301 = Index Array(array=w1422, index #1=w1421, index #2=w1420) -> (element #1=w1418:dbl, element #2=w1419:dbl)
                        n1302 = Add(x=w1421, y=1) -> (x+y=w1425:i32)
                        n1303 = local write "x-U-Scan aktuelle y-Position [mm]"(w1419) -> ()
                        n1304 = local write "x-U-Scan aktuelle x-Position [mm]"(w1418) -> ()
                        n1305 = local write "x-U-Scan y-Startposition [mm]"(w1419) -> ()
                        n1306 = local write "x-U-Scan x-Startposition [mm]"(w1418) -> ()
                        n1307 = local write "x-U-Scan aktuelle Spannung [V]"(w1424) -> ()
                        n1308 = local write "x-U-Scan Spannungsstart [V]"(w1424) -> ()
                        n1309 = local write "Spannungskanal"(w1441) -> ()
                        n1310 = local write "Achs-ID"(w1425) -> ()
                      }
                      frame #1 {
                        n1311 = local read "Fehler (Ausgang)"() -> (w1466:errorcluster)
                        n1312 = local read "Day folder"() -> (w1471:string)
                        n1313 = local read "Summierte Helligkeit speichern"() -> (w1459:bool)
                        n1314 = local read "# x-U-Scan Spannungsschritte"() -> (w1462:i32)
                        n1315 = local read "# x-U-Scan x-Rasterschritte"() -> (w1461:i32)
                        n1316 = local read "Gemittelte Bilder speichern"() -> (w1457:bool)
                        n1317 = local read "LAPD-Daten speichern"() -> (w1456:bool)
                        n1318 = local read "Einzelbilder speichern"() -> (w1458:bool)
                        n1319 = local read "Einzelbilder speichern"() -> (w1473:bool)
                        n1320 = call "create_save_folder.vi"("Day folder"=w1471, "Measuring number"=w1463, "Measuring folder"="x-U-Scan" ("Subfolder"), "error in"=w1466) -> ("Save Folder"=w1470:string, "Error Out"=w1469:errorcluster)  [unwired: 5 in]
                        n1321 = Multiply(x=w1462, y=w1461) -> (x*y=w1464:i32)
                        n1322 = local write "Save folder"(w1470) -> ()
                        n1323 = case shown="True" w1473 {
                          tunnel: w1469 -> [w1476 w1478]
                          tunnel: [w1476 w1477] -> w1468
                          frame #0 {
                          }
                          frame #1 {
                            n1324 = local read "Save folder"() -> (w1481:string)
                            n1325 = Concatenate Strings(w1481, "\\Einzelbilder" ("Subfolder")) -> (w1479:string)
                            n1326 = String To Path(string=w1479) -> (path=w1482:path)
                            n1327 = call <vilib>:"Check if File or Folder Exists.vi"("error in (no error)"=w1478, "path"=w1482) -> ("error out"=w1477:errorcluster, "file or folder exists?"=w1483:bool, "dup path"=w1484:path)  [unwired: 7 in]
                            n1328 = case shown="False" w1483 {
                              tunnel: w1484 -> [w1485 _]
                              frame #0 {
                                n1329 = Create Folder(path (use dialog)=w1485) -> ()  [unwired: 2 in, 3 out]
                              }
                              frame #1 {
                              }
                            }
                          }
                        }
                        n1330 = Compound Arithmetic op=OR(w1457, w1458, w1459, w1456) -> (w1460:bool)
                        n1331 = local write "Daten speichern"(w1460) -> ()
                        n1332 = local write "# Messschritte"(w1464) -> ()
                        n1333 = local read "Gemittelte Bilder speichern"() -> (w1474:bool)
                        n1334 = case shown="True" w1474 {
                          tunnel: w1468 -> [w1486 w1488]
                          tunnel: [w1486 w1487] -> w1467
                          frame #0 {
                          }
                          frame #1 {
                            n1335 = local read "Save folder"() -> (w1492:string)
                            n1336 = Concatenate Strings(w1492, "\\Gemittelte Bilder" ("Subfolder")) -> (w1494:string)
                            n1337 = String To Path(string=w1494) -> (path=w1491:path)
                            n1338 = call <vilib>:"Check if File or Folder Exists.vi"("error in (no error)"=w1488, "path"=w1491) -> ("error out"=w1487:errorcluster, "file or folder exists?"=w1490:bool, "dup path"=w1489:path)  [unwired: 7 in]
                            n1339 = case shown="False" w1490 {
                              tunnel: w1489 -> [w1495 _]
                              frame #0 {
                                n1340 = Create Folder(path (use dialog)=w1495) -> ()  [unwired: 2 in, 3 out]
                              }
                              frame #1 {
                              }
                            }
                          }
                        }
                        n1341 = local read "Kamera"() -> (w1475:bool)
                        n1342 = case shown="True" w1475 {
                          tunnel: [w1496 w1498] -> w1465
                          tunnel: w1467 -> [w1496 w1497]
                          frame #0 {
                          }
                          frame #1 {
                            n1343 = local read "Ereignis: FrameDone?"() -> (w1499:refnum<event-registration>)
                            n1344 = local read "Detektionskamera"() -> (w1500:T5)
                            n1345 = call "camera_release_configuration.vi"("error in"=w1497, "Session In"=w1500, "Ereignisregistrierung (Referenz) 2"=w1499) -> ("error out"=w1498:errorcluster)  [unwired: 1 out]
                          }
                        }
                        n1346 = local write "Fehler (Ausgang)"(w1465) -> ()
                      }
                    }
                  }
                  frame #2 {
                    n1347 = flat-sequence {
                      frame #0 {
                        n1348 = local read "# x-U-Scan Spannungsschritte"() -> (w1509:i32)
                        n1349 = local read "x-U-Scan x-Rasterschritt [µm]"() -> (w1502:dbl)
                        n1350 = local read "# x-U-Scan x-Rasterschritte"() -> (w1508:i32)
                        n1351 = Initialize Array(0.0 ("y"), w1508, w1509) -> (w1513:dbl[][])
                        n1352 = Divide(x=w1502, y=1000.0) -> (x/y=w1503:dbl)
                        n1353 = local write "2D-Intensitätsverteilung (MCP)"(w1513) -> ()
                        n1354 = local read "x-U-Scan Spannungsschritt [V]"() -> (w1505:dbl)
                        n1355 = local read "x-U-Scan x-Startposition [mm]"() -> (w1506:dbl)
                        n1356 = local read "x-U-Scan Spannungsstart [V]"() -> (w1507:dbl)
                        n1357 = control-ref of="2D-Intensitätsverteilung (MCP)"() -> (w1504:refnum<vi>)
                        n1358 = property class="IntGraph (strikt)"(reference=w1504, "XScale.Offset"=w1506, "XScale.Multiplier"=w1503, "YScale.Offset"=w1507, "YScale.Multiplier"=w1505, "XScale.MinorInc"=w1503, "YScale.MinorInc"=w1505, "XScale.NameLbl.Text"="Position [mm]" ("Y-Achse.Namensbeschriftung.Text"), "YScale.NameLbl.Text"="Spannung [V]" ("X-Achse.Namensbeschriftung.Text")) -> (error out=w1512:errorcluster)  [unwired: 1 in, 1 out]
                        n1359 = local write "Fehler (Ausgang)"(w1512) -> ()
                      }
                      frame #1 {
                        n1360 = local write "x-U-Scan läuft"(TRUE ("Messung läuft")) -> ()
                      }
                    }
                  }
                }
              }
            }
          }
          event #7 {
            n1361 = event-data() -> ("NewVal"=w1516:bool)  [unwired: 1 in]
            n1362 = case shown="True" w1516 {
              frame #0 {
              }
              frame #1 {
                n1363 = flat-sequence {
                  tunnel: [w1521] -> w1517
                  tunnel: w1517 -> [w1538]
                  frame #0 {
                    n1364 = local write "Ausgleichslage Start festlegen"(FALSE ("Ausgleichslage Ende festlegen")) -> ()
                    n1365 = local read "Raum-Koordinate 2 (Lagenausgleich)"() -> (w1519:enum16{"x-Achse", "y-Achse", "z-Achse"})
                    n1366 = local read "Raum-Koordinate 1"() -> (w1520:enum16{"x-Achse", "y-Achse", "z-Achse"})
                    n1367 = local read "x-U-Scan (Ausgleichslage) xy-Start [mm]"() -> (w1522:dbl[])
                    n1368 = call "stage_get_current_xyz.vi"() -> ("Aktuelle xyz-Position OUT [mm]"=w1527:dbl[])  [unwired: 3 in, 1 out]
                    n1369 = Index Array(array=w1527, index #1=w1520, index #2=w1519) -> (element #1=w1524:dbl, element #2=w1523:dbl)
                    n1370 = Replace Array Subset(array=w1522, new element #1=w1524, index #1=0 ("Index"), new element #2=w1523, index #2=1 ("Index")) -> (w1521:dbl[])
                    n1371 = local write "x-U-Scan (Ausgleichslage) xy-Start [mm]"(w1521) -> ()
                  }
                  frame #1 {
                    n1372 = local read "x-U-Scan (Ausgleichslage) xy-End [mm]"() -> (w1539:dbl[])
                    n1373 = Index Array(array=w1538, index #1=0 ("Index"), index #2=1 ("Index")) -> (element #1=w1530:dbl, element #2=w1533:dbl)
                    n1374 = Index Array(array=w1539, index #1=0 ("Index"), index #2=1 ("Index")) -> (element #1=w1529:dbl, element #2=w1532:dbl)
                    n1375 = Not Equal?(x=w1530, y=w1529) -> (x != y?=w1528:bool)
                    n1376 = case shown="True" w1528 {
                      tunnel: w1533 -> [_ w1545]
                      tunnel: w1532 -> [_ w1544]
                      tunnel: w1529 -> [_ w1543]
                      tunnel: w1530 -> [_ w1542]
                      tunnel: [0.0 w1541] -> w1531
                      frame #0 {
                      }
                      frame #1 {
                        n1377 = Subtract(x=w1545, y=w1544) -> (x-y=w1547:dbl)
                        n1378 = Subtract(x=w1542, y=w1543) -> (x-y=w1546:dbl)
                        n1379 = Divide(x=w1547, y=w1546) -> (x/y=w1541:dbl)
                      }
                    }
                    n1380 = local write "x-U-Scan (Ausgleichslage) Steigung"(w1531) -> ()
                  }
                }
              }
            }
          }
          event #8 {
            n1381 = event-data() -> ("NewVal"=w1548:bool)  [unwired: 1 in]
            n1382 = case shown="True" w1548 {
              frame #0 {
              }
              frame #1 {
                n1383 = flat-sequence {
                  tunnel: [w1553] -> w1549
                  tunnel: w1549 -> [w1570]
                  frame #0 {
                    n1384 = local write "Ausgleichslage Ende festlegen"(FALSE ("Ausgleichslage Ende festlegen")) -> ()
                    n1385 = local read "Raum-Koordinate 2 (Lagenausgleich)"() -> (w1551:enum16{"x-Achse", "y-Achse", "z-Achse"})
                    n1386 = local read "Raum-Koordinate 1"() -> (w1552:enum16{"x-Achse", "y-Achse", "z-Achse"})
                    n1387 = local read "x-U-Scan (Ausgleichslage) xy-End [mm]"() -> (w1554:dbl[])
                    n1388 = call "stage_get_current_xyz.vi"() -> ("Aktuelle xyz-Position OUT [mm]"=w1559:dbl[])  [unwired: 3 in, 1 out]
                    n1389 = Index Array(array=w1559, index #1=w1552, index #2=w1551) -> (element #1=w1556:dbl, element #2=w1555:dbl)
                    n1390 = Replace Array Subset(array=w1554, new element #1=w1556, index #1=0 ("Index"), new element #2=w1555, index #2=1 ("Index")) -> (w1553:dbl[])
                    n1391 = local write "x-U-Scan (Ausgleichslage) xy-End [mm]"(w1553) -> ()
                  }
                  frame #1 {
                    n1392 = local read "x-U-Scan (Ausgleichslage) xy-Start [mm]"() -> (w1571:dbl[])
                    n1393 = Index Array(array=w1570, index #1=0 ("Index"), index #2=1 ("Index")) -> (element #1=w1562:dbl, element #2=w1565:dbl)
                    n1394 = Index Array(array=w1571, index #1=0 ("Index"), index #2=1 ("Index")) -> (element #1=w1561:dbl, element #2=w1564:dbl)
                    n1395 = Not Equal?(x=w1562, y=w1561) -> (x != y?=w1560:bool)
                    n1396 = case shown="True" w1560 {
                      tunnel: w1565 -> [_ w1577]
                      tunnel: w1564 -> [_ w1576]
                      tunnel: w1561 -> [_ w1575]
                      tunnel: w1562 -> [_ w1574]
                      tunnel: [0.0 w1573] -> w1563
                      frame #0 {
                      }
                      frame #1 {
                        n1397 = Subtract(x=w1577, y=w1576) -> (x-y=w1579:dbl)
                        n1398 = Subtract(x=w1574, y=w1575) -> (x-y=w1578:dbl)
                        n1399 = Divide(x=w1579, y=w1578) -> (x/y=w1573:dbl)
                      }
                    }
                    n1400 = local write "x-U-Scan (Ausgleichslage) Steigung"(w1563) -> ()
                  }
                }
              }
            }
          }
          event #9 {
            n1401 = event-data() -> ("NewVal"=w1580:bool)  [unwired: 1 in]
            n1402 = case shown="True" w1580 {
              frame #0 {
              }
              frame #1 {
                n1403 = control-ref of="Shutter time (ms)"() -> (w1616:refnum<vi>)
                n1404 = property class="Ring (strikt)"(reference=w1616) -> ("RingText.Text"=w1598:string)  [unwired: 1 in, 2 out]
                n1405 = local read "# Bilder/Messschritt"() -> (w1594:i32)
                n1406 = local read "Suppressor-Spannung [V]"() -> (w1581:dbl)
                n1407 = local read "P-Schirm-Spannung [V]"() -> (w1586:dbl)
                n1408 = local read "MCP-Spannung [V]"() -> (w1585:dbl)
                n1409 = local read "Leistung (iK) [mW]"() -> (w1584:dbl)
                n1410 = local read "Tip-Spannung [V]"() -> (w1582:dbl)
                n1411 = Decimal String To Number(string=w1598) -> (number=w1593:i32)  [unwired: 2 in, 1 out]
                n1412 = local read "Polarisation [°]"() -> (w1589:dbl)
                n1413 = local read "Messlogbuch"() -> (w1591:path)
                n1414 = local read "Proben-ID"() -> (w1590:string)
                n1415 = Concatenate Strings(w1598, "ms_" ("String")) -> (w1597:string)
                n1416 = Multiply(x=w1594, y=w1593) -> (x*y=w1592:i32)
                n1417 = local read "Sequenz Ordner"() -> (w1614:string)
                n1418 = local read "ROI"() -> (w1587:i32[])
                n1419 = local read "Day folder"() -> (w1615:string)
                n1420 = call "stage_get_current_xyz.vi"() -> ("Aktuelle xyz-Position OUT [mm]"=w1595:dbl[])  [unwired: 3 in, 1 out]
                n1421 = call "create_measure_log_entry.vi"("Messlogbuch-Pfad"=w1591, "Probe"=w1590, "Polarisation [°]"=w1589, "Messart"="Referenzbilder", "ROI"=w1587, "Messungen/Messschritt"=w1594, "Maximalleistung (iK) [mW]"=w1584, "Tip-Spannung [V]"=w1582, "Suppressor-Spannung [V]"=w1581, "Zeit/Messschritt [ms]"=w1593, "MCP-Spannung [V]"=w1585, "Zeit/Messung [ms]"=w1592, "Phosphorschirm-Spannung [V]"=w1586, "xyz [mm]"=w1595) -> ("Messung Nr."=w1583:i32)  [unwired: 4 in, 1 out]
                n1422 = call "create_save_folder.vi"("Day folder"=w1615, "Measuring number"=w1583, "Measuring folder"=w1614) -> ("Save Folder"=w1601:string, "Error Out"=w1612:errorcluster)  [unwired: 6 in]
                n1423 = local write "Save folder"(w1601) -> ()
                n1424 = local read "Kamera"() -> (w1613:bool)
                n1425 = case shown="True" w1613 {
                  tunnel: [w1618 w1621] -> w1604
                  tunnel: w1612 -> [w1618 w1620]
                  tunnel: [w1617 w1619] -> w1603
                  frame #0 {
                    n1426 = local read "Detektionskamera"() -> (w1617:T5)
                  }
                  frame #1 {
                    n1427 = local read "Ereignis: FrameDone?"() -> (w1622:refnum<event-registration>)
                    n1428 = local read "Detektionskamera"() -> (w1623:T5)
                    n1429 = call "camera_release_configuration.vi"("error in"=w1620, "Session In"=w1623, "Ereignisregistrierung (Referenz) 2"=w1622) -> ("error out"=w1621:errorcluster, "Session Out"=w1619:T5)
                  }
                }
                n1430 = local read "# Bilder/Messschritt"() -> (w1610:i32)
                n1431 = call "camera_acquisition_sequence.vi"("Session In"=w1603, "Desired image number"=w1610, "error in"=w1604) -> ("Session Out"=w1602:T5, "Image Array"=w1611:T4[], "error out"=w1609:errorcluster)  [unwired: 1 in]
                n1432 = local read "Buffer Interval"() -> (w1607:u32)
                n1433 = call "save images.vi"("Save Folder"=w1601, "File name prefix"=w1597, "Array"=w1611, "error out 2"=w1609, "Bilder/Messschritt"=w1610) -> ("error out"=w1606:errorcluster)
                n1434 = call "camera_create_configuration.vi"("error in"=w1606, "BufferInterval"=w1607, "Session Out 2"=w1602) -> ("Fehler (Ausgang)"=w1600:errorcluster, "Session Out"=w1605:T5, "Ereignisregistrierung (Referenz)"=w1608:refnum<event-registration>)
                n1435 = local write "Ereignis: FrameDone?"(w1608) -> ()
                n1436 = local write "Detektionskamera"(w1605) -> ()
                n1437 = local write "Fehler (Ausgang)"(w1600) -> ()
                n1438 = Unbundle By Name(w1600) -> ("status"=w1596:bool)
                n1439 = local write "Sequenzaufnahme ON"(w1596) -> ()
              }
            }
          }
        }
        n1440 = local read "Fehler (Ausgang)"() -> (w669:errorcluster)
        n1441 = local read "Programm beenden"() -> (w667:bool)
        n1442 = Unbundle By Name(w669) -> ("status"=w668:bool)
        n1443 = Or(x=w668, y=w667) -> (x .or. y?=w664:bool)
        "Scanschleifenzähler" <- w665
      }
    }
    frame #2 {
      n1444 = flat-sequence {
        frame #0 {
          n1445 = local read "Kamera"() -> (w1704:bool)
          n1446 = case shown="True" w1704 {
            frame #0 {
            }
            frame #1 {
              n1447 = local read "Detektionskamera"() -> (w1706:T5)
              n1448 = local read "Image Memory"() -> (w1708:T4)
              n1449 = call "camera_release configuration_stop.vi"("Image Memory"=w1708, "Detektionskamera"=w1706) -> ("error out"=w1705:errorcluster, "status"=w1707:bool)
              n1450 = local write "Kamera"(w1707) -> ()
              n1451 = local write "Fehler (Ausgang)"(w1705) -> ()
            }
          }
        }
        frame #1 {
          # "Wegen Abstürzen des Programms wird dieser Teil verhindert\nAchtung: IMMER manuell Netzteile auf 0V setzen oder HV-\nSteuerung von Hand ausmachen"
          n1452 = local read "HV-Steuerung"() -> (w1711:bool)
          n1453 = And(x=w1711, y=FALSE) -> (x .and. y?=w1709:bool)
          n1454 = case shown="True" w1709 {
            frame #0 {
            }
            frame #1 {
              n1455 = call "HV_power_supply_set_voltage.vi"("Desired output voltage in V (HV power supply)"=0.0, "Channel of HV power supply"=refnum<k21> "Dev0/Ao1") -> ("error out"=w1712:errorcluster)  [unwired: 8 in]
              n1456 = call "HV_power_supply_set_voltage.vi"("Desired output voltage in V (HV power supply)"=0.0, "Channel of HV power supply"=refnum<k21> "Dev0/Ao0") -> ("error out"=w1713:errorcluster)  [unwired: 8 in]
              n1457 = local write "Fehler (Ausgang)"(w1712) -> ()
              n1458 = local write "Fehler (Ausgang)"(w1713) -> ()
            }
          }
        }
        frame #2 {
          n1459 = local read "Wellenplatte"() -> (w1718:bool)
          n1460 = case shown="True" w1718 {
            frame #0 {
            }
            frame #1 {
              n1461 = local read "Wellenplatte [°]"() -> (w1719:refnum<k7>)
              n1462 = invoke class="MG17Motor" method="StopCtrl"(reference=w1719) -> ()  [unwired: 2 in, 3 out]
            }
          }
        }
        frame #3 {
          w1720 = FALSE ("Bühne bereit")
          w1721 = 0.0 ("Suppressor-Spannung [V]")
          n1463 = local write "Tip-Spannung [V]"(w1721) -> ()
          n1464 = local write "Suppressor-Spannung [V]"(w1721) -> ()
          n1465 = local write "Bühne"(w1720) -> ()
          n1466 = local write "Leistungs-/Polarisationsscan ON/OFF"(w1720) -> ()
          n1467 = local write "Spannungsscan läuft"(w1720) -> ()
          n1468 = local write "HV-Steuerung"(w1720) -> ()
          n1469 = local write "Waveplate ON/OFF"(w1720) -> ()
          n1470 = local write "x-U-Scan ON/OFF"(w1720) -> ()
          n1471 = local write "Kamera ON/OFF"(w1720) -> ()
          n1472 = local write "Wellenplatte"(w1720) -> ()
          n1473 = local write "x-U-Scan läuft"(w1720) -> ()
          n1474 = local write "Leistungs-/Polarisationscan läuft"(w1720) -> ()
        }
      }
    }
  }
